vi "AlliGator Settings Storage.vi"(6 "Get(F)/Set":bool, 7 "AlliGator Settings List":T1=enum."Source Image:Use Image Histogram for Contrast", 8 "Error In":errorcluster, 11 "Variant Data in":variant) -> (0 "Error Out":errorcluster, 3 "Variant Data out":variant)   [LabVIEW 2021, in "AlliGator Settings.lvlib"]
doc: "Get/Set Settings parameter values using variant attributes."
uses:
  AlliGator Settings.lvlib
  Phasor/Phasor Explorer Gate Parameters.ctl
  Phasor/Phasor Gate Type.ctl
  Phasor/Phasor Type of User-defined Function.ctl
  Phasor/Phasor Explorer Decay Parameters.ctl
  Phasor/Phasor IRF Model.ctl
  Phasor/Phasor Explorer Phasor Parameters.ctl
  Phasor/Phasor Calculation Type.ctl
  Phasor/Phasor SEPL Type.ctl
  Phasor/Phasor Explorer Display Parameters.ctl
  Phasor/Phasor Type of Series.ctl
  Image/Image Save File Format.ctl
  Phasor Plot/AlliGator Phasor Plot Size.ctl
  AlliGator Background Subtraction Parameters.ctl
  Graphs/XY Graph/XY Graph Plot Shift Parameters.ctl
  Graphs/XY Graph/XY Graph Plot Shift Method.ctl
  Fits/IRF(X)PSED/IRF(X)PSED Extraction Options.ctl
  Fits/IRF(X)PSED/Fourier Series Smoothing Option.ctl
  Fits/IRF(X)PSED/Fourier Series Truncation.ctl
  Fits/IRF(X)PSED/IRF Extraction Method.ctl
  AlliGator Settings List.ctl
  AlliGator Low Count Pixels Rejection Options.ctl
  Phasor/Phasor Ratio Type.ctl
  Decay Analysis/Decay Preprocessing/AlliGator Baseline Subtraction Method.ctl
  Fits/Decay Convolution/Decay Model.ctl
  Fits/Residual Type.ctl
  Fits/Non-linear Fitting Method v2.ctl
  Fits/Fit Calculation Method.ctl
  Fits/Non-linear Fitting Algorithm.ctl
  Fits/IRF(X)PSED/Decay Fit Parameters & Derived Quantities List v2.ctl
  Decay Analysis/Decay Fit/AlliGator Decay Fit Parameter Constraints 2.ctl
  Fits/IRF(X)PSED/Decay Fit Parameters In List.ctl
  Decay Analysis/IRF/AlliGator IRF Optimization Controls.ctl
  Decay Analysis/IRF/AlliGator IRF Deconvolution Metrics.ctl
  Math/Advanced Signal Processing Toolkit/Wavelet Analysis Options.ctl
  AlliGator High Count Pixels Rejection Options.ctl
  AlliGator Image Smoothing Options.ctl
  Arrays/Kernel Type.ctl
  Arrays/Smoothing Algorithm.ctl
  Fits/Square Pulse/Square Pulse Options.ctl
  Fits/Square Pulse/Square Pulse Levels Type.ctl
  Source Image/AlliGator Image Binning Options.ctl
  Phasor Plot/AlliGator Phasor Plot Smoothing Options.ctl
  AlliGator Phasor Plot Graphics Options.ctl
  AlliGator Exported Image Settings.ctl
  AlliGator Define Gates to.ctl
  AlliGator Gates to Keep.ctl
  Phasor Ratio/AlliGator Phasor Ratio Color-Coded Quantity.ctl
  Phasor/Phasor Calibration Type.ctl
  Histograms/Linear Histogram Options.ctl
  Histograms/Histogram Bin Option.ctl
  Histograms/Histogram Bin Position.ctl
  AlliGator Gate Arithmetic.ctl
  Phasor Ratio/AlliGator Phasor Reference Associated with Shortest Lifetime.ctl
  AlliGator Python Settings.ctl
  SwissSPAD/SwissSPAD Live_Image Display Options.ctl
  AlliGator Average Lifetime Options.ctl
  Phasor Calibration/AlliGator Calibration Map Algorithm.ctl
  Decay Analysis/Decay Fit/AlliGator Guess Parameters Options.ctl
  Phasor/Phasor Standard Deviation Options.ctl
  Source Image/AlliGator Source Image Scale Bar Options.ctl
  Fits/IRF(X)PSED/MLE Baseline Offset Type.ctl
  Image/Flatfield Correction Options.ctl
  Fits/Optimal Offset Selection Criterion.ctl
  Fits/IRF(X)PSED/Decay Fit Options v2.ctl
  Fits/IRF(X)PSED/Decay Fit Options v1.ctl
  Fits/Non-linear Fitting Method v1.ctl
  Graphs/XY Graph/XY Graph Plot Data.ctl
  Phasor/Phasor User-defined Gate & IRF.vi
  Graphs/XY Graph/XY Graph Add-Ons.lvlib
  Phasor/Phasor.lvlib
  Utilities/Utilities.lvlib
  Fits/Fits.lvlib
  Fits/IRF(X)PSED/Fit Weights Type.ctl
  Fits/IRF(X)PSED/Decay Fit Options v3.ctl
  Phasor Plot/AlliGator Phasor Plot.lvlib
  Image/Image.lvlib
  Decay Analysis/Decay Preprocessing/AlliGator Decay Preprocessing.lvlib
  Decay Analysis/Decay Fit/AlliGator Decay Fit.lvlib
  Decay Analysis/IRF/AlliGator IRF.lvlib
  Math/Math.lvlib
  Arrays/Arrays.lvlib
  Source Image/AlliGator Source Image.lvlib
  Phasor/Phasor Explorer.lvlib
  Phasor Ratio/AlliGator Phasor Ratio.lvlib
  Histograms/Histogram Window.lvlib
  SwissSPAD/SwissSPAD Live.lvlib
  Phasor Calibration/AlliGator Phasor Calibration.lvlib
  Fits/IRF(X)PSED/Fit Weights Type v2.ctl
  Fits/IRF(X)PSED/Decay Fit Options v4.ctl
panel:
  in  "Show Dead Left Columns Correction":bool
  in  "Tab Control":T2(tab)
  in  "Source ImageTab":T3(tab)
  in  "Use Image Histogram for Contrast":bool=TRUE
  in  "Low Count Pixels Rejection Options":T4={"Background Low Threshold Factor"=0.0, "Fixed Low Background Threshold"=20000.0, "Reject Low Count Pixels"=FALSE, "Low Percentile"=0.0} {"Low Percentile" min=0.0 max=100.0}
  in  "High Count Pixels Rejection Options":T5={"Background High Threshold Factor"=0.0, "Fixed High Background Threshold"=20000.0, "Reject High Count Pixels"=FALSE, "High Percentile"=100.0} {"High Percentile" min=0.0 max=100.0}
  in  "Hot Pixel Removal":T6 {"Percentile" min=0 max=100}
  in  "Dead Left Columns Correction":bool
  in  "Use Fixed ROI Diameter":bool
  in  "ROI Diameter":i32=12
  in  "ROI Center Color":u32(colorbox)=16711680
  in  "Image Binning Options":T7={"Use Image Binning"=FALSE, "X Bin"=1, "Y Bin"=1} {"Y Bin" min=1; "X Bin" min=1}
  in  "Flatfield Correction":T8={"Flatfield Estimation Options"={"Sampling Grid Size X"=256, "Sampling Grid Size Y"=256, "Polynomial Degree"=5}, "Background Options"={"Estimate Background"=TRUE, "Background Estimation Size"=32, "Niblack Deviation Factor [0. 1]"=0.2}, "Correction Factor"=1.1} {"Background Options"."Niblack Deviation Factor [0. 1]" min=0.0 max=1.0}
  in  "Image Smoothing Options":T9={"Use Image Smoothing"=FALSE, "Kernel Type"=enum."Bilinear", "Bin"=500, "Algorithm"=enum."Rapid"} {"Bin" min=1}
  in  "Peak Threshold":dbl=500.0
  in  "Intensity Threshold":dbl=500.0
  in  "Invert Binary Mask":bool
  in  "Image Pre-Processing Operations Order":string[](array[string]) caption="Order"
  in  "Median Overlay Color":u32(colorbox)
  in  "Overlay ROI Median":bool=TRUE caption="Use Image Brightness"
  in  "Image Resolution (Pixel Size)":dbl[unit]
  in  "Scale Bar Options":T12 caption="Scale Bar Options (*)"
  in  "Overlay Analyzed ROI Center":bool
  in  "Use Image Brightness":bool=TRUE
  in  "Blend Overlay with Image Background":bool=TRUE
  in  "Dataset Scaling Factor":dbl=1.0 caption="Scaling Factor" min=0.0
  in  "Gate Image Integration":dbl[unit]=3e-10 min=0.0 format="%#.3g"
  in  "Gate Image Exposure":dbl[unit]=3e-10 min=0.0 format="%#.3g"
  in  "Background File Subtraction":bool
  in  "Background Scaling Factor":dbl=1.0 caption="Scaling Factor"
  in  "Background File":path
  in  "Background Pile-up Correction":bool caption="Pile-up Correction"
  in  "Background Pixel Well Capacity":u32=1 caption="Max Value" min=1 step=1
  in  "Channel Arithmetic":T13
  in  "Available Gate Names":string[](array[string])
  in  "Channel Name":u16(ring) items=["Gate"]
  in  "Gates to Keep":T14 caption="Gates to Keep (*)"
  in  "Define Gates to":T15
  in  "Laser Period":dbl[unit] format="%#_3g"
  in  "Gates to Skip":T16
  in  "Gate Separation":dbl[unit]=4e-11
  in  "Gate Width":dbl[unit]=3e-10
  in  "Gate Step":i32=1 min=1
  in  "Pile-up Correction":bool
  in  "Pixel Well Capacity":i32=1 min=1
  in  "# Gates":u32=1 min=1 step=1
  in  "SYNC Period":dbl[unit] caption="IRF Period" min=0.0 format="%#_3g"
  in  "Mscrotime Gate Separation":dbl[unit]=1.0 min=0.0
  in  "Decay Tabs":T17(tab)
  in  "# Folds":u32=1 min=1
  in  "Fold Decay":bool caption="Straighten Decay"
  in  "Use Decay Pre-Processing":bool=TRUE
  in  "Head Fraction":dbl min=0.0 max=1.0
  in  "Use Cursors":bool
  in  "Use Periodicity":bool
  in  "Pixel-Normalize Decay":bool
  in  "Verbose Decay Pre-Processing":bool=TRUE caption="Verbose Devay Pre-Processing"
  in  "Straighten Decay":bool
  in  "Reverse Gates":bool caption="Revert Gates"
  in  "Additional Points":u32 caption="Gate Duration"
  in  "Tail Fraction":dbl caption="Gate Duration" min=0.0 max=1.0
  in  "Extrapolate Decay":bool
  in  "Baseline Subtraction Method":T18=enum."Min" caption="Method"
  in  "Background Definition Range":T19={"Min Gate"=0.0, "Max Gate"=8e-10}
  in  "Decay Shift Parameters":T20
  in  "Shift Decay":bool
  in  "Smoothen Decay":bool caption="Smooth Decay"
  in  "Smoothing Parameter":dbl caption="Gate Duration" min=0.0 max=1.0
  in  "1-Normalize Decay":bool
  in  "Background Subtraction":bool=TRUE
  in  "Constant Background":dbl=1.0
  in  "Decay Pre-Processing Operations Order":string[](array[string]) caption="Order"
  in  "[0-1]-Normalize Decay":bool caption="1- Normalize Decay"
  in  "Average Lifetime Options":T22={"Use Local IRF "=TRUE, "Use IRF Offset"=TRUE, "Use Fixed Offset"=TRUE, "Fixed Offset"=0.0, "Baseline %"=0.0} caption="Use Local IRF" {"Baseline %" min=0.0 max=100.0}
  in  "IRF Time Constants":dbl[](array[numeric])
  in  "IRF order":i32
  in  "Square Pulse Options":T23={"Method"=enum."Mode", "# Bins"=0, "Threshold %"=10.0, "Center on Midpoint"=FALSE, "Smoothen Plot"=FALSE} {"Threshold %" min=0.0 max=100.0}
  in  "Wavelet Analysis Options":T25={"Wavelet"=enum."db02", "Option for Approximate Coefficients"=enum."None", "# Levels"=1, "Threshold Settings"={"Thresholding Rule"=enum."Universal", "Rescaling Method"=enum."Single level", "Soft Threshold?"=TRUE}, "Wavelet Transform Type"=enum."Discrete"}
  in  "Time Constant for IRF Extraction":T26={"Time Constant for IRF Extraction"=1e-18, "IRF Order"=1, "Fourier Series Smoothing"=enum."None", "Noise Threshold"=0.0, "Smoothing Width"=0.0, "Fourier Series Truncation"=enum."Automatic", "Truncation Order"=0, "Save Power Spectrum"=FALSE, "Smoothing"=FALSE, "Smoothing Parameter"=0.0, "Smoothing Order"=1, "Method"=enum."Direct"} caption="Gate Duration" {"Smoothing Order" min=1 max=10; "Time Constant for IRF Extraction" format="%#_5g"}
  in  "Extract IRF instead of Decay":bool
  in  "IRF Optimization Options":T30={"Search Range"=1e-18, "Search Step"=1e-09, "Tail Threshold (%)"=1e-09, "Regularized IRF"=FALSE, "Export Plot"=FALSE, "Export Data"=FALSE, "Smooth Metrics"=FALSE, "S-G Side Points"=1, "S-G Polynomial Order"=3, "Metrics"=enum."Average"} {"S-G Polynomial Order" min=3 max=10; "S-G Side Points" min=1; "Search Range" min=0.0 max=1e-09}
  in  "Use Data Information Laser Period":bool
  in  "Use Legagy Fitting Approach":bool
  in  "Fit Options":T32={"Show Fit Residuals"=TRUE, "Fit Model"=enum."1-Exponential", "Residual Type"=enum."Standard", "Max Decay Percentile"=0.0, "Min Decay Percentile"=0.0, "Show Full Decay"=TRUE, "Weights"=enum."Unweighted", "Fitting Method"=enum."Least Square", "Compute Parameter Uncertainties"=TRUE, "Periodic Boundaries"=TRUE, "Model Calculation"=enum."Simulation", "Period"=1.2500000000000001e-08, "Termination Criteria"={"Max Iterations"=1000, "Max Function Calls"=0, "Max Time"=1000.0, "Function Tolerance"=1e-06, "Parameter Tolerance"=1e-06, "Gradient Tolerance"=0.0, "Min Lambda"=1e-06, "Max Lambda"=1e-06, "Initial Tick Count"=0}, "Offset Resolution"=1.2500000000000001e-08, "Use Local IRF"=TRUE, "Fitting Algorithm"=enum."Levenberg-Marquardt", "Show Confidence Interval "=TRUE, "Confidence Level"=95.0} {"Confidence Level" min=0.0 max=100.0; "Offset Resolution" min=0.0; "Period" min=0.0; "Min Decay Percentile" min=0.0 max=1.0; "Max Decay Percentile" min=0.0 max=100.0}
  in  "Optimal Offset Selection Criterion":T39
  in  "MLE Baseline Offset Type":T40
  in  "MLE Baseline Offset":dbl
  in  "Guess Parameters Options":T41 caption="Options"
  in  "Guess Parameters Names":T42[](array[typedef])
  in  "Guess Parameter Values":dbl[](array[numeric]) caption="Guess Parameters"
  in  "Fit Parameter Constraints":T43[](array[typedef]) {"Max Value" format="%#.3g"; "Min Value" format="%#.3g"}
  in  "Displayed Fit Parameters":T44[](array[typedef])
  in  "Export Tabulated Results":bool=TRUE
  in  "Decay Graph Color Array":u32[](array[colorbox])
  in  "Show Last Decay only":bool
  in  "Max Peak Value":dbl
  in  "Reject High Decay Peak Pixels":bool
  in  "Min Peak Value":dbl
  in  "Reject Low Decay Peak Pixels":bool
  in  "Intensity Correction File":path
  in  "Use Intensity Correction File":bool
  in  "Use File Timestamp":bool
  in  "Time Step":dbl[unit]=1.0
  in  "Intensity-weighted Phasor Plot":bool caption="Cumulative Phasor Plot"
  in  "Low Color":u32(colorbox)
  in  "High Color":u32(colorbox)
  in  "User-defined Quantity":string
  in  "Blend Overlay with Phasor Background":bool=TRUE
  in  "Draw Reference Segment":bool
  in  "Store Phasor Harmonics":bool
  in  "All Phasor Plot ROIs":bool
  in  "Selected Phasor Plot ROI(s)":bool
  in  "Phasor Ratio Color-Coded Quantity":T45 caption="Displayed Quantity"
  in  "All Image ROIs":bool
  in  "Selected Image ROI(s)":bool
  in  "Reference Radius":i32=512
  in  "Phasor Ratio Display Range":cluster{dbl, dbl}(slide)={0.0, 454.0} scale=0.0..1.0
  in  "Phasor Plot Graphics Options":T46={"UC Color"=3381759, "Show UC Tau Ticks"=FALSE, "SEPL Color"=3381759, "Show SEPL Tau Ticks"=FALSE, "Axes Color"=16776960, "Show (g,s) Ticks"=FALSE, "Show UC"=FALSE, "Show SEPL"=FALSE, "Show Axes"=FALSE, "Show UC Tau Labels"=FALSE, "Show SEPL Tau Labels"=FALSE, "Show (g,s) Labels"=FALSE, "UC Label Size"=18, "UC Label Distance"=0.0, "SEPL Label Size"=18, "SEPL Label Distance"=0.0, "Axes Label Size"=18, "Axes Label Distance"=0.0}
  in  "Phasor Plot Smoothing Options":T47={"Use Phasor Plot Smoothing"=FALSE, "Kernel Type"=enum."Uniform", "Bin"=1, "Algorithm"=enum."Rapid"} {"Bin" min=1 step=2}
  in  "Phasor Ratio Color Map":string
  in  "Phasor Ratio Color Map Type":T48(radio)
  in  "Show Color Map Vertices":bool=TRUE
  in  "Exponential Fading":bool
  in  "Phasor Ratio Reference Colors":T49={"Reference 1"=3381759, "Reference 2"=3381759, "Boundary"=3381759}
  in  "Phasor Ratio Decay Range":dbl=1.0
  in  "Show References":bool
  in  "Save Phasor Plot":bool
  in  "Cumulative Phasor Plot":bool
  in  "Phasor Plot Size":T50={"H"=512, "V"=512, "Margin"=0.2} {"Margin" min=0.0}
  in  "Use Phasor Brightness":bool
  in  "Intensity-weighted Phasor Graph":bool
  in  "Phasor SDV Options":T51={"Compute Estimated SDV"=FALSE, "# Replicas"=100, "Use Estimated Average Phasor"=FALSE}
  in  "Define Shortest Lifetime as":T52
  in  "Save Phasor Graph Image":bool
  in  "Pixel-level Phasor Computation":bool
  in  "Phasor Ratio Type":T53
  in  "Phasor Frequency":dbl[unit]=160000000.0
  in  "Phasor Graph Active":bool caption="Save Phasor Graph Image"
  in  "SEPL Tabs":enum32{"Display", "Phasor", "IRF", "Gates"}(tab)
  in  "SEPL Display Parameters":T54={"# Points"=1000, "Ramp Type"=enum."Logarithmic", "Type of Series"=enum."1-Exp Decays", "Min tau"=1.0000000000000002e-12, "Max tau"=1.0000000000000001e-07, "Include 0"=FALSE, "Include Infinity"=FALSE} {"Min tau" min=0.0; "Max tau" min=0.0; "# Points" min=1 step=1}
  in  "SEPL Phasor Parameters":T56={"Harmonic Frequency"=0.0, "Use f* = 1/D Frequency"=FALSE, "Calibrated Phasor"=FALSE, "Calibration Lifetime"=1e-09, "Phasor Calculation"=enum."Direct Sum", "SEPL Type"=enum."UC", "# Gates"=1.0, "Square Gate Width"=1e-09, "Show Ticks"=FALSE} {"Square Gate Width" min=0.0; "# Gates" min=0.0; "Calibration Lifetime" min=0.0; "Harmonic Frequency" min=0.0}
  in  "SEPL IRF Parameters":T59={"Lifetime"=3.0000000000000004e-09, "IRF Offset"=0.0, "IRF Period"=1.2500000000000001e-08, "Normalized Decays"=FALSE, "IRF Model"=enum."Dirac", "IRF Parameter 1"=0.0} {"Lifetime" min=0.0; "IRF Period" min=0.0}
  in  "SEPL Gate Parameters":T61={"First Gate Start"=0.0, "Use Gate Center"=FALSE, "Gate Width"=0.0, "Gate Step"=0.0, "# Gates"=1.0, "Gate Type"=enum."Square", "Edge Width"=0.0, "Top Slope"=0.0, "Reversed Sawtooth?"=FALSE, "Analytical Computation"=FALSE, "Integration"=enum."Item 0", "Tolerance"=1.0, "# Steps"=1.0, "Type of User-defined Function"=enum."Gate", "Use Gate Step"=FALSE} {"# Steps" min=0.0; "Tolerance" min=0.0; "Top Slope" min=0.0; "Edge Width" min=0.0; "Gate Step" min=0.0; "# Gates" min=1.0 step=1.0; "Gate Width" min=0.0}
  in  "Calibration Map Algorithm":T64
  in  "Calibration Type":T65=enum."Single Phasor"
  in  "Use Backup Calibration if needed":bool=TRUE
  in  "Backup Calibration Type":T66(ring) caption="Backup Calibration"
  in  "Calibration Lifetime":dbl[unit]=1e-09
  in  "Decay Analysis Parameters":T20
  in  "Python Settings":T67
  in  "Transparent Mask Color":u32(colorbox)
  in  "ROI Description Max Characters":i32=256
  in  "Beep on Error":bool caption="Verbose Error Mode"
  in  "# Logical Processors Used":i32 caption="Used" min=1 max=16
  in  "Histogram Options":T68={"Bin Size"=0.0, "Bin Number"=0, "Bin Option"=enum."Bin Number", "Min Value"=-inf, "Max Value"=inf, "Filter NaN & Infinite Values"=TRUE, "Frequency Plot"=FALSE, "Align Bins"=FALSE, "Bin Location"=enum."Left", "Project Outside Values"=FALSE, "Max Histogram Size"=100000} {"Max Histogram Size" format="%.0e"}
  in  "Exported Gate Image Settings":T71
  in  "Verbose Error Mode":bool
  in  "Verbose Settings Mode":bool
  in  "Beep after Script":bool
  in  "Verbose Mode":bool
  in  "Saved Displayed Image File Format":T72
  in  "Visible Settings Tab":string caption="Settings Tab List"
  in  "Include Loading in Timing":bool
  in  "Last Run Version":string
  # "see the AlliGator License on the block diagram (Ctrl+E or Window:Show Block Diagram)"
  # "Gates Characteristics"
  # "Limit Phasor Plot Analysis  to:"
  # "Lifetime Analysis Options"
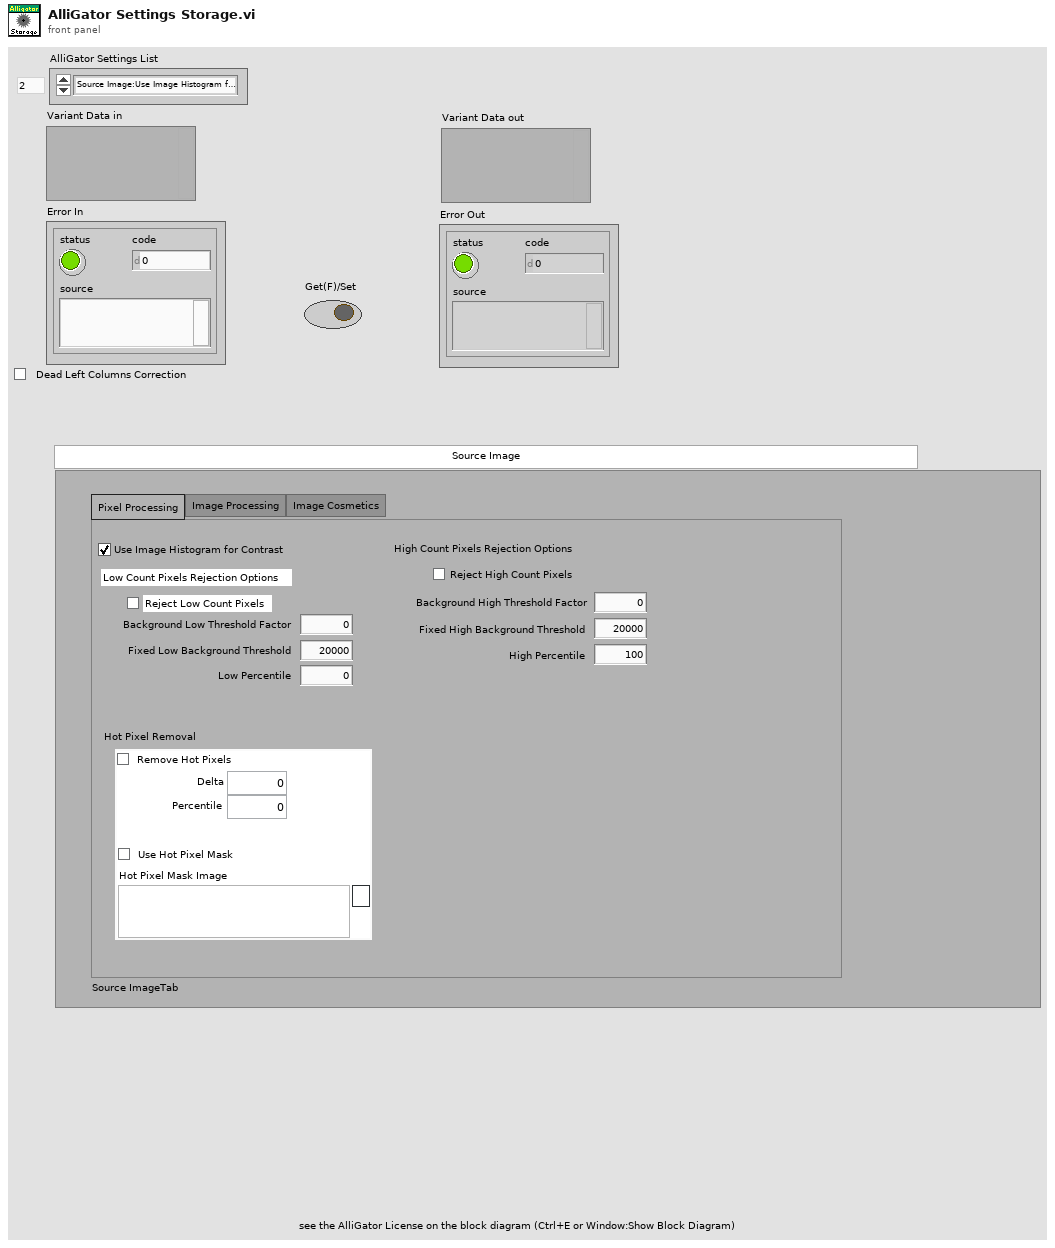
[diagram p1: front panel]
types:
  T1 = typedef "AlliGator Settings.lvlib/AlliGator Settings List.ctl" = enum16{"GUI:Visible Settings Tab", "GUI:Last Run Version", "Source Image:Use Image Histogram for Contrast", "Source Image:Low Count Pixels Rejection Options", "Source Image:High Count Pixels Rejection Options", "Source Image:Use Image Brightness", "Source Image:Blend Overlay with Image Background", "Source Image:Use Fixed ROI Diameter", "Source Image:ROI Diameter", "Source Image:ROI Center Color", "Source Image:Peak Threshold", "Source Image:Intensity Threshold", "Source Image:Image Binning Options", "Source Image:Image Smoothing Options", "Source Image:Image Histogram Active", "Source Image:Invert Binary Mask", "Source Image:Hot Pixel Removal", "Source Image:Overlay Analyzed ROI Center", "Source Image:Auto-Adjust Contrast", "Source Image:Histogram Lower Percentile", "Source Image:Histogram Upper Percentile", "Source Image:Save Source Image", "Source Image:Scale Bar Options", "Source Image:Image Resolution (Pixel Size)", "Source Image:Flatfield Correction", "Source Image:Show Dead Left Columns Correction", "Source Image:Dead Left Columns Correction", "Source Image:Image Pre-Processing Operations Order", "Source Image:Overlay ROI Median", "Source Image:Median Overlay Color", "Data Information:Gate Width", "Data Information:Nanotime Gate Separation", "Data Information:Macrotime Gate Separation", "Data Information:Gate Step", "Data Information:# Gates", "Data Information:Gate Image Exposure", "Data Information:Gate Image Integration", "Data Information:Gates to Skip", "Data Information:Gates to Keep", "Data Information:Define Gates to", "Data Information:Channel Name", "Data Information:Available Channel Names", "Data Information:Channel Arithmetic", "Data Information:Background File Subtraction", "Data Information:Background File", "Data Information:Background Scaling Factor", "Data Information:Background Pile-up Correction", "Data Information:Background Pixel Well Capacity", "Data Information:Laser Period", "Data Information:SYNC Period", "Data Information:Pile-up Correction", "Data Information:Pixel Well Capacity", "Data Information:Dataset Scaling Factor", "Fluorescence Decay_Decay Pre-Processing:Reverse Gates", "Fluorescence Decay_Decay Pre-Processing:Verbose Decay Pre-Processing", "Fluorescence Decay_Decay Pre-Processing:Use Decay Pre-Processing", "Fluorescence Decay_Decay Pre-Processing:Background Subtraction", "Fluorescence Decay_Decay Pre-Processing:Background Definition Range", "Fluorescence Decay_Decay Pre-Processing:Baseline Subtraction Method", "Fluorescence Decay_Decay Pre-Processing:Decay Pre-Processing Operations Order", "Fluorescence Decay_Decay Pre-Processing:Smoothing Parameter", "Fluorescence Decay_Decay Pre-Processing:Shift Decay", "Fluorescence Decay_Decay Pre-Processing:Decay Shift Parameters", "Fluorescence Decay_Decay Pre-Processing:Fold Decay", "Fluorescence Decay_Decay Pre-Processing:# Folds", "Fluorescence Decay_Decay Pre-Processing:1-Normalize Decay", "Fluorescence Decay_Decay Pre-Processing:[0-1]-Normalize Decay", "Fluorescence Decay_Decay Pre-Processing:Smoothen Decay", "Fluorescence Decay_Decay Pre-Processing:Extrapolate Decay", "Fluorescence Decay_Decay Pre-Processing:Use Periodicity", "Fluorescence Decay_Decay Pre-Processing:Use Cursors", "Fluorescence Decay_Decay Pre-Processing:Tail Fraction", "Fluorescence Decay_Decay Pre-Processing:Head Fraction", "Fluorescence Decay_Decay Pre-Processing:Additional Points", "Fluorescence Decay_Decay Pre-Processing:Straighten Decay", "Fluorescence Decay_Decay Pre-Processing:Constant Background", "Fluorescence Decay_Decay Pre-Processing:Pixel-Normalize Decay", "Fluorescence Decay_Advanced Analysis:Extract IRF instead of Decay", "Fluorescence Decay_Advanced Analysis:IRF Extraction Options", "Fluorescence Decay_Advanced Analysis:IRF Optimization Options", "Fluorescence Decay_Advanced Analysis:Square Pulse Options", "Fluorescence Decay_Advanced Analysis:IRF Order", "Fluorescence Decay_Advanced Analysis:IRF Time Constants", "Fluorescence Decay_Advanced Analysis:Wavelet Analysis Options", "Fluorescence Decay_Advanced Analysis:Average Lifetime Options", "Fluorescence Decay_Fit Options:Fit Options", "Fluorescence Decay_Fit Options:Use Legacy Fitting Approach", "Fluorescence Decay_Fit Options:Use Data Information Laser Period", "Fluorescence Decay_Fit Parameters:Displayed Fit Parameters", "Fluorescence Decay_Fit Parameters:Fit Parameter Constraints", "Fluorescence Decay_Fit Parameters:Export Tabulated Results", "Fluorescence Decay_Fit Parameters:MLE Baseline Offset Type", "Fluorescence Decay_Fit Parameters:MLE Baseline Offset", "Fluorescence Decay_Fit Parameters:Guess Parameter Names", "Fluorescence Decay_Fit Parameters:Guess Parameter Values", "Fluorescence Decay_Fit Parameters:Guess Parameters Options", "Fluorescence Decay_Fit Parameters:Optimal Offset Selection Criterion", "Fluorescence Decay_Styles:Show Last Decay Only", "Fluorescence Decay_Styles:Decay Graph Color Array", "Fluorescence Decay:Decay Graph Active", "Fluorescence Decay Statistics:Min Peak Value", "Fluorescence Decay Statistics:Reject Low Decay Peak Pixels", "Fluorescence Decay Statistics:Reject High Decay Peak Pixels", "Fluorescence Decay Statistics:Max Peak Value", "Time Traces:Use File Timestamp", "Time Traces:Time Step", "Time Traces:Use Intensity Correction File", "Time Traces:Intensity Correction File", "Phasor Plot:Phasor Plot Smoothing Options", "Phasor Plot:Phasor Plot Size", "Phasor Plot:Phasor Plot Graphics Options", "Phasor Plot:Cumulative Phasor Plot", "Phasor Plot:Use Phasor Brightness", "Phasor Plot:Blend Overlay with Phasor Background", "Phasor Plot:Save Phasor Plot", "Phasor Plot:Show References", "Phasor Plot:Phasor Ratio Decay Range", "Phasor Plot:Exponential Fading", "Phasor Plot:Phasor Ratio Reference Colors", "Phasor Plot:Reference Radius", "Phasor Plot:Show Color Map Vertices", "Phasor Plot:Phasor Plot Active", "Phasor Plot:Phasor Ratio Color Map Type", "Phasor Plot:Phasor Ratio Color Map", "Phasor Plot:Phasor Ratio Display Range", "Phasor Plot:Selected Image ROI(s)", "Phasor Plot:All Image ROIs", "Phasor Plot:Selected Phasor Plot ROI(s)", "Phasor Plot:All Phasor Plot ROIs", "Phasor Plot:Phasor Ratio Color-Coded Quantity", "Phasor Plot:Store Phasor Harmonics", "Phasor Plot:Draw Reference Segment", "Phasor Plot:User-Defined Quantity", "Phasor Plot:Color Scale High Color", "Phasor Plot:Color Scale Low Color", "Phasor Plot:Intensity-weighted Phasor Plot", "Phasor Graph:Phasor Frequency", "Phasor Graph:Phasor Ratio Type", "Phasor Graph:Pixel-level Phasor Computation", "Phasor Graph:Save Phasor Graph", "Phasor Graph:Phasor Graph Active", "Phasor Graph:Phasor SDV Options", "Phasor Graph:Intensity-weighted Phasor Graph", "Phasor Graph:Define Shortest Lifetime as", "Phasor Calibration:Use Backup Calibration if needed", "Phasor Calibration:Backup Calibration Type", "Phasor Calibration:Calibration Type", "Phasor Calibration:Calibration Lifetime", "Phasor Calibration:Calibration Map Algorithm", "Single-Exponential Phasor Locus (SEPL):Gate Parameters", "Single-Exponential Phasor Locus (SEPL):User-defined Gate", "Single-Exponential Phasor Locus (SEPL):User-defined IRF", "Single-Exponential Phasor Locus (SEPL):Phasor Parameters", "Single-Exponential Phasor Locus (SEPL):Decay & IRF Parameters", "Single-Exponential Phasor Locus (SEPL):Display Parameters", "Lifetime Analysis:Decay Analysis Parameters", "Lifetime Analysis:Lifetime Map Active", "Plugins:Python Settings", "Miscellaneous:Verbose Mode", "Miscellaneous:Beep after Script", "Miscellaneous:Saved Image File Format", "Miscellaneous:Exported Gate Image Settings", "Miscellaneous:Include Loading in Timing", "Miscellaneous:Verbose Settings Mode", "Miscellaneous:Histogram Options", "Miscellaneous:Beep on Error", "Miscellaneous:# Logical Processors Used", "Miscellaneous:ROI Description Max Characters", "Miscellaneous:Verbose Error Mode", "Miscellaneous:Transparent Mask Color"}
  T2 = enum32{"Source Image", "Data Information", "Fluorescence Decay", "Fluorescence Decay Statistics", "Time Traces", "Phasor Plot", "Phasor Graph", "Single-Exponential Phasor Locus (SEPL)", "Phasor Calibration", "Lifetime Analysis", "Plugins", "Miscellaneous"}
  T3 = enum32{"Pixel Processing", "Image Processing", "Image Cosmetics"}
  T4 = typedef "AlliGator Settings.lvlib/AlliGator Low Count Pixels Rejection Options.ctl" = cluster{"Background Low Threshold Factor":dbl, "Fixed Low Background Threshold":dbl, "Reject Low Count Pixels":bool, "Low Percentile":dbl}
  T5 = typedef "AlliGator Settings.lvlib/AlliGator High Count Pixels Rejection Options.ctl" = cluster{"Background High Threshold Factor":dbl, "Fixed High Background Threshold":dbl, "Reject High Count Pixels":bool, "High Percentile":dbl}
  T6 = typedef "SwissSPAD Live.lvlib/SwissSPAD Live_Image Display Options.ctl" = cluster{"Remove Screamers":bool, "Delta":sgl, "Equalize Histogram":bool, "Percentile":sgl, "Hot Pixel Mask Image":path, "Use Hot Pixel Mask":bool}
  T7 = typedef "AlliGator Source Image.lvlib/AlliGator Image Binning Options.ctl" = cluster{"Use Image Binning":bool, "X Bin":i32, "Y Bin":i32}
  T8 = typedef "Image.lvlib/Flatfield Correction Options.ctl" = cluster{"Flatfield Estimation Options":cluster{"Sampling Grid Size X":i32, "Sampling Grid Size Y":i32, "Polynomial Degree":i32}, "Background Options":cluster{"Estimate Background":bool, "Background Estimation Size":i32, "Niblack Deviation Factor [0. 1]":dbl}, "Correction Factor":sgl}
  T9 = typedef "AlliGator Settings.lvlib/AlliGator Image Smoothing Options.ctl" = cluster{"Use Image Smoothing":bool, "Kernel Type":T10, "Bin":i32, "Algorithm":T11}
  T10 = typedef "Arrays.lvlib/Kernel Type.ctl" = enum16{"Uniform", "Bilinear", "Gaussian"}
  T11 = typedef "Arrays.lvlib/Smoothing Algorithm.ctl" = enum16{"Rapid", "Thorough"}
  T12 = typedef "AlliGator Source Image.lvlib/AlliGator Source Image Scale Bar Options.ctl" = cluster{"Show Scale Bar Overlay":bool, "Scale Bar Length":dbl[unit], "Scale Bar Color":u32, "Scale Bar X":u32, "Scale Bar Y":u32, "Scale Bar Height":dbl[unit]}
  T13 = typedef "AlliGator Settings.lvlib/AlliGator Gate Arithmetic.ctl" = enum16{"None", "INT-G2", "G2/INT*<INT>", "(1 - G2/INT)*<INT>"}
  T14 = typedef "AlliGator Settings.lvlib/AlliGator Gates to Keep.ctl" = cluster{"First":u32, "Last":u32}
  T15 = typedef "AlliGator Settings.lvlib/AlliGator Define Gates to.ctl" = enum32{"Skip", "Keep"}
  T16 = typedef "AlliGator Settings.lvlib/AlliGator Background Subtraction Parameters.ctl" = cluster{"Start":u32, "End":u32}
  T17 = enum32{"Decay Pre-Processing", "Advanced Analysis", "Fit Options", "Fit Parameters", "Styles"}
  T18 = typedef "AlliGator Decay Preprocessing.lvlib/AlliGator Baseline Subtraction Method.ctl" = enum16{"Mean", "Min", "Square Gated Single-Exponential", "File", "Constant"}
  T19 = cluster{"Min Gate":dbl[unit], "Max Gate":dbl[unit]}
  T20 = typedef "XY Graph Add-Ons.lvlib/XY Graph Plot Shift Parameters.ctl" = cluster{"Type":T21, "Shift":dbl[unit], "Threshold":dbl, "Rotate":bool}
  T21 = typedef "XY Graph Add-Ons.lvlib/XY Graph Plot Shift Method.ctl" = enum16{"Default", "CFD", "Threshold", "Cross-Correlation"}
  T22 = typedef "AlliGator Settings.lvlib/AlliGator Average Lifetime Options.ctl" = cluster{"Use Local IRF ":bool, "Use IRF Offset":bool, "Use Fixed Offset":bool, "Fixed Offset":dbl[unit], "Baseline %":dbl}
  T23 = typedef "Fits.lvlib/Square Pulse Options.ctl" = cluster{"Method":T24, "# Bins":i32, "Threshold %":dbl, "Center on Midpoint":bool, "Smoothen Plot":bool}
  T24 = typedef "Fits.lvlib/Square Pulse Levels Type.ctl" = enum16{"Mode", "Mean"}
  T25 = typedef "Math.lvlib/Wavelet Analysis Options.ctl" = cluster{"Wavelet":enum16{"db02", "db03", "db04", "db05", "db06", "db07", "db08", "db09", "db10", "db11", "db12", "db13", "db14", "Haar", "bior1_3", "bior1_5", "bior2_2", "bior2_4", "bior2_6", "bior2_8", "bior3_1", "bior3_3", "bior3_5", "bior3_7", "bior3_9", "bior4_4 (FBI)", "bior5_5", "bior6_8", "coif1", "coif2", "coif3", "coif4", "coif5", "sym2", "sym3", "sym4", "sym5", "sym6", "sym7", "sym8"}, "Option for Approximate Coefficients":enum16{"None", "Threshold", "Detrend"}, "# Levels":i32, "Threshold Settings":cluster{"Thresholding Rule":enum16{"SURE", "Hybrid", "Universal", "Minimax"}, "Rescaling Method":enum16{"One", "Single level", "Multiple levels"}, "Soft Threshold?":bool}, "Wavelet Transform Type":enum16{"Discrete", "Undecimated"}}
  T26 = typedef "Fits.lvlib/IRF(X)PSED Extraction Options.ctl" = cluster{"Time Constant for IRF Extraction":dbl[unit], "IRF Order":i32, "Fourier Series Smoothing":T27, "Noise Threshold":dbl, "Smoothing Width":dbl, "Fourier Series Truncation":T28, "Truncation Order":i32, "Save Power Spectrum":bool, "Smoothing":bool, "Smoothing Parameter":dbl, "Smoothing Order":u32, "Method":T29}
  T27 = typedef "Fits.lvlib/Fourier Series Smoothing Option.ctl" = enum16{"None", "Lanczos Factors", "Fejer Summation"}
  T28 = typedef "Fits.lvlib/Fourier Series Truncation.ctl" = enum16{"Automatic", "Fixed"}
  T29 = typedef "Fits.lvlib/IRF Extraction Method.ctl" = enum16{"Direct", "Topless", "Toeplitz"}
  T30 = typedef "AlliGator IRF.lvlib/AlliGator IRF Optimization Controls.ctl" = cluster{"Search Range":dbl[unit], "Search Step":dbl[unit], "Tail Threshold (%)":dbl, "Regularized IRF":bool, "Export Plot":bool, "Export Data":bool, "Smooth Metrics":bool, "S-G Side Points":i32, "S-G Polynomial Order":i32, "Metrics":T31}
  T31 = typedef "AlliGator IRF.lvlib/AlliGator IRF Deconvolution Metrics.ctl" = enum16{"Average", "SDV", "Max", "Average * SDV", "Slope"}
  T32 = typedef "Fits.lvlib/Decay Fit Options v4.ctl" = cluster{"Show Fit Residuals":bool, "Fit Model":T33, "Residual Type":T34, "Max Decay Percentile":dbl, "Min Decay Percentile":dbl, "Show Full Decay":bool, "Weights":T35, "Fitting Method":T36, "Compute Parameter Uncertainties":bool, "Periodic Boundaries":bool, "Model Calculation":T37, "Period":dbl[unit], "Termination Criteria":cluster{"Max Iterations":i32, "Max Function Calls":i32, "Max Time":dbl[unit], "Function Tolerance":dbl, "Parameter Tolerance":dbl, "Gradient Tolerance":dbl, "Min Lambda":dbl, "Max Lambda":dbl, "Initial Tick Count":u32}, "Offset Resolution":dbl[unit], "Use Local IRF":bool, "Fitting Algorithm":T38, "Show Confidence Interval ":bool, "Confidence Level":dbl}
  T33 = typedef "Fits.lvlib/Decay Model.ctl" = enum16{"1-Exponential", "2-Exponentials"}
  T34 = typedef "Fits.lvlib/Residual Type.ctl" = enum16{"Standard", "Normalized", "Reduced"}
  T35 = typedef "Fits.lvlib/Fit Weights Type v2.ctl" = enum16{"Unweighted", "1/Variance (Neyman)", "1/Variance (Pearson)", "Best of All"}
  T36 = typedef "Fits.lvlib/Non-linear Fitting Method v2.ctl" = enum16{"Least Square", "Least Absolute Residual", "Bisquare", "MLE", "-", "Best of All"}
  T37 = typedef "Fits.lvlib/Fit Calculation Method.ctl" = enum16{"Simulation", "Convolution", "Integration"}
  T38 = typedef "Fits.lvlib/Non-linear Fitting Algorithm.ctl" = enum16{"Levenberg-Marquardt", "Trust-Region Dogleg"}
  T39 = typedef "Fits.lvlib/Optimal Offset Selection Criterion.ctl" = enum16{"Min Chi^2", "Max R^2"}
  T40 = typedef "Fits.lvlib/MLE Baseline Offset Type.ctl" = enum32{"Absolute", "Percentage"}
  T41 = typedef "AlliGator Decay Fit.lvlib/AlliGator Guess Parameters Options.ctl" = enum16{"Numerically estimated", "User-provided", "User-provided (normalized)", "Last valid fitted parameters"}
  T42 = typedef "Fits.lvlib/Decay Fit Parameters In List.ctl" = enum16{"Offset", "Baseline", "A_1", "tau_1", "A_2", "tau_2"}
  T43 = typedef "AlliGator Decay Fit.lvlib/AlliGator Decay Fit Parameter Constraints 2.ctl" = cluster{"Fit Parameter":T42, "Min Value":dbl, "Max Value":dbl, "Global":bool, "Used":bool}
  T44 = typedef "Fits.lvlib/Decay Fit Parameters & Derived Quantities List v2.ctl" = enum16{"Offset", "Baseline", "A_1", "tau_1", "A_2", "tau_2", "<tau>_a", "f1_a", "f2_a", "<tau>_i", "f1_i", "f2_i", "-", "R^2", "Chi^2"}
  T45 = typedef "AlliGator Phasor Ratio.lvlib/AlliGator Phasor Ratio Color-Coded Quantity.ctl" = enum16{"Phasor Ratio (f1 or a1)", "Average Lifetime (<tau>_i or <tau>_a))", "User-Defined Quantity"}
  T46 = typedef "AlliGator Settings.lvlib/AlliGator Phasor Plot Graphics Options.ctl" = cluster{"UC Color":u32, "Show UC Tau Ticks":bool, "SEPL Color":u32, "Show SEPL Tau Ticks":bool, "Axes Color":u32, "Show (g,s) Ticks":bool, "Show UC":bool, "Show SEPL":bool, "Show Axes":bool, "Show UC Tau Labels":bool, "Show SEPL Tau Labels":bool, "Show (g,s) Labels":bool, "UC Label Size":i16, "UC Label Distance":dbl, "SEPL Label Size":i16, "SEPL Label Distance":dbl, "Axes Label Size":i16, "Axes Label Distance":dbl}
  T47 = typedef "AlliGator Phasor Plot.lvlib/AlliGator Phasor Plot Smoothing Options.ctl" = cluster{"Use Phasor Plot Smoothing":bool, "Kernel Type":T10, "Bin":i32, "Algorithm":T11}
  T48 = enum32{"Interpolate Reference Colors", "Use Custom Map"}
  T49 = cluster{"Reference 1":u32, "Reference 2":u32, "Boundary":u32}
  T50 = typedef "AlliGator Phasor Plot.lvlib/AlliGator Phasor Plot Size.ctl" = cluster{"H":i32, "V":i32, "Margin":dbl}
  T51 = typedef "Phasor.lvlib/Phasor Standard Deviation Options.ctl" = cluster{"Compute Estimated SDV":bool, "# Replicas":u32, "Use Estimated Average Phasor":bool}
  T52 = typedef "AlliGator Phasor Ratio.lvlib/AlliGator Phasor Reference Associated with Shortest Lifetime.ctl" = enum32{"Reference 1", "Reference 2"}
  T53 = typedef "Phasor.lvlib/Phasor Ratio Type.ctl" = enum32{"Intensity-weighted", "Amplitude-weighted"}
  T54 = typedef "Phasor Explorer.lvlib/Phasor Explorer Display Parameters.ctl" = cluster{"# Points":i32, "Ramp Type":enum16{"Linear", "Logarithmic"}, "Type of Series":T55, "Min tau":dbl[unit], "Max tau":dbl[unit], "Include 0":bool, "Include Infinity":bool}
  T55 = typedef "Phasor.lvlib/Phasor Type of Series.ctl" = enum16{"1-Exp Decays", "Linear Combination of 1-Exp"}
  T56 = typedef "Phasor Explorer.lvlib/Phasor Explorer Phasor Parameters.ctl" = cluster{"Harmonic Frequency":dbl[unit], "Use f* = 1/D Frequency":bool, "Calibrated Phasor":bool, "Calibration Lifetime":dbl[unit], "Phasor Calculation":T57, "SEPL Type":T58, "# Gates":dbl, "Square Gate Width":dbl[unit], "Show Ticks":bool}
  T57 = typedef "Phasor.lvlib/Phasor Calculation Type.ctl" = enum16{"Direct Sum", "Analytical Formula"}
  T58 = typedef "Phasor.lvlib/Phasor SEPL Type.ctl" = enum16{"UC", "L_N", "L_N[W]", "L_X"}
  T59 = typedef "Phasor Explorer.lvlib/Phasor Explorer Decay Parameters.ctl" = cluster{"Lifetime":dbl[unit], "IRF Offset":dbl[unit], "IRF Period":dbl[unit], "Normalized Decays":bool, "IRF Model":T60, "IRF Parameter 1":dbl[unit]}
  T60 = typedef "Phasor.lvlib/Phasor IRF Model.ctl" = enum16{"Dirac", "Exponential"}
  T61 = typedef "Phasor Explorer.lvlib/Phasor Explorer Gate Parameters.ctl" = cluster{"First Gate Start":dbl[unit], "Use Gate Center":bool, "Gate Width":dbl[unit], "Gate Step":dbl[unit], "# Gates":dbl, "Gate Type":T62, "Edge Width":dbl[unit], "Top Slope":dbl[unit], "Reversed Sawtooth?":bool, "Analytical Computation":bool, "Integration":enum32{"Item 0", "Item 1"}, "Tolerance":dbl, "# Steps":dbl, "Type of User-defined Function":T63, "Use Gate Step":bool}
  T62 = typedef "Phasor.lvlib/Phasor Gate Type.ctl" = enum16{"Square", "Finite Edge Square", "Finite Edge, Tilted Top Square", "Triangle", "Sawtooth", "User-defined"}
  T63 = typedef "Phasor.lvlib/Phasor Type of User-defined Function.ctl" = enum16{"Gate", "IRF"}
  T64 = typedef "AlliGator Phasor Calibration.lvlib/AlliGator Calibration Map Algorithm.ctl" = enum16{"Simple Search", "Min Distance"}
  T65 = typedef "Phasor.lvlib/Phasor Calibration Type.ctl" = enum16{"None", "Single Phasor", "Phasor Series", "Phasor Map"}
  T66 = enum16{"Single Calibration", "Nearest Valid Calibration"}
  T67 = typedef "AlliGator Settings.lvlib/AlliGator Python Settings.ctl" = cluster{"Python Version":string, "Use PATH definition":bool, "Python.exe Path":path, "Include Example Plugins":bool}
  T68 = typedef "Histogram Window.lvlib/Linear Histogram Options.ctl" = cluster{"Bin Size":dbl, "Bin Number":i32, "Bin Option":T69, "Min Value":dbl, "Max Value":dbl, "Filter NaN & Infinite Values":bool, "Frequency Plot":bool, "Align Bins":bool, "Bin Location":T70, "Project Outside Values":bool, "Max Histogram Size":i32}
  T69 = typedef "Histogram Window.lvlib/Histogram Bin Option.ctl" = enum32{"Bin Number", "Bin Size"}
  T70 = typedef "Histogram Window.lvlib/Histogram Bin Position.ctl" = enum16{"Left", "Center", "Right"}
  T71 = typedef "AlliGator Settings.lvlib/AlliGator Exported Image Settings.ctl" = cluster{"bitness":bool, " Min Value":sgl, " Max Value":sgl}
  T72 = typedef "Image.lvlib/Image Save File Format.ctl" = enum16{"PNG", "JPEG", "BMP"}
  T73 = typedef "Fits.lvlib/Decay Fit Options v3.ctl" = cluster{"Show Fit Residuals":bool, "Fit Model":T33, "Residual Type":T34, "Max Decay Percentile":dbl, "Min Decay Percentile":dbl, "Show Full Decay":bool, "Weights":T74, "Fitting Method":T36, "Compute Parameter Uncertainties":bool, "Periodic Boundaries":bool, "Model Calculation":T37, "Period":dbl[unit], "Termination Criteria":cluster{"Max Iterations":i32, "Max Function Calls":i32, "Max Time":dbl[unit], "Function Tolerance":dbl, "Parameter Tolerance":dbl, "Gradient Tolerance":dbl, "Min Lambda":dbl, "Max Lambda":dbl, "Initial Tick Count":u32}, "Offset Resolution":dbl[unit], "Use Local IRF":bool, "Fitting Algorithm":T38, "Show Confidence Interval ":bool, "Confidence Level":dbl}
  T74 = typedef "Fits.lvlib/Fit Weights Type.ctl" = enum16{"Unweighted", "1/Variance", "Best of All"}
  T75 = typedef "Fits.lvlib/Decay Fit Options v2.ctl" = cluster{"Show Fit Residuals":bool, "Fit Model":T33, "Residual Type":T34, "Max Decay Percentile":dbl, "Min Decay Percentile":dbl, "Show Full Decay":bool, "Weights":T74, "Fitting Method":T36, "Compute Parameter Uncertainties":bool, "Periodic Boundaries":bool, "Model Calculation":T37, "Period":dbl[unit], "Termination Criteria":cluster{"Max Iterations":i32, "Max Function Calls":i32, "Max Time":dbl[unit], "Function Tolerance":dbl, "Parameter Tolerance":dbl, "Gradient Tolerance":dbl, "Min Lambda":dbl, "Max Lambda":dbl, "Initial Tick Count":u32}, "Offset Resolution":dbl[unit], "Use Local IRF":bool, "Fitting Algorithm":T38}
  T76 = typedef "Fits.lvlib/Decay Fit Options v1.ctl" = cluster{"Show Fit Residuals":bool, "Fit Model":T33, "Residual Type":T34, "Max Decay Percentile":dbl, "Min Decay Percentile":dbl, "Show Full Decay":bool, "Weights":T74, "Fitting Method":T77, "Compute Parameter Uncertainties":bool, "Periodic Boundaries":bool, "Model Calculation":T37, "Period":dbl[unit], "Termination Criteria":cluster{"Max Iterations":i32, "Max Function Calls":i32, "Max Time":dbl[unit], "Function Tolerance":dbl, "Parameter Tolerance":dbl, "Gradient Tolerance":dbl, "Min Lambda":dbl, "Max Lambda":dbl, "Initial Tick Count":u32}, "Offset Resolution":dbl[unit], "Use Local IRF":bool, "Fitting Algorithm":T38}
  T77 = typedef "Fits.lvlib/Non-linear Fitting Method v1.ctl" = enum16{"Least Square", "Least Absolute Residual", "Bisquare", "-", "Best of All"}
  T78 = typedef "XY Graph Add-Ons.lvlib/XY Graph Plot Data.ctl" = cluster{"X Array":dbl[], "Y Array":dbl[]}
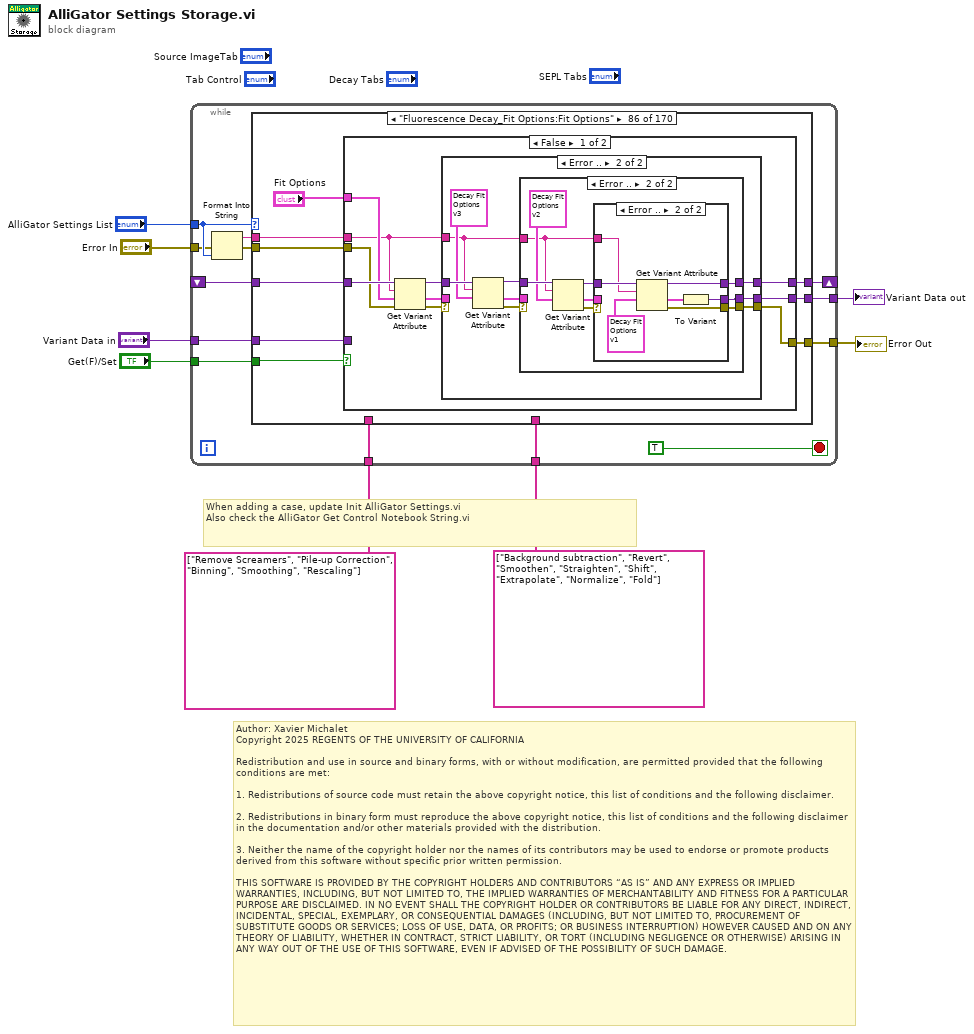
[diagram p0: block diagram]
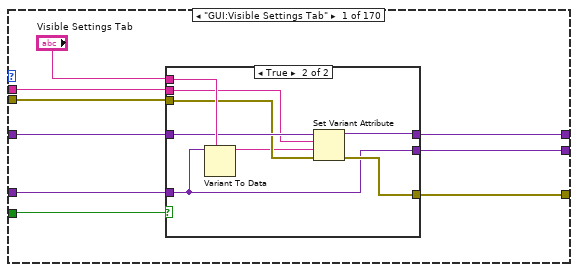
[diagram p2: hidden frame]
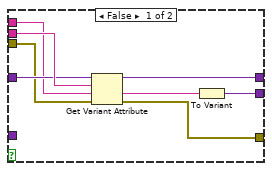
[diagram p3: hidden frame]
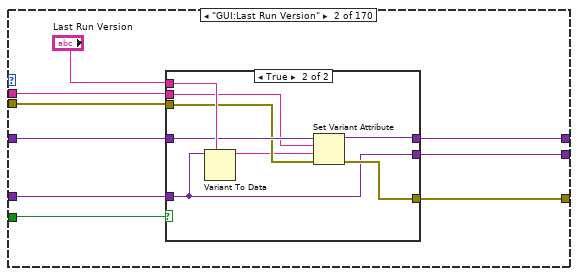
[diagram p4: hidden frame]
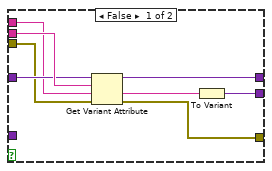
[diagram p5: hidden frame]
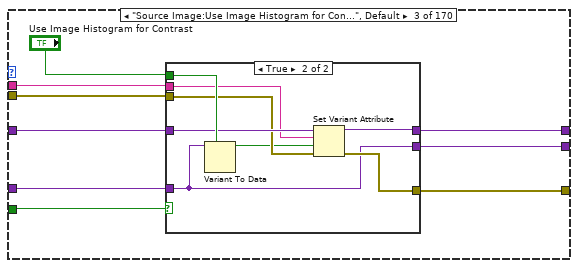
[diagram p6: hidden frame]
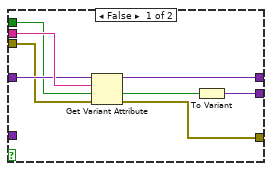
[diagram p7: hidden frame]
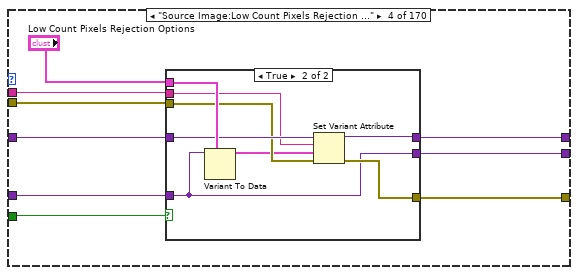
[diagram p8: hidden frame]
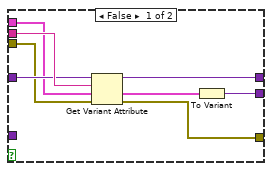
[diagram p9: hidden frame]
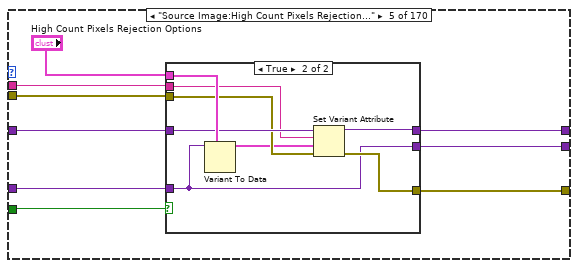
[diagram p10: hidden frame]
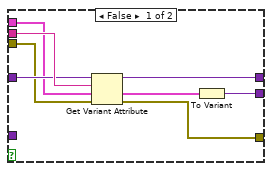
[diagram p11: hidden frame]
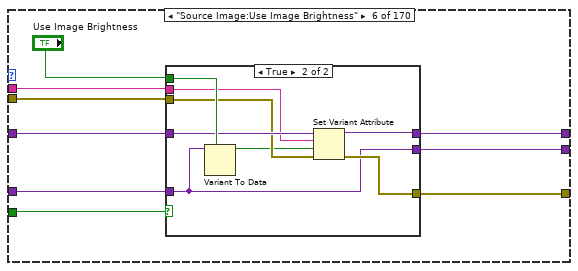
[diagram p12: hidden frame]
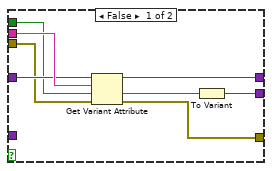
[diagram p13: hidden frame]
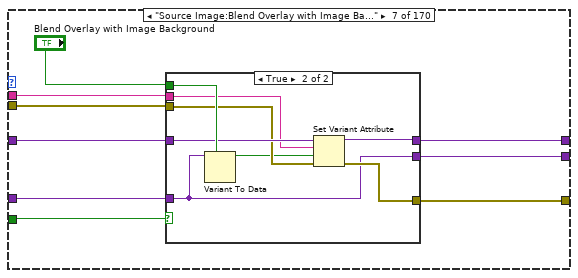
[diagram p14: hidden frame]
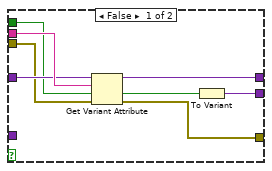
[diagram p15: hidden frame]
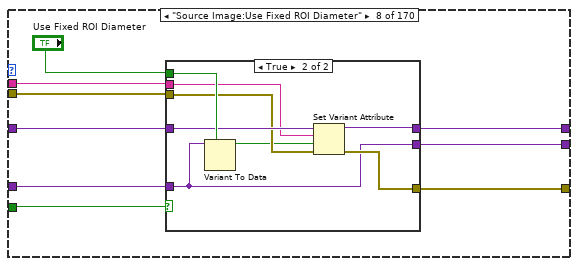
[diagram p16: hidden frame]
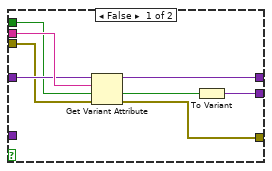
[diagram p17: hidden frame]
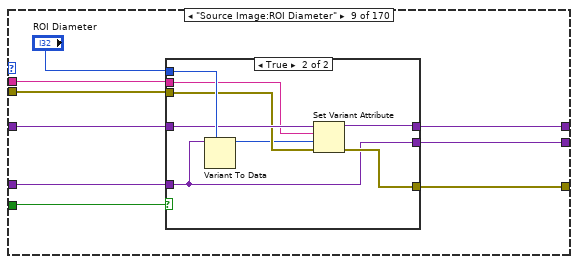
[diagram p18: hidden frame]
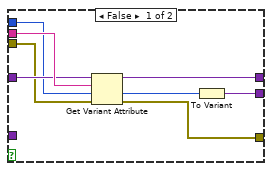
[diagram p19: hidden frame]
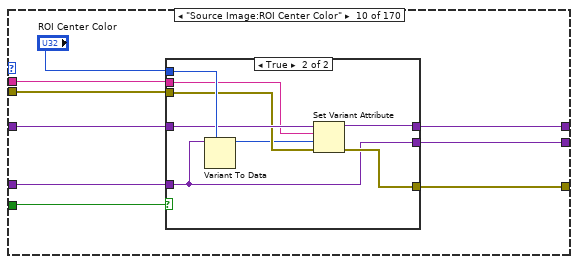
[diagram p20: hidden frame]
diagram:
  # "Author: Xavier Michalet\nCopyright 2025 REGENTS OF THE UNIVERSITY OF CALIFORNIA\n\nRedistribution and use in source and binary forms, with or without modification, are permitted provided that the following conditions are met:\n\n1. Redistributions of source code must retain the above copyright notice, this list of conditions and the following disclaimer.\n\n2. Redistributions in binary form must reproduce the above copyright notice, this list of conditions and the following disclaimer in the documentation and/or other materials provided with the distribution.\n\n3. Neither the name of the copyright holder nor the names of its contributors may be used to endorse or promote products derived from this software without specific prior written permission.\n\nTHIS SOFTWARE IS PROVIDED BY THE COPYRIGHT HOLDERS AND CONTRIBUTORS “AS IS” AND ANY EXPRESS OR IMPLIED WARRANTIES, INCLUDING, BUT NOT LIMITED TO, THE IMPLIED WARRANTIES OF MERCHANTABILITY AND FITNESS FOR A PARTICULAR PURPOSE ARE DISCLAIMED. IN NO EVENT SHALL THE COPYRIGHT HOLDER OR CONTRIBUTORS BE LIABLE FOR ANY DIRECT, INDIRECT, INCIDENTAL, SPECIAL, EXEMPLARY, OR CONSEQUENTIAL DAMAGES (INCLUDING, BUT NOT LIMITED TO, PROCUREMENT OF SUBSTITUTE GOODS OR SERVICES; LOSS OF USE, DATA, OR PROFITS; OR BUSINESS INTERRUPTION) HOWEVER CAUSED AND ON ANY THEORY OF LIABILITY, WHETHER IN CONTRACT, STRICT LIABILITY, OR TORT (INCLUDING NEGLIGENCE OR OTHERWISE) ARISING IN ANY WAY OUT OF THE USE OF THIS SOFTWARE, EVEN IF ADVISED OF THE POSSIBILITY OF SUCH DAMAGE."
  # "When adding a case, update Init AlliGator Settings.vi\nAlso check the AlliGator Get Control Notebook String.vi"
  n1 = while {
    tunnel: "AlliGator Settings List" -> [w21]
    tunnel: "Get(F)/Set" -> [w18]
    tunnel: "Variant Data in" -> [w17]
    tunnel: "Error In" -> [w16]
    shift-right: [w13] -> _
    shift-left: _ -> [w14]
    tunnel: [w12] -> w4
    tunnel: [w11] -> w3
    tunnel: string[] ["Background subtraction", "Revert", "Smoothen", "Straighten", "Shift", "Extrapolate", "Normalize", "Fold"] ("Operation Order") -> [w10]
    tunnel: string[] ["Remove Screamers", "Pile-up Correction", "Binning", "Smoothing", "Rescaling"] ("Operation Order") -> [w9]
    stop <- TRUE stop-if-true
    n2 = Format Into String(error in=w16, w21) -> (resulting string=w20:string, error out=w15:errorcluster)  [unwired: 2 in]
    n3 = case shown="\"Fluorescence Decay_Fit Options:Fit Options\"" w21 {
      tunnel: w20 -> [w29 w54 w79 w104 w129 w154 w179 w204 w229 w254 w279 w304 w329 w354 w379 w404 w429 w454 w479 w504 w529 w554 w579 w604 w629 w654 w679 w704 w729 w754 w779 w804 w829 w854 w879 w904 w929 w954 w979 w1004 w1029 w1054 w1079 w1104 w1129 w1154 w1179 w1204 w1229 w1254 w1279 w1304 w1329 w1354 w1379 w1404 w1429 w1454 w1480 w1511 w1541 w1566 w1591 w1616 w1641 w1666 w1691 w1716 w1741 w1766 w1791 w1816 w1841 w1866 w1891 w1916 w1941 w1966 w1991 w2016 w2041 w2066 w2091 w2118 w2143 w2168 w2232 w2257 w2282 w2307 w2332 w2357 w2382 w2407 w2432 w2457 w2482 w2507 w2532 w2557 w2582 w2607 w2632 w2657 w2682 w2707 w2732 w2757 w2782 w2807 w2832 w2857 w2882 w2907 w2932 w2957 w2982 w3007 w3032 w3057 w3082 w3107 w3132 w3157 w3185 w3210 w3235 w3260 w3285 w3310 w3335 w3360 w3385 w3410 w3435 w3460 w3485 w3510 w3535 w3560 w3585 w3610 w3635 w3660 w3685 w3710 w3735 w3760 w3785 w3810 w3835 w3860 w3885 w3910 w3935 w3960 w3985 w4010 w4035 w4060 w4085 w4110 w4135 w4160 w4185 w4210 w4235 w4261 w4286 w4311]
      tunnel: w18 -> [w30 w55 w80 w105 w130 w155 w180 w205 w230 w255 w280 w305 w330 w355 w380 w405 w430 w455 w480 w505 w530 w555 w580 w605 w630 w655 w680 w705 w730 w755 w780 w805 w830 w855 w880 w905 w930 w955 w980 w1005 w1030 w1055 w1080 w1105 w1130 w1155 w1180 w1205 w1230 w1255 w1280 w1305 w1330 w1355 w1380 w1405 w1430 w1455 w1481 w1512 w1542 w1567 w1592 w1617 w1642 w1667 w1692 w1717 w1742 w1767 w1792 w1817 w1842 w1867 w1892 w1917 w1942 w1967 w1992 w2017 w2042 w2067 w2092 w2119 w2144 w2169 w2233 w2258 w2283 w2308 w2333 w2358 w2383 w2408 w2433 w2458 w2483 w2508 w2533 w2558 w2583 w2608 w2633 w2658 w2683 w2708 w2733 w2758 w2783 w2808 w2833 w2858 w2883 w2908 w2933 w2958 w2983 w3008 w3033 w3058 w3083 w3108 w3133 w3158 w3186 w3211 w3236 w3261 w3286 w3311 w3336 w3361 w3386 w3411 w3436 w3461 w3486 w3511 w3536 w3561 w3586 w3611 w3636 w3661 w3686 w3711 w3736 w3761 w3786 w3811 w3836 w3861 w3886 w3911 w3936 w3961 w3986 w4011 w4036 w4061 w4086 w4111 w4136 w4161 w4186 w4211 w4236 w4262 w4287 w4312]
      tunnel: w17 -> [w23 w48 w72 w98 w123 w148 w173 w198 w223 w248 w273 w298 w323 w348 w373 w398 w423 w448 w473 w498 w523 w548 w573 w598 w623 w648 w673 w698 w723 w748 w773 w798 w823 w848 w873 w898 w923 w948 w973 w998 w1023 w1048 w1073 w1098 w1123 w1148 w1173 w1198 w1223 w1248 w1273 w1298 w1323 w1348 w1373 w1398 w1423 w1448 w1474 w1505 w1535 w1560 w1585 w1610 w1635 w1660 w1685 w1710 w1735 w1760 w1785 w1810 w1835 w1860 w1885 w1910 w1935 w1960 w1985 w2010 w2035 w2060 w2085 w2112 w2137 w2162 w2226 w2251 w2276 w2301 w2326 w2351 w2376 w2401 w2426 w2451 w2476 w2501 w2526 w2551 w2576 w2601 w2626 w2651 w2676 w2701 w2726 w2751 w2776 w2801 w2826 w2851 w2876 w2901 w2926 w2951 w2976 w3001 w3026 w3051 w3076 w3101 w3126 w3151 w3180 w3205 w3230 w3255 w3280 w3305 w3330 w3355 w3380 w3405 w3430 w3455 w3479 w3504 w3529 w3554 w3579 w3604 w3629 w3654 w3679 w3704 w3729 w3754 w3779 w3804 w3829 w3854 w3879 w3904 w3929 w3954 w3979 w4004 w4029 w4054 w4079 w4104 w4129 w4154 w4179 w4204 w4229 w4255 w4280 w4305]
      tunnel: w15 -> [w26 w51 w76 w101 w126 w151 w176 w201 w226 w251 w276 w301 w326 w351 w376 w401 w426 w451 w476 w501 w526 w551 w576 w601 w626 w651 w676 w701 w726 w751 w776 w801 w826 w851 w876 w901 w926 w951 w976 w1001 w1026 w1051 w1076 w1101 w1126 w1151 w1176 w1201 w1226 w1251 w1276 w1301 w1326 w1351 w1376 w1401 w1426 w1451 w1477 w1508 w1538 w1563 w1588 w1613 w1638 w1663 w1688 w1713 w1738 w1763 w1788 w1813 w1838 w1863 w1888 w1913 w1938 w1963 w1988 w2013 w2038 w2063 w2088 w2115 w2140 w2165 w2229 w2254 w2279 w2304 w2329 w2354 w2379 w2404 w2429 w2454 w2479 w2504 w2529 w2554 w2579 w2604 w2629 w2654 w2679 w2704 w2729 w2754 w2779 w2804 w2829 w2854 w2879 w2904 w2929 w2954 w2979 w3004 w3029 w3054 w3079 w3104 w3129 w3154 w3177 w3204 w3229 w3254 w3279 w3304 w3329 w3354 w3379 w3404 w3429 w3454 w3482 w3507 w3532 w3557 w3582 w3607 w3632 w3657 w3682 w3707 w3732 w3757 w3782 w3807 w3832 w3857 w3882 w3907 w3932 w3957 w3982 w4007 w4032 w4057 w4082 w4107 w4132 w4157 w4182 w4207 w4232 w4258 w4283 w4308]
      tunnel: w14 -> [w28 w53 w78 w103 w128 w153 w178 w203 w228 w253 w278 w303 w328 w353 w378 w403 w428 w453 w478 w503 w528 w553 w578 w603 w628 w653 w678 w703 w728 w753 w778 w803 w828 w853 w878 w903 w928 w953 w978 w1003 w1028 w1053 w1078 w1103 w1128 w1153 w1178 w1203 w1228 w1253 w1278 w1303 w1328 w1353 w1378 w1403 w1428 w1453 w1479 w1510 w1540 w1565 w1590 w1615 w1640 w1665 w1690 w1715 w1740 w1765 w1790 w1815 w1840 w1865 w1890 w1915 w1940 w1965 w1990 w2015 w2040 w2065 w2090 w2117 w2142 w2167 w2231 w2256 w2281 w2306 w2331 w2356 w2381 w2406 w2431 w2456 w2481 w2506 w2531 w2556 w2581 w2606 w2631 w2656 w2681 w2706 w2731 w2756 w2781 w2806 w2831 w2856 w2881 w2906 w2931 w2956 w2981 w3006 w3031 w3056 w3081 w3106 w3131 w3156 w3184 w3209 w3234 w3259 w3284 w3309 w3334 w3359 w3384 w3409 w3434 w3459 w3484 w3509 w3534 w3559 w3584 w3609 w3634 w3659 w3684 w3709 w3734 w3759 w3784 w3809 w3834 w3859 w3884 w3909 w3934 w3959 w3984 w4009 w4034 w4059 w4084 w4109 w4134 w4159 w4184 w4209 w4234 w4260 w4285 w4310]
      tunnel: [w27 w52 w77 w102 w127 w152 w177 w202 w227 w252 w277 w302 w327 w352 w377 w402 w427 w452 w477 w502 w527 w552 w577 w602 w627 w652 w677 w702 w727 w752 w777 w802 w827 w852 w877 w902 w927 w952 w977 w1002 w1027 w1052 w1077 w1102 w1127 w1152 w1177 w1202 w1227 w1252 w1277 w1302 w1327 w1352 w1377 w1402 w1427 w1452 w1478 w1509 w1539 w1564 w1589 w1614 w1639 w1664 w1689 w1714 w1739 w1764 w1789 w1814 w1839 w1864 w1889 w1914 w1939 w1964 w1989 w2014 w2039 w2064 w2089 w2116 w2141 w2166 w2230 w2255 w2280 w2305 w2330 w2355 w2380 w2405 w2430 w2455 w2480 w2505 w2530 w2555 w2580 w2605 w2630 w2655 w2680 w2705 w2730 w2755 w2780 w2805 w2830 w2855 w2880 w2905 w2930 w2955 w2980 w3005 w3030 w3055 w3080 w3105 w3130 w3155 w3183 w3208 w3233 w3258 w3283 w3308 w3333 w3358 w3383 w3408 w3433 w3458 w3483 w3508 w3533 w3558 w3583 w3608 w3633 w3658 w3683 w3708 w3733 w3758 w3783 w3808 w3833 w3858 w3883 w3908 w3933 w3958 w3983 w4008 w4033 w4058 w4083 w4108 w4133 w4158 w4183 w4208 w4233 w4259 w4284 w4309] -> w13
      tunnel: [w25 w50 w75 w100 w125 w150 w175 w200 w225 w250 w275 w300 w325 w350 w375 w400 w425 w450 w475 w500 w525 w550 w575 w600 w625 w650 w675 w700 w725 w750 w775 w800 w825 w850 w875 w900 w925 w950 w975 w1000 w1025 w1050 w1075 w1100 w1125 w1150 w1175 w1200 w1225 w1250 w1275 w1300 w1325 w1350 w1375 w1400 w1425 w1450 w1476 w1507 w1537 w1562 w1587 w1612 w1637 w1662 w1687 w1712 w1737 w1762 w1787 w1812 w1837 w1862 w1887 w1912 w1937 w1962 w1987 w2012 w2037 w2062 w2087 w2114 w2139 w2164 w2228 w2253 w2278 w2303 w2328 w2353 w2378 w2403 w2428 w2453 w2478 w2503 w2528 w2553 w2578 w2603 w2628 w2653 w2678 w2703 w2728 w2753 w2778 w2803 w2828 w2853 w2878 w2903 w2928 w2953 w2978 w3003 w3028 w3053 w3078 w3103 w3128 w3153 w3182 w3207 w3232 w3257 w3282 w3307 w3332 w3357 w3382 w3407 w3432 w3457 w3481 w3506 w3531 w3556 w3581 w3606 w3631 w3656 w3681 w3706 w3731 w3756 w3781 w3806 w3831 w3856 w3881 w3906 w3931 w3956 w3981 w4006 w4031 w4056 w4081 w4106 w4131 w4156 w4181 w4206 w4231 w4257 w4282 w4307] -> w12
      tunnel: [w24 w49 w73 w99 w124 w149 w174 w199 w224 w249 w274 w299 w324 w349 w374 w399 w424 w449 w474 w499 w524 w549 w574 w599 w624 w649 w674 w699 w724 w749 w774 w799 w824 w849 w874 w899 w924 w949 w974 w999 w1024 w1049 w1074 w1099 w1124 w1149 w1174 w1199 w1224 w1249 w1274 w1299 w1324 w1349 w1374 w1399 w1424 w1449 w1475 w1506 w1536 w1561 w1586 w1611 w1636 w1661 w1686 w1711 w1736 w1761 w1786 w1811 w1836 w1861 w1886 w1911 w1936 w1961 w1986 w2011 w2036 w2061 w2086 w2113 w2138 w2163 w2227 w2252 w2277 w2302 w2327 w2352 w2377 w2402 w2427 w2452 w2477 w2502 w2527 w2552 w2577 w2602 w2627 w2652 w2677 w2702 w2727 w2752 w2777 w2802 w2827 w2852 w2877 w2902 w2927 w2952 w2977 w3002 w3027 w3052 w3077 w3102 w3127 w3152 w3181 w3206 w3231 w3256 w3281 w3306 w3331 w3356 w3381 w3406 w3431 w3456 w3480 w3505 w3530 w3555 w3580 w3605 w3630 w3655 w3680 w3705 w3730 w3755 w3780 w3805 w3830 w3855 w3880 w3905 w3930 w3955 w3980 w4005 w4030 w4055 w4080 w4105 w4130 w4155 w4180 w4205 w4230 w4256 w4281 w4306] -> w11
      tunnel: w10 -> [_ _ _ _ _ _ _ _ _ _ _ _ _ _ _ _ _ _ _ _ _ _ _ _ _ _ _ _ _ _ _ _ _ _ _ _ _ _ _ _ _ _ _ _ _ _ _ _ _ _ _ _ _ _ _ _ _ _ w1472 _ _ _ _ _ _ _ _ _ _ _ _ _ _ _ _ _ _ _ _ _ _ _ _ _ _ _ _ _ _ _ _ _ _ _ _ _ _ _ _ _ _ _ _ _ _ _ _ _ _ _ _ _ _ _ _ _ _ _ _ _ _ _ _ _ _ _ _ _ _ _ _ _ _ _ _ _ _ _ _ _ _ _ _ _ _ _ _ _ _ _ _ _ _ _ _ _ _ _ _ _ _ _ _ _ _ _ _ _ _ _]
      tunnel: w9 -> [_ _ _ _ _ _ _ _ _ _ _ _ _ _ _ _ _ _ _ _ _ _ _ _ _ _ _ _ _ _ _ _ _ _ _ _ _ _ _ _ _ _ _ _ _ _ _ _ _ _ _ _ _ _ _ _ _ _ _ w1503 _ _ _ _ _ _ _ _ _ _ _ _ _ _ _ _ _ _ _ _ _ _ _ _ _ _ _ _ _ _ _ _ _ _ _ _ _ _ _ _ _ _ _ _ _ _ _ _ _ _ _ _ _ _ _ _ _ _ _ _ _ _ _ _ _ _ _ _ _ _ _ _ _ _ _ _ _ _ _ _ _ _ _ _ _ _ _ _ _ _ _ _ _ _ _ _ _ _ _ _ _ _ _ _ _ _ _ _ _ _]
      frame "GUI:Visible Settings Tab" {
        n4 = case shown="True" w30 {
          tunnel: w29 -> [w38 w42]
          tunnel: w28 -> [w37 w45]
          tunnel: [w36 w44] -> w27
          tunnel: w26 -> [w35 w43]
          tunnel: [w34 w40] -> w25
          tunnel: "Visible Settings Tab" -> [w33 w46]
          tunnel: [w31 w39] -> w24
          tunnel: w23 -> [_ w39]
          frame False {
            n5 = Get Variant Attribute(Variant=w37, name=w38, default value (empty Variant)=w33, error in=w35) -> (duplicate Variant=w36:variant, value=w32:string, error out=w34:errorcluster)  [unwired: 1 out]
            n6 = To Variant(anything=w32) -> (Variant=w31:variant)
          }
          frame True {
            n7 = Variant To Data(type=w46, Variant=w39) -> (data=w41:string)  [unwired: 1 in, 1 out]
            n8 = Set Variant Attribute(Variant=w45, name=w42, value=w41, error in=w43) -> (Variant out=w44:variant, error out=w40:errorcluster)  [unwired: 1 out]
          }
        }
      }
      frame "GUI:Last Run Version" {
        n9 = case shown="True" w55 {
          tunnel: w54 -> [w63 w67]
          tunnel: w53 -> [w62 w70]
          tunnel: [w61 w69] -> w52
          tunnel: w51 -> [w60 w68]
          tunnel: [w59 w65] -> w50
          tunnel: "Last Run Version" -> [w58 w71]
          tunnel: [w56 w64] -> w49
          tunnel: w48 -> [_ w64]
          frame False {
            n10 = Get Variant Attribute(Variant=w62, name=w63, default value (empty Variant)=w58, error in=w60) -> (duplicate Variant=w61:variant, value=w57:string, error out=w59:errorcluster)  [unwired: 1 out]
            n11 = To Variant(anything=w57) -> (Variant=w56:variant)
          }
          frame True {
            n12 = Variant To Data(type=w71, Variant=w64) -> (data=w66:string)  [unwired: 1 in, 1 out]
            n13 = Set Variant Attribute(Variant=w70, name=w67, value=w66, error in=w68) -> (Variant out=w69:variant, error out=w65:errorcluster)  [unwired: 1 out]
          }
        }
      }
      frame "Source Image:Use Image Histogram for Contrast", Default {
        n14 = case shown="True" w80 {
          tunnel: w79 -> [w88 w92]
          tunnel: w78 -> [w87 w95]
          tunnel: [w86 w94] -> w77
          tunnel: w76 -> [w85 w93]
          tunnel: [w84 w90] -> w75
          tunnel: "Use Image Histogram for Contrast" -> [w83 w96]
          tunnel: [w81 w89] -> w73
          tunnel: w72 -> [_ w89]
          frame False {
            n15 = Get Variant Attribute(Variant=w87, name=w88, default value (empty Variant)=w83, error in=w85) -> (duplicate Variant=w86:variant, value=w82:bool, error out=w84:errorcluster)  [unwired: 1 out]
            n16 = To Variant(anything=w82) -> (Variant=w81:variant)
          }
          frame True {
            n17 = Variant To Data(type=w96, Variant=w89) -> (data=w91:bool)  [unwired: 1 in, 1 out]
            n18 = Set Variant Attribute(Variant=w95, name=w92, value=w91, error in=w93) -> (Variant out=w94:variant, error out=w90:errorcluster)  [unwired: 1 out]
          }
        }
      }
      frame "Source Image:Low Count Pixels Rejection Options" {
        n19 = case shown="True" w105 {
          tunnel: w104 -> [w113 w117]
          tunnel: w103 -> [w112 w120]
          tunnel: [w111 w119] -> w102
          tunnel: w101 -> [w110 w118]
          tunnel: [w109 w115] -> w100
          tunnel: "Low Count Pixels Rejection Options" -> [w108 w121]
          tunnel: [w106 w114] -> w99
          tunnel: w98 -> [_ w114]
          frame False {
            n20 = Get Variant Attribute(Variant=w112, name=w113, default value (empty Variant)=w108, error in=w110) -> (duplicate Variant=w111:variant, value=w107:T4, error out=w109:errorcluster)  [unwired: 1 out]
            n21 = To Variant(anything=w107) -> (Variant=w106:variant)
          }
          frame True {
            n22 = Variant To Data(type=w121, Variant=w114) -> (data=w116:T4)  [unwired: 1 in, 1 out]
            n23 = Set Variant Attribute(Variant=w120, name=w117, value=w116, error in=w118) -> (Variant out=w119:variant, error out=w115:errorcluster)  [unwired: 1 out]
          }
        }
      }
      frame "Source Image:High Count Pixels Rejection Options" {
        n24 = case shown="True" w130 {
          tunnel: w129 -> [w138 w142]
          tunnel: w128 -> [w137 w145]
          tunnel: [w136 w144] -> w127
          tunnel: w126 -> [w135 w143]
          tunnel: [w134 w140] -> w125
          tunnel: "High Count Pixels Rejection Options" -> [w133 w146]
          tunnel: [w131 w139] -> w124
          tunnel: w123 -> [_ w139]
          frame False {
            n25 = Get Variant Attribute(Variant=w137, name=w138, default value (empty Variant)=w133, error in=w135) -> (duplicate Variant=w136:variant, value=w132:T5, error out=w134:errorcluster)  [unwired: 1 out]
            n26 = To Variant(anything=w132) -> (Variant=w131:variant)
          }
          frame True {
            n27 = Variant To Data(type=w146, Variant=w139) -> (data=w141:T5)  [unwired: 1 in, 1 out]
            n28 = Set Variant Attribute(Variant=w145, name=w142, value=w141, error in=w143) -> (Variant out=w144:variant, error out=w140:errorcluster)  [unwired: 1 out]
          }
        }
      }
      frame "Source Image:Use Image Brightness" {
        n29 = case shown="True" w155 {
          tunnel: w154 -> [w163 w167]
          tunnel: w153 -> [w162 w170]
          tunnel: [w161 w169] -> w152
          tunnel: w151 -> [w160 w168]
          tunnel: [w159 w165] -> w150
          tunnel: "Use Image Brightness" -> [w158 w171]
          tunnel: [w156 w164] -> w149
          tunnel: w148 -> [_ w164]
          frame False {
            n30 = Get Variant Attribute(Variant=w162, name=w163, default value (empty Variant)=w158, error in=w160) -> (duplicate Variant=w161:variant, value=w157:bool, error out=w159:errorcluster)  [unwired: 1 out]
            n31 = To Variant(anything=w157) -> (Variant=w156:variant)
          }
          frame True {
            n32 = Variant To Data(type=w171, Variant=w164) -> (data=w166:bool)  [unwired: 1 in, 1 out]
            n33 = Set Variant Attribute(Variant=w170, name=w167, value=w166, error in=w168) -> (Variant out=w169:variant, error out=w165:errorcluster)  [unwired: 1 out]
          }
        }
      }
      frame "Source Image:Blend Overlay with Image Background" {
        n34 = case shown="True" w180 {
          tunnel: w179 -> [w188 w192]
          tunnel: w178 -> [w187 w195]
          tunnel: [w186 w194] -> w177
          tunnel: w176 -> [w185 w193]
          tunnel: [w184 w190] -> w175
          tunnel: "Blend Overlay with Image Background" -> [w183 w196]
          tunnel: [w181 w189] -> w174
          tunnel: w173 -> [_ w189]
          frame False {
            n35 = Get Variant Attribute(Variant=w187, name=w188, default value (empty Variant)=w183, error in=w185) -> (duplicate Variant=w186:variant, value=w182:bool, error out=w184:errorcluster)  [unwired: 1 out]
            n36 = To Variant(anything=w182) -> (Variant=w181:variant)
          }
          frame True {
            n37 = Variant To Data(type=w196, Variant=w189) -> (data=w191:bool)  [unwired: 1 in, 1 out]
            n38 = Set Variant Attribute(Variant=w195, name=w192, value=w191, error in=w193) -> (Variant out=w194:variant, error out=w190:errorcluster)  [unwired: 1 out]
          }
        }
      }
      frame "Source Image:Use Fixed ROI Diameter" {
        n39 = case shown="True" w205 {
          tunnel: w204 -> [w213 w217]
          tunnel: w203 -> [w212 w220]
          tunnel: [w211 w219] -> w202
          tunnel: w201 -> [w210 w218]
          tunnel: [w209 w215] -> w200
          tunnel: "Use Fixed ROI Diameter" -> [w208 w221]
          tunnel: [w206 w214] -> w199
          tunnel: w198 -> [_ w214]
          frame False {
            n40 = Get Variant Attribute(Variant=w212, name=w213, default value (empty Variant)=w208, error in=w210) -> (duplicate Variant=w211:variant, value=w207:bool, error out=w209:errorcluster)  [unwired: 1 out]
            n41 = To Variant(anything=w207) -> (Variant=w206:variant)
          }
          frame True {
            n42 = Variant To Data(type=w221, Variant=w214) -> (data=w216:bool)  [unwired: 1 in, 1 out]
            n43 = Set Variant Attribute(Variant=w220, name=w217, value=w216, error in=w218) -> (Variant out=w219:variant, error out=w215:errorcluster)  [unwired: 1 out]
          }
        }
      }
      frame "Source Image:ROI Diameter" {
        n44 = case shown="True" w230 {
          tunnel: w229 -> [w238 w242]
          tunnel: w228 -> [w237 w245]
          tunnel: [w236 w244] -> w227
          tunnel: w226 -> [w235 w243]
          tunnel: [w234 w240] -> w225
          tunnel: "ROI Diameter" -> [w233 w246]
          tunnel: [w231 w239] -> w224
          tunnel: w223 -> [_ w239]
          frame False {
            n45 = Get Variant Attribute(Variant=w237, name=w238, default value (empty Variant)=w233, error in=w235) -> (duplicate Variant=w236:variant, value=w232:i32, error out=w234:errorcluster)  [unwired: 1 out]
            n46 = To Variant(anything=w232) -> (Variant=w231:variant)
          }
          frame True {
            n47 = Variant To Data(type=w246, Variant=w239) -> (data=w241:i32)  [unwired: 1 in, 1 out]
            n48 = Set Variant Attribute(Variant=w245, name=w242, value=w241, error in=w243) -> (Variant out=w244:variant, error out=w240:errorcluster)  [unwired: 1 out]
          }
        }
      }
      frame "Source Image:ROI Center Color" {
        n49 = case shown="True" w255 {
          tunnel: w254 -> [w263 w267]
          tunnel: w253 -> [w262 w270]
          tunnel: [w261 w269] -> w252
          tunnel: w251 -> [w260 w268]
          tunnel: [w259 w265] -> w250
          tunnel: "ROI Center Color" -> [w258 w271]
          tunnel: [w256 w264] -> w249
          tunnel: w248 -> [_ w264]
          frame False {
            n50 = Get Variant Attribute(Variant=w262, name=w263, default value (empty Variant)=w258, error in=w260) -> (duplicate Variant=w261:variant, value=w257:u32, error out=w259:errorcluster)  [unwired: 1 out]
            n51 = To Variant(anything=w257) -> (Variant=w256:variant)
          }
          frame True {
            n52 = Variant To Data(type=w271, Variant=w264) -> (data=w266:u32)  [unwired: 1 in, 1 out]
            n53 = Set Variant Attribute(Variant=w270, name=w267, value=w266, error in=w268) -> (Variant out=w269:variant, error out=w265:errorcluster)  [unwired: 1 out]
          }
        }
      }
      frame "Source Image:Peak Threshold" {
        n54 = case shown="True" w280 {
          tunnel: w279 -> [w288 w292]
          tunnel: w278 -> [w287 w295]
          tunnel: [w286 w294] -> w277
          tunnel: w276 -> [w285 w293]
          tunnel: [w284 w290] -> w275
          tunnel: "Peak Threshold" -> [w283 w296]
          tunnel: [w281 w289] -> w274
          tunnel: w273 -> [_ w289]
          frame False {
            n55 = Get Variant Attribute(Variant=w287, name=w288, default value (empty Variant)=w283, error in=w285) -> (duplicate Variant=w286:variant, value=w282:dbl, error out=w284:errorcluster)  [unwired: 1 out]
            n56 = To Variant(anything=w282) -> (Variant=w281:variant)
          }
          frame True {
            n57 = Variant To Data(type=w296, Variant=w289) -> (data=w291:dbl)  [unwired: 1 in, 1 out]
            n58 = Set Variant Attribute(Variant=w295, name=w292, value=w291, error in=w293) -> (Variant out=w294:variant, error out=w290:errorcluster)  [unwired: 1 out]
          }
        }
      }
      frame "Source Image:Intensity Threshold" {
        n59 = case shown="True" w305 {
          tunnel: w304 -> [w313 w317]
          tunnel: w303 -> [w312 w320]
          tunnel: [w311 w319] -> w302
          tunnel: w301 -> [w310 w318]
          tunnel: [w309 w315] -> w300
          tunnel: "Intensity Threshold" -> [w308 w321]
          tunnel: [w306 w314] -> w299
          tunnel: w298 -> [_ w314]
          frame False {
            n60 = Get Variant Attribute(Variant=w312, name=w313, default value (empty Variant)=w308, error in=w310) -> (duplicate Variant=w311:variant, value=w307:dbl, error out=w309:errorcluster)  [unwired: 1 out]
            n61 = To Variant(anything=w307) -> (Variant=w306:variant)
          }
          frame True {
            n62 = Variant To Data(type=w321, Variant=w314) -> (data=w316:dbl)  [unwired: 1 in, 1 out]
            n63 = Set Variant Attribute(Variant=w320, name=w317, value=w316, error in=w318) -> (Variant out=w319:variant, error out=w315:errorcluster)  [unwired: 1 out]
          }
        }
      }
      frame "Source Image:Image Binning Options" {
        n64 = case shown="True" w330 {
          tunnel: w329 -> [w338 w342]
          tunnel: w328 -> [w337 w345]
          tunnel: [w336 w344] -> w327
          tunnel: w326 -> [w335 w343]
          tunnel: [w334 w340] -> w325
          tunnel: "Image Binning Options" -> [w333 w346]
          tunnel: [w331 w339] -> w324
          tunnel: w323 -> [_ w339]
          frame False {
            n65 = Get Variant Attribute(Variant=w337, name=w338, default value (empty Variant)=w333, error in=w335) -> (duplicate Variant=w336:variant, value=w332:T7, error out=w334:errorcluster)  [unwired: 1 out]
            n66 = To Variant(anything=w332) -> (Variant=w331:variant)
          }
          frame True {
            n67 = Variant To Data(type=w346, Variant=w339) -> (data=w341:T7)  [unwired: 1 in, 1 out]
            n68 = Set Variant Attribute(Variant=w345, name=w342, value=w341, error in=w343) -> (Variant out=w344:variant, error out=w340:errorcluster)  [unwired: 1 out]
          }
        }
      }
      frame "Source Image:Image Smoothing Options" {
        n69 = case shown="True" w355 {
          tunnel: w354 -> [w363 w367]
          tunnel: w353 -> [w362 w370]
          tunnel: [w361 w369] -> w352
          tunnel: w351 -> [w360 w368]
          tunnel: [w359 w365] -> w350
          tunnel: "Image Smoothing Options" -> [w358 w371]
          tunnel: [w356 w364] -> w349
          tunnel: w348 -> [_ w364]
          frame False {
            n70 = Get Variant Attribute(Variant=w362, name=w363, default value (empty Variant)=w358, error in=w360) -> (duplicate Variant=w361:variant, value=w357:T9, error out=w359:errorcluster)  [unwired: 1 out]
            n71 = To Variant(anything=w357) -> (Variant=w356:variant)
          }
          frame True {
            n72 = Variant To Data(type=w371, Variant=w364) -> (data=w366:T9)  [unwired: 1 in, 1 out]
            n73 = Set Variant Attribute(Variant=w370, name=w367, value=w366, error in=w368) -> (Variant out=w369:variant, error out=w365:errorcluster)  [unwired: 1 out]
          }
        }
      }
      frame "Source Image:Image Histogram Active" {
        w372 = FALSE  # Not a Settings Window Control
        n74 = case shown="True" w380 {
          tunnel: w379 -> [w388 w392]
          tunnel: w378 -> [w387 w395]
          tunnel: [w386 w394] -> w377
          tunnel: w376 -> [w385 w393]
          tunnel: [w384 w390] -> w375
          tunnel: w372 -> [w383 w396]
          tunnel: [w381 w389] -> w374
          tunnel: w373 -> [_ w389]
          frame False {
            n75 = Get Variant Attribute(Variant=w387, name=w388, default value (empty Variant)=w383, error in=w385) -> (duplicate Variant=w386:variant, value=w382:bool, error out=w384:errorcluster)  [unwired: 1 out]
            n76 = To Variant(anything=w382) -> (Variant=w381:variant)
          }
          frame True {
            n77 = Variant To Data(type=w396, Variant=w389) -> (data=w391:bool)  [unwired: 1 in, 1 out]
            n78 = Set Variant Attribute(Variant=w395, name=w392, value=w391, error in=w393) -> (Variant out=w394:variant, error out=w390:errorcluster)  [unwired: 1 out]
          }
        }
      }
      frame "Source Image:Invert Binary Mask" {
        n79 = case shown="True" w405 {
          tunnel: w404 -> [w413 w417]
          tunnel: w403 -> [w412 w420]
          tunnel: [w411 w419] -> w402
          tunnel: w401 -> [w410 w418]
          tunnel: [w409 w415] -> w400
          tunnel: "Invert Binary Mask" -> [w408 w421]
          tunnel: [w406 w414] -> w399
          tunnel: w398 -> [_ w414]
          frame False {
            n80 = Get Variant Attribute(Variant=w412, name=w413, default value (empty Variant)=w408, error in=w410) -> (duplicate Variant=w411:variant, value=w407:bool, error out=w409:errorcluster)  [unwired: 1 out]
            n81 = To Variant(anything=w407) -> (Variant=w406:variant)
          }
          frame True {
            n82 = Variant To Data(type=w421, Variant=w414) -> (data=w416:bool)  [unwired: 1 in, 1 out]
            n83 = Set Variant Attribute(Variant=w420, name=w417, value=w416, error in=w418) -> (Variant out=w419:variant, error out=w415:errorcluster)  [unwired: 1 out]
          }
        }
      }
      frame "Source Image:Hot Pixel Removal" {
        n84 = case shown="True" w430 {
          tunnel: w429 -> [w438 w442]
          tunnel: w428 -> [w437 w445]
          tunnel: [w436 w444] -> w427
          tunnel: w426 -> [w435 w443]
          tunnel: [w434 w440] -> w425
          tunnel: "Hot Pixel Removal" -> [w433 w446]
          tunnel: [w431 w439] -> w424
          tunnel: w423 -> [_ w439]
          frame False {
            n85 = Get Variant Attribute(Variant=w437, name=w438, default value (empty Variant)=w433, error in=w435) -> (duplicate Variant=w436:variant, value=w432:T6, error out=w434:errorcluster)  [unwired: 1 out]
            n86 = To Variant(anything=w432) -> (Variant=w431:variant)
          }
          frame True {
            n87 = Variant To Data(type=w446, Variant=w439) -> (data=w441:T6)  [unwired: 1 in, 1 out]
            n88 = Set Variant Attribute(Variant=w445, name=w442, value=w441, error in=w443) -> (Variant out=w444:variant, error out=w440:errorcluster)  [unwired: 1 out]
          }
        }
      }
      frame "Source Image:Overlay Analyzed ROI Center" {
        n89 = case shown="True" w455 {
          tunnel: w454 -> [w463 w467]
          tunnel: w453 -> [w462 w470]
          tunnel: [w461 w469] -> w452
          tunnel: w451 -> [w460 w468]
          tunnel: [w459 w465] -> w450
          tunnel: "Overlay Analyzed ROI Center" -> [w458 w471]
          tunnel: [w456 w464] -> w449
          tunnel: w448 -> [_ w464]
          frame False {
            n90 = Get Variant Attribute(Variant=w462, name=w463, default value (empty Variant)=w458, error in=w460) -> (duplicate Variant=w461:variant, value=w457:bool, error out=w459:errorcluster)  [unwired: 1 out]
            n91 = To Variant(anything=w457) -> (Variant=w456:variant)
          }
          frame True {
            n92 = Variant To Data(type=w471, Variant=w464) -> (data=w466:bool)  [unwired: 1 in, 1 out]
            n93 = Set Variant Attribute(Variant=w470, name=w467, value=w466, error in=w468) -> (Variant out=w469:variant, error out=w465:errorcluster)  [unwired: 1 out]
          }
        }
      }
      frame "Source Image:Auto-Adjust Contrast" {
        w472 = FALSE  # Not a Settings Window Control
        n94 = case shown="True" w480 {
          tunnel: w479 -> [w488 w492]
          tunnel: w478 -> [w487 w495]
          tunnel: [w486 w494] -> w477
          tunnel: w476 -> [w485 w493]
          tunnel: [w484 w490] -> w475
          tunnel: w472 -> [w483 w496]
          tunnel: [w481 w489] -> w474
          tunnel: w473 -> [_ w489]
          frame False {
            n95 = Get Variant Attribute(Variant=w487, name=w488, default value (empty Variant)=w483, error in=w485) -> (duplicate Variant=w486:variant, value=w482:bool, error out=w484:errorcluster)  [unwired: 1 out]
            n96 = To Variant(anything=w482) -> (Variant=w481:variant)
          }
          frame True {
            n97 = Variant To Data(type=w496, Variant=w489) -> (data=w491:bool)  [unwired: 1 in, 1 out]
            n98 = Set Variant Attribute(Variant=w495, name=w492, value=w491, error in=w493) -> (Variant out=w494:variant, error out=w490:errorcluster)  [unwired: 1 out]
          }
        }
      }
      frame "Source Image:Histogram Lower Percentile" {
        w497 = 1.0  # Not a Settings Window Control
        n99 = case shown="True" w505 {
          tunnel: w504 -> [w513 w517]
          tunnel: w503 -> [w512 w520]
          tunnel: [w511 w519] -> w502
          tunnel: w501 -> [w510 w518]
          tunnel: [w509 w515] -> w500
          tunnel: w497 -> [w508 w521]
          tunnel: [w506 w514] -> w499
          tunnel: w498 -> [_ w514]
          frame False {
            n100 = Get Variant Attribute(Variant=w512, name=w513, default value (empty Variant)=w508, error in=w510) -> (duplicate Variant=w511:variant, value=w507:dbl, error out=w509:errorcluster)  [unwired: 1 out]
            n101 = To Variant(anything=w507) -> (Variant=w506:variant)
          }
          frame True {
            n102 = Variant To Data(type=w521, Variant=w514) -> (data=w516:dbl)  [unwired: 1 in, 1 out]
            n103 = Set Variant Attribute(Variant=w520, name=w517, value=w516, error in=w518) -> (Variant out=w519:variant, error out=w515:errorcluster)  [unwired: 1 out]
          }
        }
      }
      frame "Source Image:Histogram Upper Percentile" {
        w522 = 1.0  # Not a Settings Window Control
        n104 = case shown="True" w530 {
          tunnel: w529 -> [w538 w542]
          tunnel: w528 -> [w537 w545]
          tunnel: [w536 w544] -> w527
          tunnel: w526 -> [w535 w543]
          tunnel: [w534 w540] -> w525
          tunnel: w522 -> [w533 w546]
          tunnel: [w531 w539] -> w524
          tunnel: w523 -> [_ w539]
          frame False {
            n105 = Get Variant Attribute(Variant=w537, name=w538, default value (empty Variant)=w533, error in=w535) -> (duplicate Variant=w536:variant, value=w532:dbl, error out=w534:errorcluster)  [unwired: 1 out]
            n106 = To Variant(anything=w532) -> (Variant=w531:variant)
          }
          frame True {
            n107 = Variant To Data(type=w546, Variant=w539) -> (data=w541:dbl)  [unwired: 1 in, 1 out]
            n108 = Set Variant Attribute(Variant=w545, name=w542, value=w541, error in=w543) -> (Variant out=w544:variant, error out=w540:errorcluster)  [unwired: 1 out]
          }
        }
      }
      frame "Source Image:Save Source Image" {
        w547 = FALSE  # Save Source Image
        n109 = case shown="True" w555 {
          tunnel: w554 -> [w563 w567]
          tunnel: w553 -> [w562 w570]
          tunnel: [w561 w569] -> w552
          tunnel: w551 -> [w560 w568]
          tunnel: [w559 w565] -> w550
          tunnel: w547 -> [w558 w571]
          tunnel: [w556 w564] -> w549
          tunnel: w548 -> [_ w564]
          frame False {
            n110 = Get Variant Attribute(Variant=w562, name=w563, default value (empty Variant)=w558, error in=w560) -> (duplicate Variant=w561:variant, value=w557:bool, error out=w559:errorcluster)  [unwired: 1 out]
            n111 = To Variant(anything=w557) -> (Variant=w556:variant)
          }
          frame True {
            n112 = Variant To Data(type=w571, Variant=w564) -> (data=w566:bool)  [unwired: 1 in, 1 out]
            n113 = Set Variant Attribute(Variant=w570, name=w567, value=w566, error in=w568) -> (Variant out=w569:variant, error out=w565:errorcluster)  [unwired: 1 out]
          }
        }
      }
      frame "Source Image:Scale Bar Options" {
        n114 = case shown="True" w580 {
          tunnel: w579 -> [w588 w592]
          tunnel: w578 -> [w587 w595]
          tunnel: [w586 w594] -> w577
          tunnel: w576 -> [w585 w593]
          tunnel: [w584 w590] -> w575
          tunnel: "Scale Bar Options" -> [w583 w596]
          tunnel: [w581 w589] -> w574
          tunnel: w573 -> [_ w589]
          frame False {
            n115 = Get Variant Attribute(Variant=w587, name=w588, default value (empty Variant)=w583, error in=w585) -> (duplicate Variant=w586:variant, value=w582:T12, error out=w584:errorcluster)  [unwired: 1 out]
            n116 = To Variant(anything=w582) -> (Variant=w581:variant)
          }
          frame True {
            n117 = Variant To Data(type=w596, Variant=w589) -> (data=w591:T12)  [unwired: 1 in, 1 out]
            n118 = Set Variant Attribute(Variant=w595, name=w592, value=w591, error in=w593) -> (Variant out=w594:variant, error out=w590:errorcluster)  [unwired: 1 out]
          }
        }
      }
      frame "Source Image:Image Resolution (Pixel Size)" {
        n119 = case shown="True" w605 {
          tunnel: w604 -> [w613 w617]
          tunnel: w603 -> [w612 w620]
          tunnel: [w611 w619] -> w602
          tunnel: w601 -> [w610 w618]
          tunnel: [w609 w615] -> w600
          tunnel: "Image Resolution (Pixel Size)" -> [w608 w621]
          tunnel: [w606 w614] -> w599
          tunnel: w598 -> [_ w614]
          frame False {
            n120 = Get Variant Attribute(Variant=w612, name=w613, default value (empty Variant)=w608, error in=w610) -> (duplicate Variant=w611:variant, value=w607:dbl[unit], error out=w609:errorcluster)  [unwired: 1 out]
            n121 = To Variant(anything=w607) -> (Variant=w606:variant)
          }
          frame True {
            n122 = Variant To Data(type=w621, Variant=w614) -> (data=w616:dbl[unit])  [unwired: 1 in, 1 out]
            n123 = Set Variant Attribute(Variant=w620, name=w617, value=w616, error in=w618) -> (Variant out=w619:variant, error out=w615:errorcluster)  [unwired: 1 out]
          }
        }
      }
      frame "Source Image:Flatfield Correction" {
        n124 = case shown="True" w630 {
          tunnel: w629 -> [w638 w642]
          tunnel: w628 -> [w637 w645]
          tunnel: [w636 w644] -> w627
          tunnel: w626 -> [w635 w643]
          tunnel: [w634 w640] -> w625
          tunnel: "Flatfield Correction" -> [w633 w646]
          tunnel: [w631 w639] -> w624
          tunnel: w623 -> [_ w639]
          frame False {
            n125 = Get Variant Attribute(Variant=w637, name=w638, default value (empty Variant)=w633, error in=w635) -> (duplicate Variant=w636:variant, value=w632:T8, error out=w634:errorcluster)  [unwired: 1 out]
            n126 = To Variant(anything=w632) -> (Variant=w631:variant)
          }
          frame True {
            n127 = Variant To Data(type=w646, Variant=w639) -> (data=w641:T8)  [unwired: 1 in, 1 out]
            n128 = Set Variant Attribute(Variant=w645, name=w642, value=w641, error in=w643) -> (Variant out=w644:variant, error out=w640:errorcluster)  [unwired: 1 out]
          }
        }
      }
      frame "Source Image:Show Dead Left Columns Correction" {
        n129 = case shown="True" w655 {
          tunnel: w654 -> [w663 w667]
          tunnel: w653 -> [w662 w670]
          tunnel: [w661 w669] -> w652
          tunnel: w651 -> [w660 w668]
          tunnel: [w659 w665] -> w650
          tunnel: "Show Dead Left Columns Correction" -> [w658 w671]
          tunnel: [w656 w664] -> w649
          tunnel: w648 -> [_ w664]
          frame False {
            n130 = Get Variant Attribute(Variant=w662, name=w663, default value (empty Variant)=w658, error in=w660) -> (duplicate Variant=w661:variant, value=w657:bool, error out=w659:errorcluster)  [unwired: 1 out]
            n131 = To Variant(anything=w657) -> (Variant=w656:variant)
          }
          frame True {
            n132 = Variant To Data(type=w671, Variant=w664) -> (data=w666:bool)  [unwired: 1 in, 1 out]
            n133 = Set Variant Attribute(Variant=w670, name=w667, value=w666, error in=w668) -> (Variant out=w669:variant, error out=w665:errorcluster)  [unwired: 1 out]
          }
        }
      }
      frame "Source Image:Dead Left Columns Correction" {
        n134 = case shown="True" w680 {
          tunnel: w679 -> [w688 w692]
          tunnel: w678 -> [w687 w695]
          tunnel: [w686 w694] -> w677
          tunnel: w676 -> [w685 w693]
          tunnel: [w684 w690] -> w675
          tunnel: "Dead Left Columns Correction" -> [w683 w696]
          tunnel: [w681 w689] -> w674
          tunnel: w673 -> [_ w689]
          frame False {
            n135 = Get Variant Attribute(Variant=w687, name=w688, default value (empty Variant)=w683, error in=w685) -> (duplicate Variant=w686:variant, value=w682:bool, error out=w684:errorcluster)  [unwired: 1 out]
            n136 = To Variant(anything=w682) -> (Variant=w681:variant)
          }
          frame True {
            n137 = Variant To Data(type=w696, Variant=w689) -> (data=w691:bool)  [unwired: 1 in, 1 out]
            n138 = Set Variant Attribute(Variant=w695, name=w692, value=w691, error in=w693) -> (Variant out=w694:variant, error out=w690:errorcluster)  [unwired: 1 out]
          }
        }
      }
      frame "Source Image:Overlay ROI Median" {
        n139 = case shown="True" w705 {
          tunnel: w704 -> [w713 w717]
          tunnel: w703 -> [w712 w720]
          tunnel: [w711 w719] -> w702
          tunnel: w701 -> [w710 w718]
          tunnel: [w709 w715] -> w700
          tunnel: "Overlay ROI Median" -> [w708 w721]
          tunnel: [w706 w714] -> w699
          tunnel: w698 -> [_ w714]
          frame False {
            n140 = Get Variant Attribute(Variant=w712, name=w713, default value (empty Variant)=w708, error in=w710) -> (duplicate Variant=w711:variant, value=w707:bool, error out=w709:errorcluster)  [unwired: 1 out]
            n141 = To Variant(anything=w707) -> (Variant=w706:variant)
          }
          frame True {
            n142 = Variant To Data(type=w721, Variant=w714) -> (data=w716:bool)  [unwired: 1 in, 1 out]
            n143 = Set Variant Attribute(Variant=w720, name=w717, value=w716, error in=w718) -> (Variant out=w719:variant, error out=w715:errorcluster)  [unwired: 1 out]
          }
        }
      }
      frame "Source Image:Median Overlay Color" {
        n144 = case shown="True" w730 {
          tunnel: w729 -> [w738 w742]
          tunnel: w728 -> [w737 w745]
          tunnel: [w736 w744] -> w727
          tunnel: w726 -> [w735 w743]
          tunnel: [w734 w740] -> w725
          tunnel: "Median Overlay Color" -> [w733 w746]
          tunnel: [w731 w739] -> w724
          tunnel: w723 -> [_ w739]
          frame False {
            n145 = Get Variant Attribute(Variant=w737, name=w738, default value (empty Variant)=w733, error in=w735) -> (duplicate Variant=w736:variant, value=w732:u32, error out=w734:errorcluster)  [unwired: 1 out]
            n146 = To Variant(anything=w732) -> (Variant=w731:variant)
          }
          frame True {
            n147 = Variant To Data(type=w746, Variant=w739) -> (data=w741:u32)  [unwired: 1 in, 1 out]
            n148 = Set Variant Attribute(Variant=w745, name=w742, value=w741, error in=w743) -> (Variant out=w744:variant, error out=w740:errorcluster)  [unwired: 1 out]
          }
        }
      }
      frame "Data Information:Gate Width" {
        n149 = case shown="True" w755 {
          tunnel: w754 -> [w763 w767]
          tunnel: w753 -> [w762 w770]
          tunnel: [w761 w769] -> w752
          tunnel: w751 -> [w760 w768]
          tunnel: [w759 w765] -> w750
          tunnel: "Gate Width" -> [w758 w771]
          tunnel: [w756 w764] -> w749
          tunnel: w748 -> [_ w764]
          frame False {
            n150 = Get Variant Attribute(Variant=w762, name=w763, default value (empty Variant)=w758, error in=w760) -> (duplicate Variant=w761:variant, value=w757:dbl[unit], error out=w759:errorcluster)  [unwired: 1 out]
            n151 = To Variant(anything=w757) -> (Variant=w756:variant)
          }
          frame True {
            n152 = Variant To Data(type=w771, Variant=w764) -> (data=w766:dbl[unit])  [unwired: 1 in, 1 out]
            n153 = Set Variant Attribute(Variant=w770, name=w767, value=w766, error in=w768) -> (Variant out=w769:variant, error out=w765:errorcluster)  [unwired: 1 out]
          }
        }
      }
      frame "Data Information:Nanotime Gate Separation" {
        n154 = case shown="True" w780 {
          tunnel: w779 -> [w788 w792]
          tunnel: w778 -> [w787 w795]
          tunnel: [w786 w794] -> w777
          tunnel: w776 -> [w785 w793]
          tunnel: [w784 w790] -> w775
          tunnel: "Gate Separation" -> [w783 w796]
          tunnel: [w781 w789] -> w774
          tunnel: w773 -> [_ w789]
          frame False {
            n155 = Get Variant Attribute(Variant=w787, name=w788, default value (empty Variant)=w783, error in=w785) -> (duplicate Variant=w786:variant, value=w782:dbl[unit], error out=w784:errorcluster)  [unwired: 1 out]
            n156 = To Variant(anything=w782) -> (Variant=w781:variant)
          }
          frame True {
            n157 = Variant To Data(type=w796, Variant=w789) -> (data=w791:dbl[unit])  [unwired: 1 in, 1 out]
            n158 = Set Variant Attribute(Variant=w795, name=w792, value=w791, error in=w793) -> (Variant out=w794:variant, error out=w790:errorcluster)  [unwired: 1 out]
          }
        }
      }
      frame "Data Information:Gate Step" {
        n159 = case shown="True" w805 {
          tunnel: w804 -> [w813 w817]
          tunnel: w803 -> [w812 w820]
          tunnel: [w811 w819] -> w802
          tunnel: w801 -> [w810 w818]
          tunnel: [w809 w815] -> w800
          tunnel: "Gate Step" -> [w808 w821]
          tunnel: [w806 w814] -> w799
          tunnel: w798 -> [_ w814]
          frame False {
            n160 = Get Variant Attribute(Variant=w812, name=w813, default value (empty Variant)=w808, error in=w810) -> (duplicate Variant=w811:variant, value=w807:i32, error out=w809:errorcluster)  [unwired: 1 out]
            n161 = To Variant(anything=w807) -> (Variant=w806:variant)
          }
          frame True {
            n162 = Variant To Data(type=w821, Variant=w814) -> (data=w816:i32)  [unwired: 1 in, 1 out]
            n163 = Set Variant Attribute(Variant=w820, name=w817, value=w816, error in=w818) -> (Variant out=w819:variant, error out=w815:errorcluster)  [unwired: 1 out]
          }
        }
      }
      frame "Data Information:# Gates" {
        n164 = case shown="True" w830 {
          tunnel: w829 -> [w838 w842]
          tunnel: w828 -> [w837 w845]
          tunnel: [w836 w844] -> w827
          tunnel: w826 -> [w835 w843]
          tunnel: [w834 w840] -> w825
          tunnel: "# Gates" -> [w833 w846]
          tunnel: [w831 w839] -> w824
          tunnel: w823 -> [_ w839]
          frame False {
            n165 = Get Variant Attribute(Variant=w837, name=w838, default value (empty Variant)=w833, error in=w835) -> (duplicate Variant=w836:variant, value=w832:u32, error out=w834:errorcluster)  [unwired: 1 out]
            n166 = To Variant(anything=w832) -> (Variant=w831:variant)
          }
          frame True {
            n167 = Variant To Data(type=w846, Variant=w839) -> (data=w841:u32)  [unwired: 1 in, 1 out]
            n168 = Set Variant Attribute(Variant=w845, name=w842, value=w841, error in=w843) -> (Variant out=w844:variant, error out=w840:errorcluster)  [unwired: 1 out]
          }
        }
      }
      frame "Data Information:Gate Image Exposure" {
        n169 = case shown="True" w855 {
          tunnel: w854 -> [w863 w867]
          tunnel: w853 -> [w862 w870]
          tunnel: [w861 w869] -> w852
          tunnel: w851 -> [w860 w868]
          tunnel: [w859 w865] -> w850
          tunnel: "Gate Image Exposure" -> [w858 w871]
          tunnel: [w856 w864] -> w849
          tunnel: w848 -> [_ w864]
          frame False {
            n170 = Get Variant Attribute(Variant=w862, name=w863, default value (empty Variant)=w858, error in=w860) -> (duplicate Variant=w861:variant, value=w857:dbl[unit], error out=w859:errorcluster)  [unwired: 1 out]
            n171 = To Variant(anything=w857) -> (Variant=w856:variant)
          }
          frame True {
            n172 = Variant To Data(type=w871, Variant=w864) -> (data=w866:dbl[unit])  [unwired: 1 in, 1 out]
            n173 = Set Variant Attribute(Variant=w870, name=w867, value=w866, error in=w868) -> (Variant out=w869:variant, error out=w865:errorcluster)  [unwired: 1 out]
          }
        }
      }
      frame "Data Information:Gate Image Integration" {
        n174 = case shown="True" w880 {
          tunnel: w879 -> [w888 w892]
          tunnel: w878 -> [w887 w895]
          tunnel: [w886 w894] -> w877
          tunnel: w876 -> [w885 w893]
          tunnel: [w884 w890] -> w875
          tunnel: "Gate Image Integration" -> [w883 w896]
          tunnel: [w881 w889] -> w874
          tunnel: w873 -> [_ w889]
          frame False {
            n175 = Get Variant Attribute(Variant=w887, name=w888, default value (empty Variant)=w883, error in=w885) -> (duplicate Variant=w886:variant, value=w882:dbl[unit], error out=w884:errorcluster)  [unwired: 1 out]
            n176 = To Variant(anything=w882) -> (Variant=w881:variant)
          }
          frame True {
            n177 = Variant To Data(type=w896, Variant=w889) -> (data=w891:dbl[unit])  [unwired: 1 in, 1 out]
            n178 = Set Variant Attribute(Variant=w895, name=w892, value=w891, error in=w893) -> (Variant out=w894:variant, error out=w890:errorcluster)  [unwired: 1 out]
          }
        }
      }
      frame "Data Information:Gates to Skip" {
        n179 = case shown="True" w905 {
          tunnel: w904 -> [w913 w917]
          tunnel: w903 -> [w912 w920]
          tunnel: [w911 w919] -> w902
          tunnel: w901 -> [w910 w918]
          tunnel: [w909 w915] -> w900
          tunnel: "Gates to Skip" -> [w908 w921]
          tunnel: [w906 w914] -> w899
          tunnel: w898 -> [_ w914]
          frame False {
            n180 = Get Variant Attribute(Variant=w912, name=w913, default value (empty Variant)=w908, error in=w910) -> (duplicate Variant=w911:variant, value=w907:T16, error out=w909:errorcluster)  [unwired: 1 out]
            n181 = To Variant(anything=w907) -> (Variant=w906:variant)
          }
          frame True {
            n182 = Variant To Data(type=w921, Variant=w914) -> (data=w916:T16)  [unwired: 1 in, 1 out]
            n183 = Set Variant Attribute(Variant=w920, name=w917, value=w916, error in=w918) -> (Variant out=w919:variant, error out=w915:errorcluster)  [unwired: 1 out]
          }
        }
      }
      frame "Data Information:Gates to Keep" {
        n184 = case shown="True" w930 {
          tunnel: w929 -> [w938 w942]
          tunnel: w928 -> [w937 w945]
          tunnel: [w936 w944] -> w927
          tunnel: w926 -> [w935 w943]
          tunnel: [w934 w940] -> w925
          tunnel: "Gates to Keep" -> [w933 w946]
          tunnel: [w931 w939] -> w924
          tunnel: w923 -> [_ w939]
          frame False {
            n185 = Get Variant Attribute(Variant=w937, name=w938, default value (empty Variant)=w933, error in=w935) -> (duplicate Variant=w936:variant, value=w932:T14, error out=w934:errorcluster)  [unwired: 1 out]
            n186 = To Variant(anything=w932) -> (Variant=w931:variant)
          }
          frame True {
            n187 = Variant To Data(type=w946, Variant=w939) -> (data=w941:T14)  [unwired: 1 in, 1 out]
            n188 = Set Variant Attribute(Variant=w945, name=w942, value=w941, error in=w943) -> (Variant out=w944:variant, error out=w940:errorcluster)  [unwired: 1 out]
          }
        }
      }
      frame "Data Information:Define Gates to" {
        n189 = case shown="True" w955 {
          tunnel: w954 -> [w963 w967]
          tunnel: w953 -> [w962 w970]
          tunnel: [w961 w969] -> w952
          tunnel: w951 -> [w960 w968]
          tunnel: [w959 w965] -> w950
          tunnel: "Define Gates to" -> [w958 w971]
          tunnel: [w956 w964] -> w949
          tunnel: w948 -> [_ w964]
          frame False {
            n190 = Get Variant Attribute(Variant=w962, name=w963, default value (empty Variant)=w958, error in=w960) -> (duplicate Variant=w961:variant, value=w957:T15, error out=w959:errorcluster)  [unwired: 1 out]
            n191 = To Variant(anything=w957) -> (Variant=w956:variant)
          }
          frame True {
            n192 = Variant To Data(type=w971, Variant=w964) -> (data=w966:T15)  [unwired: 1 in, 1 out]
            n193 = Set Variant Attribute(Variant=w970, name=w967, value=w966, error in=w968) -> (Variant out=w969:variant, error out=w965:errorcluster)  [unwired: 1 out]
          }
        }
      }
      frame "Data Information:Channel Name" {
        n194 = case shown="True" w980 {
          tunnel: w979 -> [w988 w992]
          tunnel: w978 -> [w987 w995]
          tunnel: [w986 w994] -> w977
          tunnel: w976 -> [w985 w993]
          tunnel: [w984 w990] -> w975
          tunnel: "Channel Name" -> [w983 w996]
          tunnel: [w981 w989] -> w974
          tunnel: w973 -> [_ w989]
          frame False {
            n195 = Get Variant Attribute(Variant=w987, name=w988, default value (empty Variant)=w983, error in=w985) -> (duplicate Variant=w986:variant, value=w982:u16, error out=w984:errorcluster)  [unwired: 1 out]
            n196 = To Variant(anything=w982) -> (Variant=w981:variant)
          }
          frame True {
            n197 = Variant To Data(type=w996, Variant=w989) -> (data=w991:u16)  [unwired: 1 in, 1 out]
            n198 = Set Variant Attribute(Variant=w995, name=w992, value=w991, error in=w993) -> (Variant out=w994:variant, error out=w990:errorcluster)  [unwired: 1 out]
          }
        }
      }
      frame "Data Information:Available Channel Names" {
        n199 = case shown="True" w1005 {
          tunnel: w1004 -> [w1013 w1017]
          tunnel: w1003 -> [w1012 w1020]
          tunnel: [w1011 w1019] -> w1002
          tunnel: w1001 -> [w1010 w1018]
          tunnel: [w1009 w1015] -> w1000
          tunnel: "Available Gate Names" -> [w1008 w1021]
          tunnel: [w1006 w1014] -> w999
          tunnel: w998 -> [_ w1014]
          frame False {
            n200 = Get Variant Attribute(Variant=w1012, name=w1013, default value (empty Variant)=w1008, error in=w1010) -> (duplicate Variant=w1011:variant, value=w1007:string[], error out=w1009:errorcluster)  [unwired: 1 out]
            n201 = To Variant(anything=w1007) -> (Variant=w1006:variant)
          }
          frame True {
            n202 = Variant To Data(type=w1021, Variant=w1014) -> (data=w1016:string[])  [unwired: 1 in, 1 out]
            n203 = Set Variant Attribute(Variant=w1020, name=w1017, value=w1016, error in=w1018) -> (Variant out=w1019:variant, error out=w1015:errorcluster)  [unwired: 1 out]
          }
        }
      }
      frame "Data Information:Channel Arithmetic" {
        n204 = case shown="True" w1030 {
          tunnel: w1029 -> [w1038 w1042]
          tunnel: w1028 -> [w1037 w1045]
          tunnel: [w1036 w1044] -> w1027
          tunnel: w1026 -> [w1035 w1043]
          tunnel: [w1034 w1040] -> w1025
          tunnel: "Channel Arithmetic" -> [w1033 w1046]
          tunnel: [w1031 w1039] -> w1024
          tunnel: w1023 -> [_ w1039]
          frame False {
            n205 = Get Variant Attribute(Variant=w1037, name=w1038, default value (empty Variant)=w1033, error in=w1035) -> (duplicate Variant=w1036:variant, value=w1032:T13, error out=w1034:errorcluster)  [unwired: 1 out]
            n206 = To Variant(anything=w1032) -> (Variant=w1031:variant)
          }
          frame True {
            n207 = Variant To Data(type=w1046, Variant=w1039) -> (data=w1041:T13)  [unwired: 1 in, 1 out]
            n208 = Set Variant Attribute(Variant=w1045, name=w1042, value=w1041, error in=w1043) -> (Variant out=w1044:variant, error out=w1040:errorcluster)  [unwired: 1 out]
          }
        }
      }
      frame "Data Information:Background File Subtraction" {
        n209 = case shown="True" w1055 {
          tunnel: w1054 -> [w1063 w1067]
          tunnel: w1053 -> [w1062 w1070]
          tunnel: [w1061 w1069] -> w1052
          tunnel: w1051 -> [w1060 w1068]
          tunnel: [w1059 w1065] -> w1050
          tunnel: "Background File Subtraction" -> [w1058 w1071]
          tunnel: [w1056 w1064] -> w1049
          tunnel: w1048 -> [_ w1064]
          frame False {
            n210 = Get Variant Attribute(Variant=w1062, name=w1063, default value (empty Variant)=w1058, error in=w1060) -> (duplicate Variant=w1061:variant, value=w1057:bool, error out=w1059:errorcluster)  [unwired: 1 out]
            n211 = To Variant(anything=w1057) -> (Variant=w1056:variant)
          }
          frame True {
            n212 = Variant To Data(type=w1071, Variant=w1064) -> (data=w1066:bool)  [unwired: 1 in, 1 out]
            n213 = Set Variant Attribute(Variant=w1070, name=w1067, value=w1066, error in=w1068) -> (Variant out=w1069:variant, error out=w1065:errorcluster)  [unwired: 1 out]
          }
        }
      }
      frame "Data Information:Background File" {
        n214 = case shown="True" w1080 {
          tunnel: w1079 -> [w1088 w1092]
          tunnel: w1078 -> [w1087 w1095]
          tunnel: [w1086 w1094] -> w1077
          tunnel: w1076 -> [w1085 w1093]
          tunnel: [w1084 w1090] -> w1075
          tunnel: "Background File" -> [w1083 w1096]
          tunnel: [w1081 w1089] -> w1074
          tunnel: w1073 -> [_ w1089]
          frame False {
            n215 = Get Variant Attribute(Variant=w1087, name=w1088, default value (empty Variant)=w1083, error in=w1085) -> (duplicate Variant=w1086:variant, value=w1082:path, error out=w1084:errorcluster)  [unwired: 1 out]
            n216 = To Variant(anything=w1082) -> (Variant=w1081:variant)
          }
          frame True {
            n217 = Variant To Data(type=w1096, Variant=w1089) -> (data=w1091:path)  [unwired: 1 in, 1 out]
            n218 = Set Variant Attribute(Variant=w1095, name=w1092, value=w1091, error in=w1093) -> (Variant out=w1094:variant, error out=w1090:errorcluster)  [unwired: 1 out]
          }
        }
      }
      frame "Data Information:Background Scaling Factor" {
        n219 = case shown="True" w1105 {
          tunnel: w1104 -> [w1113 w1117]
          tunnel: w1103 -> [w1112 w1120]
          tunnel: [w1111 w1119] -> w1102
          tunnel: w1101 -> [w1110 w1118]
          tunnel: [w1109 w1115] -> w1100
          tunnel: "Background Scaling Factor" -> [w1108 w1121]
          tunnel: [w1106 w1114] -> w1099
          tunnel: w1098 -> [_ w1114]
          frame False {
            n220 = Get Variant Attribute(Variant=w1112, name=w1113, default value (empty Variant)=w1108, error in=w1110) -> (duplicate Variant=w1111:variant, value=w1107:dbl, error out=w1109:errorcluster)  [unwired: 1 out]
            n221 = To Variant(anything=w1107) -> (Variant=w1106:variant)
          }
          frame True {
            n222 = Variant To Data(type=w1121, Variant=w1114) -> (data=w1116:dbl)  [unwired: 1 in, 1 out]
            n223 = Set Variant Attribute(Variant=w1120, name=w1117, value=w1116, error in=w1118) -> (Variant out=w1119:variant, error out=w1115:errorcluster)  [unwired: 1 out]
          }
        }
      }
      frame "Data Information:Background Pile-up Correction" {
        n224 = case shown="True" w1130 {
          tunnel: w1129 -> [w1138 w1142]
          tunnel: w1128 -> [w1137 w1145]
          tunnel: [w1136 w1144] -> w1127
          tunnel: w1126 -> [w1135 w1143]
          tunnel: [w1134 w1140] -> w1125
          tunnel: "Background Pile-up Correction" -> [w1133 w1146]
          tunnel: [w1131 w1139] -> w1124
          tunnel: w1123 -> [_ w1139]
          frame False {
            n225 = Get Variant Attribute(Variant=w1137, name=w1138, default value (empty Variant)=w1133, error in=w1135) -> (duplicate Variant=w1136:variant, value=w1132:bool, error out=w1134:errorcluster)  [unwired: 1 out]
            n226 = To Variant(anything=w1132) -> (Variant=w1131:variant)
          }
          frame True {
            n227 = Variant To Data(type=w1146, Variant=w1139) -> (data=w1141:bool)  [unwired: 1 in, 1 out]
            n228 = Set Variant Attribute(Variant=w1145, name=w1142, value=w1141, error in=w1143) -> (Variant out=w1144:variant, error out=w1140:errorcluster)  [unwired: 1 out]
          }
        }
      }
      frame "Data Information:Background Pixel Well Capacity" {
        n229 = case shown="True" w1155 {
          tunnel: w1154 -> [w1163 w1167]
          tunnel: w1153 -> [w1162 w1170]
          tunnel: [w1161 w1169] -> w1152
          tunnel: w1151 -> [w1160 w1168]
          tunnel: [w1159 w1165] -> w1150
          tunnel: "Background Pixel Well Capacity" -> [w1158 w1171]
          tunnel: [w1156 w1164] -> w1149
          tunnel: w1148 -> [_ w1164]
          frame False {
            n230 = Get Variant Attribute(Variant=w1162, name=w1163, default value (empty Variant)=w1158, error in=w1160) -> (duplicate Variant=w1161:variant, value=w1157:u32, error out=w1159:errorcluster)  [unwired: 1 out]
            n231 = To Variant(anything=w1157) -> (Variant=w1156:variant)
          }
          frame True {
            n232 = Variant To Data(type=w1171, Variant=w1164) -> (data=w1166:u32)  [unwired: 1 in, 1 out]
            n233 = Set Variant Attribute(Variant=w1170, name=w1167, value=w1166, error in=w1168) -> (Variant out=w1169:variant, error out=w1165:errorcluster)  [unwired: 1 out]
          }
        }
      }
      frame "Data Information:Laser Period" {
        n234 = case shown="False" w1180 {
          tunnel: w1179 -> [w1188 w1192]
          tunnel: w1178 -> [w1187 w1195]
          tunnel: [w1186 w1194] -> w1177
          tunnel: w1176 -> [w1185 w1193]
          tunnel: [w1184 w1190] -> w1175
          tunnel: "Laser Period" -> [w1183 w1196]
          tunnel: [w1181 w1189] -> w1174
          tunnel: w1173 -> [_ w1189]
          frame False {
            n235 = Get Variant Attribute(Variant=w1187, name=w1188, default value (empty Variant)=w1183, error in=w1185) -> (duplicate Variant=w1186:variant, value=w1182:dbl[unit], error out=w1184:errorcluster)  [unwired: 1 out]
            n236 = To Variant(anything=w1182) -> (Variant=w1181:variant)
          }
          frame True {
            n237 = Variant To Data(type=w1196, Variant=w1189) -> (data=w1191:dbl[unit])  [unwired: 1 in, 1 out]
            n238 = Set Variant Attribute(Variant=w1195, name=w1192, value=w1191, error in=w1193) -> (Variant out=w1194:variant, error out=w1190:errorcluster)  [unwired: 1 out]
          }
        }
      }
      frame "Data Information:SYNC Period" {
        n239 = case shown="False" w1205 {
          tunnel: w1204 -> [w1213 w1217]
          tunnel: w1203 -> [w1212 w1220]
          tunnel: [w1211 w1219] -> w1202
          tunnel: w1201 -> [w1210 w1218]
          tunnel: [w1209 w1215] -> w1200
          tunnel: "SYNC Period" -> [w1208 w1221]
          tunnel: [w1206 w1214] -> w1199
          tunnel: w1198 -> [_ w1214]
          frame False {
            n240 = Get Variant Attribute(Variant=w1212, name=w1213, default value (empty Variant)=w1208, error in=w1210) -> (duplicate Variant=w1211:variant, value=w1207:dbl[unit], error out=w1209:errorcluster)  [unwired: 1 out]
            n241 = To Variant(anything=w1207) -> (Variant=w1206:variant)
          }
          frame True {
            n242 = Variant To Data(type=w1221, Variant=w1214) -> (data=w1216:dbl[unit])  [unwired: 1 in, 1 out]
            n243 = Set Variant Attribute(Variant=w1220, name=w1217, value=w1216, error in=w1218) -> (Variant out=w1219:variant, error out=w1215:errorcluster)  [unwired: 1 out]
          }
        }
      }
      frame "Data Information:Pile-up Correction" {
        n244 = case shown="True" w1230 {
          tunnel: w1229 -> [w1238 w1242]
          tunnel: w1228 -> [w1237 w1245]
          tunnel: [w1236 w1244] -> w1227
          tunnel: w1226 -> [w1235 w1243]
          tunnel: [w1234 w1240] -> w1225
          tunnel: "Pile-up Correction" -> [w1233 w1246]
          tunnel: [w1231 w1239] -> w1224
          tunnel: w1223 -> [_ w1239]
          frame False {
            n245 = Get Variant Attribute(Variant=w1237, name=w1238, default value (empty Variant)=w1233, error in=w1235) -> (duplicate Variant=w1236:variant, value=w1232:bool, error out=w1234:errorcluster)  [unwired: 1 out]
            n246 = To Variant(anything=w1232) -> (Variant=w1231:variant)
          }
          frame True {
            n247 = Variant To Data(type=w1246, Variant=w1239) -> (data=w1241:bool)  [unwired: 1 in, 1 out]
            n248 = Set Variant Attribute(Variant=w1245, name=w1242, value=w1241, error in=w1243) -> (Variant out=w1244:variant, error out=w1240:errorcluster)  [unwired: 1 out]
          }
        }
      }
      frame "Data Information:Pixel Well Capacity" {
        n249 = case shown="True" w1255 {
          tunnel: w1254 -> [w1263 w1267]
          tunnel: w1253 -> [w1262 w1270]
          tunnel: [w1261 w1269] -> w1252
          tunnel: w1251 -> [w1260 w1268]
          tunnel: [w1259 w1265] -> w1250
          tunnel: "Pixel Well Capacity" -> [w1258 w1271]
          tunnel: [w1256 w1264] -> w1249
          tunnel: w1248 -> [_ w1264]
          frame False {
            n250 = Get Variant Attribute(Variant=w1262, name=w1263, default value (empty Variant)=w1258, error in=w1260) -> (duplicate Variant=w1261:variant, value=w1257:i32, error out=w1259:errorcluster)  [unwired: 1 out]
            n251 = To Variant(anything=w1257) -> (Variant=w1256:variant)
          }
          frame True {
            n252 = Variant To Data(type=w1271, Variant=w1264) -> (data=w1266:i32)  [unwired: 1 in, 1 out]
            n253 = Set Variant Attribute(Variant=w1270, name=w1267, value=w1266, error in=w1268) -> (Variant out=w1269:variant, error out=w1265:errorcluster)  [unwired: 1 out]
          }
        }
      }
      frame "Data Information:Dataset Scaling Factor" {
        n254 = case shown="True" w1280 {
          tunnel: w1279 -> [w1288 w1292]
          tunnel: w1278 -> [w1287 w1295]
          tunnel: [w1286 w1294] -> w1277
          tunnel: w1276 -> [w1285 w1293]
          tunnel: [w1284 w1290] -> w1275
          tunnel: "Dataset Scaling Factor" -> [w1283 w1296]
          tunnel: [w1281 w1289] -> w1274
          tunnel: w1273 -> [_ w1289]
          frame False {
            n255 = Get Variant Attribute(Variant=w1287, name=w1288, default value (empty Variant)=w1283, error in=w1285) -> (duplicate Variant=w1286:variant, value=w1282:dbl, error out=w1284:errorcluster)  [unwired: 1 out]
            n256 = To Variant(anything=w1282) -> (Variant=w1281:variant)
          }
          frame True {
            n257 = Variant To Data(type=w1296, Variant=w1289) -> (data=w1291:dbl)  [unwired: 1 in, 1 out]
            n258 = Set Variant Attribute(Variant=w1295, name=w1292, value=w1291, error in=w1293) -> (Variant out=w1294:variant, error out=w1290:errorcluster)  [unwired: 1 out]
          }
        }
      }
      frame "Data Information:Macrotime Gate Separation" {
        n259 = case shown="True" w1305 {
          tunnel: w1304 -> [w1313 w1317]
          tunnel: w1303 -> [w1312 w1320]
          tunnel: [w1311 w1319] -> w1302
          tunnel: w1301 -> [w1310 w1318]
          tunnel: [w1309 w1315] -> w1300
          tunnel: "Mscrotime Gate Separation" -> [w1308 w1321]
          tunnel: [w1306 w1314] -> w1299
          tunnel: w1298 -> [_ w1314]
          frame False {
            n260 = Get Variant Attribute(Variant=w1312, name=w1313, default value (empty Variant)=w1308, error in=w1310) -> (duplicate Variant=w1311:variant, value=w1307:dbl[unit], error out=w1309:errorcluster)  [unwired: 1 out]
            n261 = To Variant(anything=w1307) -> (Variant=w1306:variant)
          }
          frame True {
            n262 = Variant To Data(type=w1321, Variant=w1314) -> (data=w1316:dbl[unit])  [unwired: 1 in, 1 out]
            n263 = Set Variant Attribute(Variant=w1320, name=w1317, value=w1316, error in=w1318) -> (Variant out=w1319:variant, error out=w1315:errorcluster)  [unwired: 1 out]
          }
        }
      }
      frame "Fluorescence Decay_Decay Pre-Processing:Reverse Gates" {
        n264 = case shown="True" w1330 {
          tunnel: w1329 -> [w1338 w1342]
          tunnel: w1328 -> [w1337 w1345]
          tunnel: [w1336 w1344] -> w1327
          tunnel: w1326 -> [w1335 w1343]
          tunnel: [w1334 w1340] -> w1325
          tunnel: "Reverse Gates" -> [w1333 w1346]
          tunnel: [w1331 w1339] -> w1324
          tunnel: w1323 -> [_ w1339]
          frame False {
            n265 = Get Variant Attribute(Variant=w1337, name=w1338, default value (empty Variant)=w1333, error in=w1335) -> (duplicate Variant=w1336:variant, value=w1332:bool, error out=w1334:errorcluster)  [unwired: 1 out]
            n266 = To Variant(anything=w1332) -> (Variant=w1331:variant)
          }
          frame True {
            n267 = Variant To Data(type=w1346, Variant=w1339) -> (data=w1341:bool)  [unwired: 1 in, 1 out]
            n268 = Set Variant Attribute(Variant=w1345, name=w1342, value=w1341, error in=w1343) -> (Variant out=w1344:variant, error out=w1340:errorcluster)  [unwired: 1 out]
          }
        }
      }
      frame "Fluorescence Decay_Decay Pre-Processing:Verbose Decay Pre-Processing" {
        n269 = case shown="True" w1355 {
          tunnel: w1354 -> [w1363 w1367]
          tunnel: w1353 -> [w1362 w1370]
          tunnel: [w1361 w1369] -> w1352
          tunnel: w1351 -> [w1360 w1368]
          tunnel: [w1359 w1365] -> w1350
          tunnel: "Verbose Decay Pre-Processing" -> [w1358 w1371]
          tunnel: [w1356 w1364] -> w1349
          tunnel: w1348 -> [_ w1364]
          frame False {
            n270 = Get Variant Attribute(Variant=w1362, name=w1363, default value (empty Variant)=w1358, error in=w1360) -> (duplicate Variant=w1361:variant, value=w1357:bool, error out=w1359:errorcluster)  [unwired: 1 out]
            n271 = To Variant(anything=w1357) -> (Variant=w1356:variant)
          }
          frame True {
            n272 = Variant To Data(type=w1371, Variant=w1364) -> (data=w1366:bool)  [unwired: 1 in, 1 out]
            n273 = Set Variant Attribute(Variant=w1370, name=w1367, value=w1366, error in=w1368) -> (Variant out=w1369:variant, error out=w1365:errorcluster)  [unwired: 1 out]
          }
        }
      }
      frame "Fluorescence Decay_Decay Pre-Processing:Use Decay Pre-Processing" {
        n274 = case shown="True" w1380 {
          tunnel: w1379 -> [w1388 w1392]
          tunnel: w1378 -> [w1387 w1395]
          tunnel: [w1386 w1394] -> w1377
          tunnel: w1376 -> [w1385 w1393]
          tunnel: [w1384 w1390] -> w1375
          tunnel: "Use Decay Pre-Processing" -> [w1383 w1396]
          tunnel: [w1381 w1389] -> w1374
          tunnel: w1373 -> [_ w1389]
          frame False {
            n275 = Get Variant Attribute(Variant=w1387, name=w1388, default value (empty Variant)=w1383, error in=w1385) -> (duplicate Variant=w1386:variant, value=w1382:bool, error out=w1384:errorcluster)  [unwired: 1 out]
            n276 = To Variant(anything=w1382) -> (Variant=w1381:variant)
          }
          frame True {
            n277 = Variant To Data(type=w1396, Variant=w1389) -> (data=w1391:bool)  [unwired: 1 in, 1 out]
            n278 = Set Variant Attribute(Variant=w1395, name=w1392, value=w1391, error in=w1393) -> (Variant out=w1394:variant, error out=w1390:errorcluster)  [unwired: 1 out]
          }
        }
      }
      frame "Fluorescence Decay_Decay Pre-Processing:Background Subtraction" {
        n279 = case shown="True" w1405 {
          tunnel: w1404 -> [w1413 w1417]
          tunnel: w1403 -> [w1412 w1420]
          tunnel: [w1411 w1419] -> w1402
          tunnel: w1401 -> [w1410 w1418]
          tunnel: [w1409 w1415] -> w1400
          tunnel: "Background Subtraction" -> [w1408 w1421]
          tunnel: [w1406 w1414] -> w1399
          tunnel: w1398 -> [_ w1414]
          frame False {
            n280 = Get Variant Attribute(Variant=w1412, name=w1413, default value (empty Variant)=w1408, error in=w1410) -> (duplicate Variant=w1411:variant, value=w1407:bool, error out=w1409:errorcluster)  [unwired: 1 out]
            n281 = To Variant(anything=w1407) -> (Variant=w1406:variant)
          }
          frame True {
            n282 = Variant To Data(type=w1421, Variant=w1414) -> (data=w1416:bool)  [unwired: 1 in, 1 out]
            n283 = Set Variant Attribute(Variant=w1420, name=w1417, value=w1416, error in=w1418) -> (Variant out=w1419:variant, error out=w1415:errorcluster)  [unwired: 1 out]
          }
        }
      }
      frame "Fluorescence Decay_Decay Pre-Processing:Background Definition Range" {
        n284 = case shown="True" w1430 {
          tunnel: w1429 -> [w1438 w1442]
          tunnel: w1428 -> [w1437 w1445]
          tunnel: [w1436 w1444] -> w1427
          tunnel: w1426 -> [w1435 w1443]
          tunnel: [w1434 w1440] -> w1425
          tunnel: "Background Definition Range" -> [w1433 w1446]
          tunnel: [w1431 w1439] -> w1424
          tunnel: w1423 -> [_ w1439]
          frame False {
            n285 = Get Variant Attribute(Variant=w1437, name=w1438, default value (empty Variant)=w1433, error in=w1435) -> (duplicate Variant=w1436:variant, value=w1432:T19, error out=w1434:errorcluster)  [unwired: 1 out]
            n286 = To Variant(anything=w1432) -> (Variant=w1431:variant)
          }
          frame True {
            n287 = Variant To Data(type=w1446, Variant=w1439) -> (data=w1441:T19)  [unwired: 1 in, 1 out]
            n288 = Set Variant Attribute(Variant=w1445, name=w1442, value=w1441, error in=w1443) -> (Variant out=w1444:variant, error out=w1440:errorcluster)  [unwired: 1 out]
          }
        }
      }
      frame "Fluorescence Decay_Decay Pre-Processing:Baseline Subtraction Method" {
        n289 = case shown="True" w1455 {
          tunnel: w1454 -> [w1463 w1467]
          tunnel: w1453 -> [w1462 w1470]
          tunnel: [w1461 w1469] -> w1452
          tunnel: w1451 -> [w1460 w1468]
          tunnel: [w1459 w1465] -> w1450
          tunnel: "Baseline Subtraction Method" -> [w1458 w1471]
          tunnel: [w1456 w1464] -> w1449
          tunnel: w1448 -> [_ w1464]
          frame False {
            n290 = Get Variant Attribute(Variant=w1462, name=w1463, default value (empty Variant)=w1458, error in=w1460) -> (duplicate Variant=w1461:variant, value=w1457:T18, error out=w1459:errorcluster)  [unwired: 1 out]
            n291 = To Variant(anything=w1457) -> (Variant=w1456:variant)
          }
          frame True {
            n292 = Variant To Data(type=w1471, Variant=w1464) -> (data=w1466:T18)  [unwired: 1 in, 1 out]
            n293 = Set Variant Attribute(Variant=w1470, name=w1467, value=w1466, error in=w1468) -> (Variant out=w1469:variant, error out=w1465:errorcluster)  [unwired: 1 out]
          }
        }
      }
      frame "Fluorescence Decay_Decay Pre-Processing:Decay Pre-Processing Operations Order" {
        n294 = case shown="True" w1481 {
          tunnel: w1480 -> [w1489 w1496]
          tunnel: w1479 -> [w1488 w1499]
          tunnel: [w1487 w1498] -> w1478
          tunnel: w1477 -> [w1486 w1497]
          tunnel: [w1485 w1495] -> w1476
          tunnel: "Decay Pre-Processing Operations Order" -> [w1484 w1500]
          tunnel: [w1482 w1494] -> w1475
          tunnel: w1474 -> [_ w1494]
          tunnel: w1472 -> [_ w1490]
          frame False {
            n295 = Get Variant Attribute(Variant=w1488, name=w1489, default value (empty Variant)=w1484, error in=w1486) -> (duplicate Variant=w1487:variant, value=w1483:string[], error out=w1485:errorcluster)  [unwired: 1 out]
            n296 = To Variant(anything=w1483) -> (Variant=w1482:variant)
          }
          frame True {
            n297 = Variant To Data(type=w1500, Variant=w1494) -> (data=w1492:string[])  [unwired: 1 in, 1 out]
            n298 = Array Size(array=w1492) -> (size(s)=w1491:i32)
            n299 = case shown="8" w1491 {
              tunnel: w1492 -> [w1501 _]
              tunnel: [w1501 w1502] -> w1493
              tunnel: w1490 -> [_ w1502]
              frame 8 {
              }
              frame 0, Default {
              }
            }
            n300 = Set Variant Attribute(Variant=w1499, name=w1496, value=w1493, error in=w1497) -> (Variant out=w1498:variant, error out=w1495:errorcluster)  [unwired: 1 out]
          }
        }
      }
      frame "Source Image:Image Pre-Processing Operations Order" {
        n301 = case shown="True" w1512 {
          tunnel: w1511 -> [w1520 w1527]
          tunnel: w1510 -> [w1519 w1530]
          tunnel: [w1518 w1529] -> w1509
          tunnel: w1508 -> [w1517 w1528]
          tunnel: [w1516 w1526] -> w1507
          tunnel: "Image Pre-Processing Operations Order" -> [w1515 w1531]
          tunnel: [w1513 w1525] -> w1506
          tunnel: w1505 -> [_ w1525]
          tunnel: w1503 -> [_ w1521]
          frame False {
            n302 = Get Variant Attribute(Variant=w1519, name=w1520, default value (empty Variant)=w1515, error in=w1517) -> (duplicate Variant=w1518:variant, value=w1514:string[], error out=w1516:errorcluster)  [unwired: 1 out]
            n303 = To Variant(anything=w1514) -> (Variant=w1513:variant)
          }
          frame True {
            n304 = Variant To Data(type=w1531, Variant=w1525) -> (data=w1523:string[])  [unwired: 1 in, 1 out]
            n305 = Array Size(array=w1523) -> (size(s)=w1522:i32)
            n306 = case shown="5, 6" w1522 {
              tunnel: w1523 -> [w1532 _]
              tunnel: [w1532 w1533] -> w1524
              tunnel: w1521 -> [_ w1533]
              frame 5, 6 {
              }
              frame 0, Default {
              }
            }
            n307 = Set Variant Attribute(Variant=w1530, name=w1527, value=w1524, error in=w1528) -> (Variant out=w1529:variant, error out=w1526:errorcluster)  [unwired: 1 out]
          }
        }
      }
      frame "Fluorescence Decay_Decay Pre-Processing:Smoothing Parameter" {
        n308 = case shown="True" w1542 {
          tunnel: w1541 -> [w1550 w1554]
          tunnel: w1540 -> [w1549 w1557]
          tunnel: [w1548 w1556] -> w1539
          tunnel: w1538 -> [w1547 w1555]
          tunnel: [w1546 w1552] -> w1537
          tunnel: "Smoothing Parameter" -> [w1545 w1558]
          tunnel: [w1543 w1551] -> w1536
          tunnel: w1535 -> [_ w1551]
          frame False {
            n309 = Get Variant Attribute(Variant=w1549, name=w1550, default value (empty Variant)=w1545, error in=w1547) -> (duplicate Variant=w1548:variant, value=w1544:dbl, error out=w1546:errorcluster)  [unwired: 1 out]
            n310 = To Variant(anything=w1544) -> (Variant=w1543:variant)
          }
          frame True {
            n311 = Variant To Data(type=w1558, Variant=w1551) -> (data=w1553:dbl)  [unwired: 1 in, 1 out]
            n312 = Set Variant Attribute(Variant=w1557, name=w1554, value=w1553, error in=w1555) -> (Variant out=w1556:variant, error out=w1552:errorcluster)  [unwired: 1 out]
          }
        }
      }
      frame "Fluorescence Decay_Decay Pre-Processing:Shift Decay" {
        n313 = case shown="True" w1567 {
          tunnel: w1566 -> [w1575 w1579]
          tunnel: w1565 -> [w1574 w1582]
          tunnel: [w1573 w1581] -> w1564
          tunnel: w1563 -> [w1572 w1580]
          tunnel: [w1571 w1577] -> w1562
          tunnel: "Shift Decay" -> [w1570 w1583]
          tunnel: [w1568 w1576] -> w1561
          tunnel: w1560 -> [_ w1576]
          frame False {
            n314 = Get Variant Attribute(Variant=w1574, name=w1575, default value (empty Variant)=w1570, error in=w1572) -> (duplicate Variant=w1573:variant, value=w1569:bool, error out=w1571:errorcluster)  [unwired: 1 out]
            n315 = To Variant(anything=w1569) -> (Variant=w1568:variant)
          }
          frame True {
            n316 = Variant To Data(type=w1583, Variant=w1576) -> (data=w1578:bool)  [unwired: 1 in, 1 out]
            n317 = Set Variant Attribute(Variant=w1582, name=w1579, value=w1578, error in=w1580) -> (Variant out=w1581:variant, error out=w1577:errorcluster)  [unwired: 1 out]
          }
        }
      }
      frame "Fluorescence Decay_Decay Pre-Processing:Decay Shift Parameters" {
        n318 = case shown="True" w1592 {
          tunnel: w1591 -> [w1600 w1604]
          tunnel: w1590 -> [w1599 w1607]
          tunnel: [w1598 w1606] -> w1589
          tunnel: w1588 -> [w1597 w1605]
          tunnel: [w1596 w1602] -> w1587
          tunnel: "Decay Shift Parameters" -> [w1595 w1608]
          tunnel: [w1593 w1601] -> w1586
          tunnel: w1585 -> [_ w1601]
          frame False {
            n319 = Get Variant Attribute(Variant=w1599, name=w1600, default value (empty Variant)=w1595, error in=w1597) -> (duplicate Variant=w1598:variant, value=w1594:T20, error out=w1596:errorcluster)  [unwired: 1 out]
            n320 = To Variant(anything=w1594) -> (Variant=w1593:variant)
          }
          frame True {
            n321 = Variant To Data(type=w1608, Variant=w1601) -> (data=w1603:T20)  [unwired: 1 in, 1 out]
            n322 = Set Variant Attribute(Variant=w1607, name=w1604, value=w1603, error in=w1605) -> (Variant out=w1606:variant, error out=w1602:errorcluster)  [unwired: 1 out]
          }
        }
      }
      frame "Fluorescence Decay_Decay Pre-Processing:Fold Decay" {
        n323 = case shown="True" w1617 {
          tunnel: w1616 -> [w1625 w1629]
          tunnel: w1615 -> [w1624 w1632]
          tunnel: [w1623 w1631] -> w1614
          tunnel: w1613 -> [w1622 w1630]
          tunnel: [w1621 w1627] -> w1612
          tunnel: "Fold Decay" -> [w1620 w1633]
          tunnel: [w1618 w1626] -> w1611
          tunnel: w1610 -> [_ w1626]
          frame False {
            n324 = Get Variant Attribute(Variant=w1624, name=w1625, default value (empty Variant)=w1620, error in=w1622) -> (duplicate Variant=w1623:variant, value=w1619:bool, error out=w1621:errorcluster)  [unwired: 1 out]
            n325 = To Variant(anything=w1619) -> (Variant=w1618:variant)
          }
          frame True {
            n326 = Variant To Data(type=w1633, Variant=w1626) -> (data=w1628:bool)  [unwired: 1 in, 1 out]
            n327 = Set Variant Attribute(Variant=w1632, name=w1629, value=w1628, error in=w1630) -> (Variant out=w1631:variant, error out=w1627:errorcluster)  [unwired: 1 out]
          }
        }
      }
      frame "Fluorescence Decay_Decay Pre-Processing:# Folds" {
        n328 = case shown="True" w1642 {
          tunnel: w1641 -> [w1650 w1654]
          tunnel: w1640 -> [w1649 w1657]
          tunnel: [w1648 w1656] -> w1639
          tunnel: w1638 -> [w1647 w1655]
          tunnel: [w1646 w1652] -> w1637
          tunnel: "# Folds" -> [w1645 w1658]
          tunnel: [w1643 w1651] -> w1636
          tunnel: w1635 -> [_ w1651]
          frame False {
            n329 = Get Variant Attribute(Variant=w1649, name=w1650, default value (empty Variant)=w1645, error in=w1647) -> (duplicate Variant=w1648:variant, value=w1644:u32, error out=w1646:errorcluster)  [unwired: 1 out]
            n330 = To Variant(anything=w1644) -> (Variant=w1643:variant)
          }
          frame True {
            n331 = Variant To Data(type=w1658, Variant=w1651) -> (data=w1653:u32)  [unwired: 1 in, 1 out]
            n332 = Set Variant Attribute(Variant=w1657, name=w1654, value=w1653, error in=w1655) -> (Variant out=w1656:variant, error out=w1652:errorcluster)  [unwired: 1 out]
          }
        }
      }
      frame "Fluorescence Decay_Decay Pre-Processing:1-Normalize Decay" {
        n333 = case shown="True" w1667 {
          tunnel: w1666 -> [w1675 w1679]
          tunnel: w1665 -> [w1674 w1682]
          tunnel: [w1673 w1681] -> w1664
          tunnel: w1663 -> [w1672 w1680]
          tunnel: [w1671 w1677] -> w1662
          tunnel: "1-Normalize Decay" -> [w1670 w1683]
          tunnel: [w1668 w1676] -> w1661
          tunnel: w1660 -> [_ w1676]
          frame False {
            n334 = Get Variant Attribute(Variant=w1674, name=w1675, default value (empty Variant)=w1670, error in=w1672) -> (duplicate Variant=w1673:variant, value=w1669:bool, error out=w1671:errorcluster)  [unwired: 1 out]
            n335 = To Variant(anything=w1669) -> (Variant=w1668:variant)
          }
          frame True {
            n336 = Variant To Data(type=w1683, Variant=w1676) -> (data=w1678:bool)  [unwired: 1 in, 1 out]
            n337 = Set Variant Attribute(Variant=w1682, name=w1679, value=w1678, error in=w1680) -> (Variant out=w1681:variant, error out=w1677:errorcluster)  [unwired: 1 out]
          }
        }
      }
      frame "Fluorescence Decay_Decay Pre-Processing:[0-1]-Normalize Decay" {
        n338 = case shown="True" w1692 {
          tunnel: w1691 -> [w1700 w1704]
          tunnel: w1690 -> [w1699 w1707]
          tunnel: [w1698 w1706] -> w1689
          tunnel: w1688 -> [w1697 w1705]
          tunnel: [w1696 w1702] -> w1687
          tunnel: "[0-1]-Normalize Decay" -> [w1695 w1708]
          tunnel: [w1693 w1701] -> w1686
          tunnel: w1685 -> [_ w1701]
          frame False {
            n339 = Get Variant Attribute(Variant=w1699, name=w1700, default value (empty Variant)=w1695, error in=w1697) -> (duplicate Variant=w1698:variant, value=w1694:bool, error out=w1696:errorcluster)  [unwired: 1 out]
            n340 = To Variant(anything=w1694) -> (Variant=w1693:variant)
          }
          frame True {
            n341 = Variant To Data(type=w1708, Variant=w1701) -> (data=w1703:bool)  [unwired: 1 in, 1 out]
            n342 = Set Variant Attribute(Variant=w1707, name=w1704, value=w1703, error in=w1705) -> (Variant out=w1706:variant, error out=w1702:errorcluster)  [unwired: 1 out]
          }
        }
      }
      frame "Fluorescence Decay_Decay Pre-Processing:Smoothen Decay" {
        n343 = case shown="True" w1717 {
          tunnel: w1716 -> [w1725 w1729]
          tunnel: w1715 -> [w1724 w1732]
          tunnel: [w1723 w1731] -> w1714
          tunnel: w1713 -> [w1722 w1730]
          tunnel: [w1721 w1727] -> w1712
          tunnel: "Smoothen Decay" -> [w1720 w1733]
          tunnel: [w1718 w1726] -> w1711
          tunnel: w1710 -> [_ w1726]
          frame False {
            n344 = Get Variant Attribute(Variant=w1724, name=w1725, default value (empty Variant)=w1720, error in=w1722) -> (duplicate Variant=w1723:variant, value=w1719:bool, error out=w1721:errorcluster)  [unwired: 1 out]
            n345 = To Variant(anything=w1719) -> (Variant=w1718:variant)
          }
          frame True {
            n346 = Variant To Data(type=w1733, Variant=w1726) -> (data=w1728:bool)  [unwired: 1 in, 1 out]
            n347 = Set Variant Attribute(Variant=w1732, name=w1729, value=w1728, error in=w1730) -> (Variant out=w1731:variant, error out=w1727:errorcluster)  [unwired: 1 out]
          }
        }
      }
      frame "Fluorescence Decay_Decay Pre-Processing:Extrapolate Decay" {
        n348 = case shown="True" w1742 {
          tunnel: w1741 -> [w1750 w1754]
          tunnel: w1740 -> [w1749 w1757]
          tunnel: [w1748 w1756] -> w1739
          tunnel: w1738 -> [w1747 w1755]
          tunnel: [w1746 w1752] -> w1737
          tunnel: "Extrapolate Decay" -> [w1745 w1758]
          tunnel: [w1743 w1751] -> w1736
          tunnel: w1735 -> [_ w1751]
          frame False {
            n349 = Get Variant Attribute(Variant=w1749, name=w1750, default value (empty Variant)=w1745, error in=w1747) -> (duplicate Variant=w1748:variant, value=w1744:bool, error out=w1746:errorcluster)  [unwired: 1 out]
            n350 = To Variant(anything=w1744) -> (Variant=w1743:variant)
          }
          frame True {
            n351 = Variant To Data(type=w1758, Variant=w1751) -> (data=w1753:bool)  [unwired: 1 in, 1 out]
            n352 = Set Variant Attribute(Variant=w1757, name=w1754, value=w1753, error in=w1755) -> (Variant out=w1756:variant, error out=w1752:errorcluster)  [unwired: 1 out]
          }
        }
      }
      frame "Fluorescence Decay_Decay Pre-Processing:Use Periodicity" {
        n353 = case shown="True" w1767 {
          tunnel: w1766 -> [w1775 w1779]
          tunnel: w1765 -> [w1774 w1782]
          tunnel: [w1773 w1781] -> w1764
          tunnel: w1763 -> [w1772 w1780]
          tunnel: [w1771 w1777] -> w1762
          tunnel: "Use Periodicity" -> [w1770 w1783]
          tunnel: [w1768 w1776] -> w1761
          tunnel: w1760 -> [_ w1776]
          frame False {
            n354 = Get Variant Attribute(Variant=w1774, name=w1775, default value (empty Variant)=w1770, error in=w1772) -> (duplicate Variant=w1773:variant, value=w1769:bool, error out=w1771:errorcluster)  [unwired: 1 out]
            n355 = To Variant(anything=w1769) -> (Variant=w1768:variant)
          }
          frame True {
            n356 = Variant To Data(type=w1783, Variant=w1776) -> (data=w1778:bool)  [unwired: 1 in, 1 out]
            n357 = Set Variant Attribute(Variant=w1782, name=w1779, value=w1778, error in=w1780) -> (Variant out=w1781:variant, error out=w1777:errorcluster)  [unwired: 1 out]
          }
        }
      }
      frame "Fluorescence Decay_Decay Pre-Processing:Use Cursors" {
        n358 = case shown="True" w1792 {
          tunnel: w1791 -> [w1800 w1804]
          tunnel: w1790 -> [w1799 w1807]
          tunnel: [w1798 w1806] -> w1789
          tunnel: w1788 -> [w1797 w1805]
          tunnel: [w1796 w1802] -> w1787
          tunnel: "Use Cursors" -> [w1795 w1808]
          tunnel: [w1793 w1801] -> w1786
          tunnel: w1785 -> [_ w1801]
          frame False {
            n359 = Get Variant Attribute(Variant=w1799, name=w1800, default value (empty Variant)=w1795, error in=w1797) -> (duplicate Variant=w1798:variant, value=w1794:bool, error out=w1796:errorcluster)  [unwired: 1 out]
            n360 = To Variant(anything=w1794) -> (Variant=w1793:variant)
          }
          frame True {
            n361 = Variant To Data(type=w1808, Variant=w1801) -> (data=w1803:bool)  [unwired: 1 in, 1 out]
            n362 = Set Variant Attribute(Variant=w1807, name=w1804, value=w1803, error in=w1805) -> (Variant out=w1806:variant, error out=w1802:errorcluster)  [unwired: 1 out]
          }
        }
      }
      frame "Fluorescence Decay_Decay Pre-Processing:Tail Fraction" {
        n363 = case shown="True" w1817 {
          tunnel: w1816 -> [w1825 w1829]
          tunnel: w1815 -> [w1824 w1832]
          tunnel: [w1823 w1831] -> w1814
          tunnel: w1813 -> [w1822 w1830]
          tunnel: [w1821 w1827] -> w1812
          tunnel: "Tail Fraction" -> [w1820 w1833]
          tunnel: [w1818 w1826] -> w1811
          tunnel: w1810 -> [_ w1826]
          frame False {
            n364 = Get Variant Attribute(Variant=w1824, name=w1825, default value (empty Variant)=w1820, error in=w1822) -> (duplicate Variant=w1823:variant, value=w1819:dbl, error out=w1821:errorcluster)  [unwired: 1 out]
            n365 = To Variant(anything=w1819) -> (Variant=w1818:variant)
          }
          frame True {
            n366 = Variant To Data(type=w1833, Variant=w1826) -> (data=w1828:dbl)  [unwired: 1 in, 1 out]
            n367 = Set Variant Attribute(Variant=w1832, name=w1829, value=w1828, error in=w1830) -> (Variant out=w1831:variant, error out=w1827:errorcluster)  [unwired: 1 out]
          }
        }
      }
      frame "Fluorescence Decay_Decay Pre-Processing:Head Fraction" {
        n368 = case shown="True" w1842 {
          tunnel: w1841 -> [w1850 w1854]
          tunnel: w1840 -> [w1849 w1857]
          tunnel: [w1848 w1856] -> w1839
          tunnel: w1838 -> [w1847 w1855]
          tunnel: [w1846 w1852] -> w1837
          tunnel: "Head Fraction" -> [w1845 w1858]
          tunnel: [w1843 w1851] -> w1836
          tunnel: w1835 -> [_ w1851]
          frame False {
            n369 = Get Variant Attribute(Variant=w1849, name=w1850, default value (empty Variant)=w1845, error in=w1847) -> (duplicate Variant=w1848:variant, value=w1844:dbl, error out=w1846:errorcluster)  [unwired: 1 out]
            n370 = To Variant(anything=w1844) -> (Variant=w1843:variant)
          }
          frame True {
            n371 = Variant To Data(type=w1858, Variant=w1851) -> (data=w1853:dbl)  [unwired: 1 in, 1 out]
            n372 = Set Variant Attribute(Variant=w1857, name=w1854, value=w1853, error in=w1855) -> (Variant out=w1856:variant, error out=w1852:errorcluster)  [unwired: 1 out]
          }
        }
      }
      frame "Fluorescence Decay_Decay Pre-Processing:Additional Points" {
        n373 = case shown="True" w1867 {
          tunnel: w1866 -> [w1875 w1879]
          tunnel: w1865 -> [w1874 w1882]
          tunnel: [w1873 w1881] -> w1864
          tunnel: w1863 -> [w1872 w1880]
          tunnel: [w1871 w1877] -> w1862
          tunnel: "Additional Points" -> [w1870 w1883]
          tunnel: [w1868 w1876] -> w1861
          tunnel: w1860 -> [_ w1876]
          frame False {
            n374 = Get Variant Attribute(Variant=w1874, name=w1875, default value (empty Variant)=w1870, error in=w1872) -> (duplicate Variant=w1873:variant, value=w1869:u32, error out=w1871:errorcluster)  [unwired: 1 out]
            n375 = To Variant(anything=w1869) -> (Variant=w1868:variant)
          }
          frame True {
            n376 = Variant To Data(type=w1883, Variant=w1876) -> (data=w1878:u32)  [unwired: 1 in, 1 out]
            n377 = Set Variant Attribute(Variant=w1882, name=w1879, value=w1878, error in=w1880) -> (Variant out=w1881:variant, error out=w1877:errorcluster)  [unwired: 1 out]
          }
        }
      }
      frame "Fluorescence Decay_Decay Pre-Processing:Straighten Decay" {
        n378 = case shown="True" w1892 {
          tunnel: w1891 -> [w1900 w1904]
          tunnel: w1890 -> [w1899 w1907]
          tunnel: [w1898 w1906] -> w1889
          tunnel: w1888 -> [w1897 w1905]
          tunnel: [w1896 w1902] -> w1887
          tunnel: "Straighten Decay" -> [w1895 w1908]
          tunnel: [w1893 w1901] -> w1886
          tunnel: w1885 -> [_ w1901]
          frame False {
            n379 = Get Variant Attribute(Variant=w1899, name=w1900, default value (empty Variant)=w1895, error in=w1897) -> (duplicate Variant=w1898:variant, value=w1894:bool, error out=w1896:errorcluster)  [unwired: 1 out]
            n380 = To Variant(anything=w1894) -> (Variant=w1893:variant)
          }
          frame True {
            n381 = Variant To Data(type=w1908, Variant=w1901) -> (data=w1903:bool)  [unwired: 1 in, 1 out]
            n382 = Set Variant Attribute(Variant=w1907, name=w1904, value=w1903, error in=w1905) -> (Variant out=w1906:variant, error out=w1902:errorcluster)  [unwired: 1 out]
          }
        }
      }
      frame "Fluorescence Decay_Decay Pre-Processing:Constant Background" {
        n383 = case shown="True" w1917 {
          tunnel: w1916 -> [w1925 w1929]
          tunnel: w1915 -> [w1924 w1932]
          tunnel: [w1923 w1931] -> w1914
          tunnel: w1913 -> [w1922 w1930]
          tunnel: [w1921 w1927] -> w1912
          tunnel: "Constant Background" -> [w1920 w1933]
          tunnel: [w1918 w1926] -> w1911
          tunnel: w1910 -> [_ w1926]
          frame False {
            n384 = Get Variant Attribute(Variant=w1924, name=w1925, default value (empty Variant)=w1920, error in=w1922) -> (duplicate Variant=w1923:variant, value=w1919:dbl, error out=w1921:errorcluster)  [unwired: 1 out]
            n385 = To Variant(anything=w1919) -> (Variant=w1918:variant)
          }
          frame True {
            n386 = Variant To Data(type=w1933, Variant=w1926) -> (data=w1928:dbl)  [unwired: 1 in, 1 out]
            n387 = Set Variant Attribute(Variant=w1932, name=w1929, value=w1928, error in=w1930) -> (Variant out=w1931:variant, error out=w1927:errorcluster)  [unwired: 1 out]
          }
        }
      }
      frame "Fluorescence Decay_Decay Pre-Processing:Pixel-Normalize Decay" {
        n388 = case shown="True" w1942 {
          tunnel: w1941 -> [w1950 w1954]
          tunnel: w1940 -> [w1949 w1957]
          tunnel: [w1948 w1956] -> w1939
          tunnel: w1938 -> [w1947 w1955]
          tunnel: [w1946 w1952] -> w1937
          tunnel: "Pixel-Normalize Decay" -> [w1945 w1958]
          tunnel: [w1943 w1951] -> w1936
          tunnel: w1935 -> [_ w1951]
          frame False {
            n389 = Get Variant Attribute(Variant=w1949, name=w1950, default value (empty Variant)=w1945, error in=w1947) -> (duplicate Variant=w1948:variant, value=w1944:bool, error out=w1946:errorcluster)  [unwired: 1 out]
            n390 = To Variant(anything=w1944) -> (Variant=w1943:variant)
          }
          frame True {
            n391 = Variant To Data(type=w1958, Variant=w1951) -> (data=w1953:bool)  [unwired: 1 in, 1 out]
            n392 = Set Variant Attribute(Variant=w1957, name=w1954, value=w1953, error in=w1955) -> (Variant out=w1956:variant, error out=w1952:errorcluster)  [unwired: 1 out]
          }
        }
      }
      frame "Fluorescence Decay_Advanced Analysis:Extract IRF instead of Decay" {
        n393 = case shown="True" w1967 {
          tunnel: w1966 -> [w1975 w1979]
          tunnel: w1965 -> [w1974 w1982]
          tunnel: [w1973 w1981] -> w1964
          tunnel: w1963 -> [w1972 w1980]
          tunnel: [w1971 w1977] -> w1962
          tunnel: "Extract IRF instead of Decay" -> [w1970 w1983]
          tunnel: [w1968 w1976] -> w1961
          tunnel: w1960 -> [_ w1976]
          frame False {
            n394 = Get Variant Attribute(Variant=w1974, name=w1975, default value (empty Variant)=w1970, error in=w1972) -> (duplicate Variant=w1973:variant, value=w1969:bool, error out=w1971:errorcluster)  [unwired: 1 out]
            n395 = To Variant(anything=w1969) -> (Variant=w1968:variant)
          }
          frame True {
            n396 = Variant To Data(type=w1983, Variant=w1976) -> (data=w1978:bool)  [unwired: 1 in, 1 out]
            n397 = Set Variant Attribute(Variant=w1982, name=w1979, value=w1978, error in=w1980) -> (Variant out=w1981:variant, error out=w1977:errorcluster)  [unwired: 1 out]
          }
        }
      }
      frame "Fluorescence Decay_Advanced Analysis:IRF Extraction Options" {
        n398 = case shown="True" w1992 {
          tunnel: w1991 -> [w2000 w2004]
          tunnel: w1990 -> [w1999 w2007]
          tunnel: [w1998 w2006] -> w1989
          tunnel: w1988 -> [w1997 w2005]
          tunnel: [w1996 w2002] -> w1987
          tunnel: "Time Constant for IRF Extraction" -> [w1995 w2008]
          tunnel: [w1993 w2001] -> w1986
          tunnel: w1985 -> [_ w2001]
          frame False {
            n399 = Get Variant Attribute(Variant=w1999, name=w2000, default value (empty Variant)=w1995, error in=w1997) -> (duplicate Variant=w1998:variant, value=w1994:T26, error out=w1996:errorcluster)  [unwired: 1 out]
            n400 = To Variant(anything=w1994) -> (Variant=w1993:variant)
          }
          frame True {
            n401 = Variant To Data(type=w2008, Variant=w2001) -> (data=w2003:T26)  [unwired: 1 in, 1 out]
            n402 = Set Variant Attribute(Variant=w2007, name=w2004, value=w2003, error in=w2005) -> (Variant out=w2006:variant, error out=w2002:errorcluster)  [unwired: 1 out]
          }
        }
      }
      frame "Fluorescence Decay_Advanced Analysis:IRF Optimization Options" {
        n403 = case shown="True" w2017 {
          tunnel: w2016 -> [w2025 w2029]
          tunnel: w2015 -> [w2024 w2032]
          tunnel: [w2023 w2031] -> w2014
          tunnel: w2013 -> [w2022 w2030]
          tunnel: [w2021 w2027] -> w2012
          tunnel: "IRF Optimization Options" -> [w2020 w2033]
          tunnel: [w2018 w2026] -> w2011
          tunnel: w2010 -> [_ w2026]
          frame False {
            n404 = Get Variant Attribute(Variant=w2024, name=w2025, default value (empty Variant)=w2020, error in=w2022) -> (duplicate Variant=w2023:variant, value=w2019:T30, error out=w2021:errorcluster)  [unwired: 1 out]
            n405 = To Variant(anything=w2019) -> (Variant=w2018:variant)
          }
          frame True {
            n406 = Variant To Data(type=w2033, Variant=w2026) -> (data=w2028:T30)  [unwired: 1 in, 1 out]
            n407 = Set Variant Attribute(Variant=w2032, name=w2029, value=w2028, error in=w2030) -> (Variant out=w2031:variant, error out=w2027:errorcluster)  [unwired: 1 out]
          }
        }
      }
      frame "Fluorescence Decay_Advanced Analysis:Square Pulse Options" {
        n408 = case shown="True" w2042 {
          tunnel: w2041 -> [w2050 w2054]
          tunnel: w2040 -> [w2049 w2057]
          tunnel: [w2048 w2056] -> w2039
          tunnel: w2038 -> [w2047 w2055]
          tunnel: [w2046 w2052] -> w2037
          tunnel: "Square Pulse Options" -> [w2045 w2058]
          tunnel: [w2043 w2051] -> w2036
          tunnel: w2035 -> [_ w2051]
          frame False {
            n409 = Get Variant Attribute(Variant=w2049, name=w2050, default value (empty Variant)=w2045, error in=w2047) -> (duplicate Variant=w2048:variant, value=w2044:T23, error out=w2046:errorcluster)  [unwired: 1 out]
            n410 = To Variant(anything=w2044) -> (Variant=w2043:variant)
          }
          frame True {
            n411 = Variant To Data(type=w2058, Variant=w2051) -> (data=w2053:T23)  [unwired: 1 in, 1 out]
            n412 = Set Variant Attribute(Variant=w2057, name=w2054, value=w2053, error in=w2055) -> (Variant out=w2056:variant, error out=w2052:errorcluster)  [unwired: 1 out]
          }
        }
      }
      frame "Fluorescence Decay_Advanced Analysis:IRF Order" {
        n413 = case shown="True" w2067 {
          tunnel: w2066 -> [w2075 w2079]
          tunnel: w2065 -> [w2074 w2082]
          tunnel: [w2073 w2081] -> w2064
          tunnel: w2063 -> [w2072 w2080]
          tunnel: [w2071 w2077] -> w2062
          tunnel: "IRF order" -> [w2070 w2083]
          tunnel: [w2068 w2076] -> w2061
          tunnel: w2060 -> [_ w2076]
          frame False {
            n414 = Get Variant Attribute(Variant=w2074, name=w2075, default value (empty Variant)=w2070, error in=w2072) -> (duplicate Variant=w2073:variant, value=w2069:i32, error out=w2071:errorcluster)  [unwired: 1 out]
            n415 = To Variant(anything=w2069) -> (Variant=w2068:variant)
          }
          frame True {
            n416 = Variant To Data(type=w2083, Variant=w2076) -> (data=w2078:i32)  [unwired: 1 in, 1 out]
            n417 = Set Variant Attribute(Variant=w2082, name=w2079, value=w2078, error in=w2080) -> (Variant out=w2081:variant, error out=w2077:errorcluster)  [unwired: 1 out]
          }
        }
      }
      frame "Fluorescence Decay_Advanced Analysis:IRF Time Constants" {
        n418 = case shown="True" w2092 {
          tunnel: w2091 -> [w2101 w2106]
          tunnel: w2090 -> [w2100 w2109]
          tunnel: [w2099 w2108] -> w2089
          tunnel: w2088 -> [w2098 w2107]
          tunnel: [w2097 w2104] -> w2087
          tunnel: "IRF Time Constants" -> [w2096 w2110]
          tunnel: [w2094 w2103] -> w2086
          tunnel: w2085 -> [_ w2103]
          tunnel: [w2093 w2102] -> _
          frame False {
            n419 = Get Variant Attribute(Variant=w2100, name=w2101, default value (empty Variant)=w2096, error in=w2098) -> (duplicate Variant=w2099:variant, found=w2093:bool, value=w2095:dbl[], error out=w2097:errorcluster)
            n420 = To Variant(anything=w2095) -> (Variant=w2094:variant)
          }
          frame True {
            n421 = Variant To Data(type=w2110, Variant=w2103) -> (data=w2105:dbl[])  [unwired: 1 in, 1 out]
            n422 = Set Variant Attribute(Variant=w2109, name=w2106, value=w2105, error in=w2107) -> (Variant out=w2108:variant, replaced=w2102:bool, error out=w2104:errorcluster)
          }
        }
      }
      frame "Fluorescence Decay_Advanced Analysis:Wavelet Analysis Options" {
        n423 = case shown="True" w2119 {
          tunnel: w2118 -> [w2127 w2131]
          tunnel: w2117 -> [w2126 w2134]
          tunnel: [w2125 w2133] -> w2116
          tunnel: w2115 -> [w2124 w2132]
          tunnel: [w2123 w2129] -> w2114
          tunnel: "Wavelet Analysis Options" -> [w2122 w2135]
          tunnel: [w2120 w2128] -> w2113
          tunnel: w2112 -> [_ w2128]
          frame False {
            n424 = Get Variant Attribute(Variant=w2126, name=w2127, default value (empty Variant)=w2122, error in=w2124) -> (duplicate Variant=w2125:variant, value=w2121:T25, error out=w2123:errorcluster)  [unwired: 1 out]
            n425 = To Variant(anything=w2121) -> (Variant=w2120:variant)
          }
          frame True {
            n426 = Variant To Data(type=w2135, Variant=w2128) -> (data=w2130:T25)  [unwired: 1 in, 1 out]
            n427 = Set Variant Attribute(Variant=w2134, name=w2131, value=w2130, error in=w2132) -> (Variant out=w2133:variant, error out=w2129:errorcluster)  [unwired: 1 out]
          }
        }
      }
      frame "Fluorescence Decay_Advanced Analysis:Average Lifetime Options" {
        n428 = case shown="True" w2144 {
          tunnel: w2143 -> [w2152 w2156]
          tunnel: w2142 -> [w2151 w2159]
          tunnel: [w2150 w2158] -> w2141
          tunnel: w2140 -> [w2149 w2157]
          tunnel: [w2148 w2154] -> w2139
          tunnel: "Average Lifetime Options" -> [w2147 w2160]
          tunnel: [w2145 w2153] -> w2138
          tunnel: w2137 -> [_ w2153]
          frame False {
            n429 = Get Variant Attribute(Variant=w2151, name=w2152, default value (empty Variant)=w2147, error in=w2149) -> (duplicate Variant=w2150:variant, value=w2146:T22, error out=w2148:errorcluster)  [unwired: 1 out]
            n430 = To Variant(anything=w2146) -> (Variant=w2145:variant)
          }
          frame True {
            n431 = Variant To Data(type=w2160, Variant=w2153) -> (data=w2155:T22)  [unwired: 1 in, 1 out]
            n432 = Set Variant Attribute(Variant=w2159, name=w2156, value=w2155, error in=w2157) -> (Variant out=w2158:variant, error out=w2154:errorcluster)  [unwired: 1 out]
          }
        }
      }
      frame "Fluorescence Decay_Fit Options:Fit Options" {
        n433 = case shown="False" w2169 {
          tunnel: w2168 -> [w2172 w2220]
          tunnel: w2167 -> [w2179 w2223]
          tunnel: [w2170 w2222] -> w2166
          tunnel: w2165 -> [w2178 w2221]
          tunnel: [w2171 w2218] -> w2164
          tunnel: "Fit Options" -> [w2177 w2224]
          tunnel: [w2175 w2217] -> w2163
          tunnel: w2162 -> [_ w2217]
          frame False {
            n434 = Get Variant Attribute(Variant=w2179, name=w2172, default value (empty Variant)=w2177, error in=w2178) -> (duplicate Variant=w2173:variant, value=w2176:T32, error out=w2174:errorcluster)  [unwired: 1 out]
            n435 = case shown="Error .." w2174 {
              selector: w2174 -> [w2180 _]
              tunnel: w2176 -> [w2182 _]
              tunnel: [w2181 w2192] -> w2175
              tunnel: w2173 -> [w2183 w2189]
              tunnel: w2172 -> [_ w2185]
              tunnel: [w2180 w2191] -> w2171
              tunnel: [w2183 w2190] -> w2170
              frame No Error {
                n436 = To Variant(anything=w2182) -> (Variant=w2181:variant)
              }
              frame Error {
                n437 = Get Variant Attribute(Variant=w2189, name=w2185, default value (empty Variant)=T73 {"Show Fit Residuals"=TRUE, "Fit Model"=enum."1-Exponential", "Residual Type"=enum."Standard", "Max Decay Percentile"=0.0, "Min Decay Percentile"=0.0, "Show Full Decay"=TRUE, "Weights"=enum."Unweighted", "Fitting Method"=enum."Least Square", "Compute Parameter Uncertainties"=TRUE, "Periodic Boundaries"=TRUE, "Model Calculation"=enum."Simulation", "Period"=1.2500000000000001e-08, "Termination Criteria"={"Max Iterations"=0, "Max Function Calls"=0, "Max Time"=1000.0, "Function Tolerance"=1e-06, "Parameter Tolerance"=1e-06, "Gradient Tolerance"=0.0, "Min Lambda"=1e-06, "Max Lambda"=1e-06, "Initial Tick Count"=0}, "Offset Resolution"=1.2500000000000001e-08, "Use Local IRF"=TRUE, "Fitting Algorithm"=enum."Levenberg-Marquardt", "Show Confidence Interval "=TRUE, "Confidence Level"=95.0} ("Decay Fit Options")) -> (duplicate Variant=w2188:variant, value=w2187:T73, error out=w2184:errorcluster)  [unwired: 1 in, 1 out]
                n438 = case shown="Error .." w2184 {
                  selector: w2184 -> [w2194 _]
                  tunnel: w2187 -> [w2196 _]
                  tunnel: [w2195 w2202] -> w2192
                  tunnel: w2188 -> [w2193 w2205]
                  tunnel: w2185 -> [_ w2197]
                  tunnel: [w2194 w2198] -> w2191
                  tunnel: [w2193 w2199] -> w2190
                  frame No Error {
                    n439 = To Variant(anything=w2196) -> (Variant=w2195:variant)
                  }
                  frame Error {
                    n440 = Get Variant Attribute(Variant=w2205, name=w2197, default value (empty Variant)=T75 {"Show Fit Residuals"=TRUE, "Fit Model"=enum."1-Exponential", "Residual Type"=enum."Standard", "Max Decay Percentile"=0.0, "Min Decay Percentile"=0.0, "Show Full Decay"=TRUE, "Weights"=enum."Unweighted", "Fitting Method"=enum."Least Square", "Compute Parameter Uncertainties"=TRUE, "Periodic Boundaries"=TRUE, "Model Calculation"=enum."Simulation", "Period"=1.2500000000000001e-08, "Termination Criteria"={"Max Iterations"=0, "Max Function Calls"=0, "Max Time"=1000.0, "Function Tolerance"=1e-06, "Parameter Tolerance"=1e-06, "Gradient Tolerance"=0.0, "Min Lambda"=1e-06, "Max Lambda"=1e-06, "Initial Tick Count"=0}, "Offset Resolution"=1.2500000000000001e-08, "Use Local IRF"=TRUE, "Fitting Algorithm"=enum."Levenberg-Marquardt"} ("Decay Fit Options")) -> (duplicate Variant=w2200:variant, value=w2203:T75, error out=w2201:errorcluster)  [unwired: 1 in, 1 out]
                    n441 = case shown="Error .." w2201 {
                      selector: w2201 -> [w2206 _]
                      tunnel: w2203 -> [w2209 _]
                      tunnel: [w2208 w2210] -> w2202
                      tunnel: w2200 -> [w2207 w2216]
                      tunnel: [w2207 w2212] -> w2199
                      tunnel: [w2206 w2213] -> w2198
                      tunnel: w2197 -> [_ w2215]
                      frame No Error {
                        n442 = To Variant(anything=w2209) -> (Variant=w2208:variant)
                      }
                      frame Error {
                        n443 = Get Variant Attribute(Variant=w2216, name=w2215, default value (empty Variant)=T76 {"Show Fit Residuals"=TRUE, "Fit Model"=enum."1-Exponential", "Residual Type"=enum."Standard", "Max Decay Percentile"=0.0, "Min Decay Percentile"=0.0, "Show Full Decay"=TRUE, "Weights"=enum."Unweighted", "Fitting Method"=enum."Least Square", "Compute Parameter Uncertainties"=TRUE, "Periodic Boundaries"=TRUE, "Model Calculation"=enum."Simulation", "Period"=1.2500000000000001e-08, "Termination Criteria"={"Max Iterations"=0, "Max Function Calls"=0, "Max Time"=1000.0, "Function Tolerance"=1e-06, "Parameter Tolerance"=1e-06, "Gradient Tolerance"=0.0, "Min Lambda"=1e-06, "Max Lambda"=1e-06, "Initial Tick Count"=0}, "Offset Resolution"=1.2500000000000001e-08, "Use Local IRF"=TRUE, "Fitting Algorithm"=enum."Levenberg-Marquardt"} ("Decay Fit Options")) -> (duplicate Variant=w2212:variant, value=w2211:T76, error out=w2213:errorcluster)  [unwired: 1 in, 1 out]
                        n444 = To Variant(anything=w2211) -> (Variant=w2210:variant)
                      }
                    }
                  }
                }
              }
            }
          }
          frame True {
            n445 = Variant To Data(type=w2224, Variant=w2217) -> (data=w2219:T32)  [unwired: 1 in, 1 out]
            n446 = Set Variant Attribute(Variant=w2223, name=w2220, value=w2219, error in=w2221) -> (Variant out=w2222:variant, error out=w2218:errorcluster)  [unwired: 1 out]
          }
        }
      }
      frame "Fluorescence Decay_Fit Options:Use Legacy Fitting Approach" {
        n447 = case shown="True" w2233 {
          tunnel: w2232 -> [w2241 w2245]
          tunnel: w2231 -> [w2240 w2248]
          tunnel: [w2239 w2247] -> w2230
          tunnel: w2229 -> [w2238 w2246]
          tunnel: [w2237 w2243] -> w2228
          tunnel: "Use Legagy Fitting Approach" -> [w2236 w2249]
          tunnel: [w2234 w2242] -> w2227
          tunnel: w2226 -> [_ w2242]
          frame False {
            n448 = Get Variant Attribute(Variant=w2240, name=w2241, default value (empty Variant)=w2236, error in=w2238) -> (duplicate Variant=w2239:variant, value=w2235:bool, error out=w2237:errorcluster)  [unwired: 1 out]
            n449 = To Variant(anything=w2235) -> (Variant=w2234:variant)
          }
          frame True {
            n450 = Variant To Data(type=w2249, Variant=w2242) -> (data=w2244:bool)  [unwired: 1 in, 1 out]
            n451 = Set Variant Attribute(Variant=w2248, name=w2245, value=w2244, error in=w2246) -> (Variant out=w2247:variant, error out=w2243:errorcluster)  [unwired: 1 out]
          }
        }
      }
      frame "Fluorescence Decay_Fit Options:Use Data Information Laser Period" {
        n452 = case shown="True" w2258 {
          tunnel: w2257 -> [w2266 w2270]
          tunnel: w2256 -> [w2265 w2273]
          tunnel: [w2264 w2272] -> w2255
          tunnel: w2254 -> [w2263 w2271]
          tunnel: [w2262 w2268] -> w2253
          tunnel: "Use Data Information Laser Period" -> [w2261 w2274]
          tunnel: [w2259 w2267] -> w2252
          tunnel: w2251 -> [_ w2267]
          frame False {
            n453 = Get Variant Attribute(Variant=w2265, name=w2266, default value (empty Variant)=w2261, error in=w2263) -> (duplicate Variant=w2264:variant, value=w2260:bool, error out=w2262:errorcluster)  [unwired: 1 out]
            n454 = To Variant(anything=w2260) -> (Variant=w2259:variant)
          }
          frame True {
            n455 = Variant To Data(type=w2274, Variant=w2267) -> (data=w2269:bool)  [unwired: 1 in, 1 out]
            n456 = Set Variant Attribute(Variant=w2273, name=w2270, value=w2269, error in=w2271) -> (Variant out=w2272:variant, error out=w2268:errorcluster)  [unwired: 1 out]
          }
        }
      }
      frame "Fluorescence Decay_Fit Parameters:Displayed Fit Parameters" {
        n457 = case shown="True" w2283 {
          tunnel: w2282 -> [w2291 w2295]
          tunnel: w2281 -> [w2290 w2298]
          tunnel: [w2289 w2297] -> w2280
          tunnel: w2279 -> [w2288 w2296]
          tunnel: [w2287 w2293] -> w2278
          tunnel: "Displayed Fit Parameters" -> [w2286 w2299]
          tunnel: [w2284 w2292] -> w2277
          tunnel: w2276 -> [_ w2292]
          frame False {
            n458 = Get Variant Attribute(Variant=w2290, name=w2291, default value (empty Variant)=w2286, error in=w2288) -> (duplicate Variant=w2289:variant, value=w2285:T44[], error out=w2287:errorcluster)  [unwired: 1 out]
            n459 = To Variant(anything=w2285) -> (Variant=w2284:variant)
          }
          frame True {
            n460 = Variant To Data(type=w2299, Variant=w2292) -> (data=w2294:T44[])  [unwired: 1 in, 1 out]
            n461 = Set Variant Attribute(Variant=w2298, name=w2295, value=w2294, error in=w2296) -> (Variant out=w2297:variant, error out=w2293:errorcluster)  [unwired: 1 out]
          }
        }
      }
      frame "Fluorescence Decay_Fit Parameters:Fit Parameter Constraints" {
        n462 = case shown="True" w2308 {
          tunnel: w2307 -> [w2316 w2320]
          tunnel: w2306 -> [w2315 w2323]
          tunnel: [w2314 w2322] -> w2305
          tunnel: w2304 -> [w2313 w2321]
          tunnel: [w2312 w2318] -> w2303
          tunnel: "Fit Parameter Constraints" -> [w2311 w2324]
          tunnel: [w2309 w2317] -> w2302
          tunnel: w2301 -> [_ w2317]
          frame False {
            n463 = Get Variant Attribute(Variant=w2315, name=w2316, default value (empty Variant)=w2311, error in=w2313) -> (duplicate Variant=w2314:variant, value=w2310:T43[], error out=w2312:errorcluster)  [unwired: 1 out]
            n464 = To Variant(anything=w2310) -> (Variant=w2309:variant)
          }
          frame True {
            n465 = Variant To Data(type=w2324, Variant=w2317) -> (data=w2319:T43[])  [unwired: 1 in, 1 out]
            n466 = Set Variant Attribute(Variant=w2323, name=w2320, value=w2319, error in=w2321) -> (Variant out=w2322:variant, error out=w2318:errorcluster)  [unwired: 1 out]
          }
        }
      }
      frame "Fluorescence Decay_Fit Parameters:Export Tabulated Results" {
        n467 = case shown="True" w2333 {
          tunnel: w2332 -> [w2341 w2345]
          tunnel: w2331 -> [w2340 w2348]
          tunnel: [w2339 w2347] -> w2330
          tunnel: w2329 -> [w2338 w2346]
          tunnel: [w2337 w2343] -> w2328
          tunnel: "Export Tabulated Results" -> [w2336 w2349]
          tunnel: [w2334 w2342] -> w2327
          tunnel: w2326 -> [_ w2342]
          frame False {
            n468 = Get Variant Attribute(Variant=w2340, name=w2341, default value (empty Variant)=w2336, error in=w2338) -> (duplicate Variant=w2339:variant, value=w2335:bool, error out=w2337:errorcluster)  [unwired: 1 out]
            n469 = To Variant(anything=w2335) -> (Variant=w2334:variant)
          }
          frame True {
            n470 = Variant To Data(type=w2349, Variant=w2342) -> (data=w2344:bool)  [unwired: 1 in, 1 out]
            n471 = Set Variant Attribute(Variant=w2348, name=w2345, value=w2344, error in=w2346) -> (Variant out=w2347:variant, error out=w2343:errorcluster)  [unwired: 1 out]
          }
        }
      }
      frame "Fluorescence Decay_Fit Parameters:MLE Baseline Offset Type" {
        n472 = case shown="True" w2358 {
          tunnel: w2357 -> [w2366 w2370]
          tunnel: w2356 -> [w2365 w2373]
          tunnel: [w2364 w2372] -> w2355
          tunnel: w2354 -> [w2363 w2371]
          tunnel: [w2362 w2368] -> w2353
          tunnel: "MLE Baseline Offset Type" -> [w2361 w2374]
          tunnel: [w2359 w2367] -> w2352
          tunnel: w2351 -> [_ w2367]
          frame False {
            n473 = Get Variant Attribute(Variant=w2365, name=w2366, default value (empty Variant)=w2361, error in=w2363) -> (duplicate Variant=w2364:variant, value=w2360:T40, error out=w2362:errorcluster)  [unwired: 1 out]
            n474 = To Variant(anything=w2360) -> (Variant=w2359:variant)
          }
          frame True {
            n475 = Variant To Data(type=w2374, Variant=w2367) -> (data=w2369:T40)  [unwired: 1 in, 1 out]
            n476 = Set Variant Attribute(Variant=w2373, name=w2370, value=w2369, error in=w2371) -> (Variant out=w2372:variant, error out=w2368:errorcluster)  [unwired: 1 out]
          }
        }
      }
      frame "Fluorescence Decay_Fit Parameters:MLE Baseline Offset" {
        n477 = case shown="True" w2383 {
          tunnel: w2382 -> [w2391 w2395]
          tunnel: w2381 -> [w2390 w2398]
          tunnel: [w2389 w2397] -> w2380
          tunnel: w2379 -> [w2388 w2396]
          tunnel: [w2387 w2393] -> w2378
          tunnel: "MLE Baseline Offset" -> [w2386 w2399]
          tunnel: [w2384 w2392] -> w2377
          tunnel: w2376 -> [_ w2392]
          frame False {
            n478 = Get Variant Attribute(Variant=w2390, name=w2391, default value (empty Variant)=w2386, error in=w2388) -> (duplicate Variant=w2389:variant, value=w2385:dbl, error out=w2387:errorcluster)  [unwired: 1 out]
            n479 = To Variant(anything=w2385) -> (Variant=w2384:variant)
          }
          frame True {
            n480 = Variant To Data(type=w2399, Variant=w2392) -> (data=w2394:dbl)  [unwired: 1 in, 1 out]
            n481 = Set Variant Attribute(Variant=w2398, name=w2395, value=w2394, error in=w2396) -> (Variant out=w2397:variant, error out=w2393:errorcluster)  [unwired: 1 out]
          }
        }
      }
      frame "Fluorescence Decay_Fit Parameters:Guess Parameter Names" {
        n482 = case shown="True" w2408 {
          tunnel: w2407 -> [w2416 w2420]
          tunnel: w2406 -> [w2415 w2423]
          tunnel: [w2414 w2422] -> w2405
          tunnel: w2404 -> [w2413 w2421]
          tunnel: [w2412 w2418] -> w2403
          tunnel: "Guess Parameters Names" -> [w2411 w2424]
          tunnel: [w2409 w2417] -> w2402
          tunnel: w2401 -> [_ w2417]
          frame False {
            n483 = Get Variant Attribute(Variant=w2415, name=w2416, default value (empty Variant)=w2411, error in=w2413) -> (duplicate Variant=w2414:variant, value=w2410:T42[], error out=w2412:errorcluster)  [unwired: 1 out]
            n484 = To Variant(anything=w2410) -> (Variant=w2409:variant)
          }
          frame True {
            n485 = Variant To Data(type=w2424, Variant=w2417) -> (data=w2419:T42[])  [unwired: 1 in, 1 out]
            n486 = Set Variant Attribute(Variant=w2423, name=w2420, value=w2419, error in=w2421) -> (Variant out=w2422:variant, error out=w2418:errorcluster)  [unwired: 1 out]
          }
        }
      }
      frame "Fluorescence Decay_Fit Parameters:Guess Parameter Values" {
        n487 = case shown="True" w2433 {
          tunnel: w2432 -> [w2441 w2445]
          tunnel: w2431 -> [w2440 w2448]
          tunnel: [w2439 w2447] -> w2430
          tunnel: w2429 -> [w2438 w2446]
          tunnel: [w2437 w2443] -> w2428
          tunnel: "Guess Parameter Values" -> [w2436 w2449]
          tunnel: [w2434 w2442] -> w2427
          tunnel: w2426 -> [_ w2442]
          frame False {
            n488 = Get Variant Attribute(Variant=w2440, name=w2441, default value (empty Variant)=w2436, error in=w2438) -> (duplicate Variant=w2439:variant, value=w2435:dbl[], error out=w2437:errorcluster)  [unwired: 1 out]
            n489 = To Variant(anything=w2435) -> (Variant=w2434:variant)
          }
          frame True {
            n490 = Variant To Data(type=w2449, Variant=w2442) -> (data=w2444:dbl[])  [unwired: 1 in, 1 out]
            n491 = Set Variant Attribute(Variant=w2448, name=w2445, value=w2444, error in=w2446) -> (Variant out=w2447:variant, error out=w2443:errorcluster)  [unwired: 1 out]
          }
        }
      }
      frame "Fluorescence Decay_Fit Parameters:Guess Parameters Options" {
        n492 = case shown="True" w2458 {
          tunnel: w2457 -> [w2466 w2470]
          tunnel: w2456 -> [w2465 w2473]
          tunnel: [w2464 w2472] -> w2455
          tunnel: w2454 -> [w2463 w2471]
          tunnel: [w2462 w2468] -> w2453
          tunnel: "Guess Parameters Options" -> [w2461 w2474]
          tunnel: [w2459 w2467] -> w2452
          tunnel: w2451 -> [_ w2467]
          frame False {
            n493 = Get Variant Attribute(Variant=w2465, name=w2466, default value (empty Variant)=w2461, error in=w2463) -> (duplicate Variant=w2464:variant, value=w2460:T41, error out=w2462:errorcluster)  [unwired: 1 out]
            n494 = To Variant(anything=w2460) -> (Variant=w2459:variant)
          }
          frame True {
            n495 = Variant To Data(type=w2474, Variant=w2467) -> (data=w2469:T41)  [unwired: 1 in, 1 out]
            n496 = Set Variant Attribute(Variant=w2473, name=w2470, value=w2469, error in=w2471) -> (Variant out=w2472:variant, error out=w2468:errorcluster)  [unwired: 1 out]
          }
        }
      }
      frame "Fluorescence Decay_Fit Parameters:Optimal Offset Selection Criterion" {
        n497 = case shown="True" w2483 {
          tunnel: w2482 -> [w2491 w2495]
          tunnel: w2481 -> [w2490 w2498]
          tunnel: [w2489 w2497] -> w2480
          tunnel: w2479 -> [w2488 w2496]
          tunnel: [w2487 w2493] -> w2478
          tunnel: "Optimal Offset Selection Criterion" -> [w2486 w2499]
          tunnel: [w2484 w2492] -> w2477
          tunnel: w2476 -> [_ w2492]
          frame False {
            n498 = Get Variant Attribute(Variant=w2490, name=w2491, default value (empty Variant)=w2486, error in=w2488) -> (duplicate Variant=w2489:variant, value=w2485:T39, error out=w2487:errorcluster)  [unwired: 1 out]
            n499 = To Variant(anything=w2485) -> (Variant=w2484:variant)
          }
          frame True {
            n500 = Variant To Data(type=w2499, Variant=w2492) -> (data=w2494:T39)  [unwired: 1 in, 1 out]
            n501 = Set Variant Attribute(Variant=w2498, name=w2495, value=w2494, error in=w2496) -> (Variant out=w2497:variant, error out=w2493:errorcluster)  [unwired: 1 out]
          }
        }
      }
      frame "Fluorescence Decay_Styles:Show Last Decay Only" {
        n502 = case shown="True" w2508 {
          tunnel: w2507 -> [w2516 w2520]
          tunnel: w2506 -> [w2515 w2523]
          tunnel: [w2514 w2522] -> w2505
          tunnel: w2504 -> [w2513 w2521]
          tunnel: [w2512 w2518] -> w2503
          tunnel: "Show Last Decay only" -> [w2511 w2524]
          tunnel: [w2509 w2517] -> w2502
          tunnel: w2501 -> [_ w2517]
          frame False {
            n503 = Get Variant Attribute(Variant=w2515, name=w2516, default value (empty Variant)=w2511, error in=w2513) -> (duplicate Variant=w2514:variant, value=w2510:bool, error out=w2512:errorcluster)  [unwired: 1 out]
            n504 = To Variant(anything=w2510) -> (Variant=w2509:variant)
          }
          frame True {
            n505 = Variant To Data(type=w2524, Variant=w2517) -> (data=w2519:bool)  [unwired: 1 in, 1 out]
            n506 = Set Variant Attribute(Variant=w2523, name=w2520, value=w2519, error in=w2521) -> (Variant out=w2522:variant, error out=w2518:errorcluster)  [unwired: 1 out]
          }
        }
      }
      frame "Fluorescence Decay_Styles:Decay Graph Color Array" {
        n507 = case shown="True" w2533 {
          tunnel: w2532 -> [w2541 w2545]
          tunnel: w2531 -> [w2540 w2548]
          tunnel: [w2539 w2547] -> w2530
          tunnel: w2529 -> [w2538 w2546]
          tunnel: [w2537 w2543] -> w2528
          tunnel: "Decay Graph Color Array" -> [w2536 w2549]
          tunnel: [w2534 w2542] -> w2527
          tunnel: w2526 -> [_ w2542]
          frame False {
            n508 = Get Variant Attribute(Variant=w2540, name=w2541, default value (empty Variant)=w2536, error in=w2538) -> (duplicate Variant=w2539:variant, value=w2535:u32[], error out=w2537:errorcluster)  [unwired: 1 out]
            n509 = To Variant(anything=w2535) -> (Variant=w2534:variant)
          }
          frame True {
            n510 = Variant To Data(type=w2549, Variant=w2542) -> (data=w2544:u32[])  [unwired: 1 in, 1 out]
            n511 = Set Variant Attribute(Variant=w2548, name=w2545, value=w2544, error in=w2546) -> (Variant out=w2547:variant, error out=w2543:errorcluster)  [unwired: 1 out]
          }
        }
      }
      frame "Fluorescence Decay:Decay Graph Active" {
        w2550 = FALSE  # Not a Settings Window Control
        n512 = case shown="True" w2558 {
          tunnel: w2557 -> [w2566 w2570]
          tunnel: w2556 -> [w2565 w2573]
          tunnel: [w2564 w2572] -> w2555
          tunnel: w2554 -> [w2563 w2571]
          tunnel: [w2562 w2568] -> w2553
          tunnel: w2550 -> [w2561 w2574]
          tunnel: [w2559 w2567] -> w2552
          tunnel: w2551 -> [_ w2567]
          frame False {
            n513 = Get Variant Attribute(Variant=w2565, name=w2566, default value (empty Variant)=w2561, error in=w2563) -> (duplicate Variant=w2564:variant, value=w2560:bool, error out=w2562:errorcluster)  [unwired: 1 out]
            n514 = To Variant(anything=w2560) -> (Variant=w2559:variant)
          }
          frame True {
            n515 = Variant To Data(type=w2574, Variant=w2567) -> (data=w2569:bool)  [unwired: 1 in, 1 out]
            n516 = Set Variant Attribute(Variant=w2573, name=w2570, value=w2569, error in=w2571) -> (Variant out=w2572:variant, error out=w2568:errorcluster)  [unwired: 1 out]
          }
        }
      }
      frame "Fluorescence Decay Statistics:Min Peak Value" {
        n517 = case shown="True" w2583 {
          tunnel: w2582 -> [w2591 w2595]
          tunnel: w2581 -> [w2590 w2598]
          tunnel: [w2589 w2597] -> w2580
          tunnel: w2579 -> [w2588 w2596]
          tunnel: [w2587 w2593] -> w2578
          tunnel: "Min Peak Value" -> [w2586 w2599]
          tunnel: [w2584 w2592] -> w2577
          tunnel: w2576 -> [_ w2592]
          frame False {
            n518 = Get Variant Attribute(Variant=w2590, name=w2591, default value (empty Variant)=w2586, error in=w2588) -> (duplicate Variant=w2589:variant, value=w2585:dbl, error out=w2587:errorcluster)  [unwired: 1 out]
            n519 = To Variant(anything=w2585) -> (Variant=w2584:variant)
          }
          frame True {
            n520 = Variant To Data(type=w2599, Variant=w2592) -> (data=w2594:dbl)  [unwired: 1 in, 1 out]
            n521 = Set Variant Attribute(Variant=w2598, name=w2595, value=w2594, error in=w2596) -> (Variant out=w2597:variant, error out=w2593:errorcluster)  [unwired: 1 out]
          }
        }
      }
      frame "Fluorescence Decay Statistics:Reject Low Decay Peak Pixels" {
        n522 = case shown="True" w2608 {
          tunnel: w2607 -> [w2616 w2620]
          tunnel: w2606 -> [w2615 w2623]
          tunnel: [w2614 w2622] -> w2605
          tunnel: w2604 -> [w2613 w2621]
          tunnel: [w2612 w2618] -> w2603
          tunnel: "Reject Low Decay Peak Pixels" -> [w2611 w2624]
          tunnel: [w2609 w2617] -> w2602
          tunnel: w2601 -> [_ w2617]
          frame False {
            n523 = Get Variant Attribute(Variant=w2615, name=w2616, default value (empty Variant)=w2611, error in=w2613) -> (duplicate Variant=w2614:variant, value=w2610:bool, error out=w2612:errorcluster)  [unwired: 1 out]
            n524 = To Variant(anything=w2610) -> (Variant=w2609:variant)
          }
          frame True {
            n525 = Variant To Data(type=w2624, Variant=w2617) -> (data=w2619:bool)  [unwired: 1 in, 1 out]
            n526 = Set Variant Attribute(Variant=w2623, name=w2620, value=w2619, error in=w2621) -> (Variant out=w2622:variant, error out=w2618:errorcluster)  [unwired: 1 out]
          }
        }
      }
      frame "Fluorescence Decay Statistics:Reject High Decay Peak Pixels" {
        n527 = case shown="True" w2633 {
          tunnel: w2632 -> [w2641 w2645]
          tunnel: w2631 -> [w2640 w2648]
          tunnel: [w2639 w2647] -> w2630
          tunnel: w2629 -> [w2638 w2646]
          tunnel: [w2637 w2643] -> w2628
          tunnel: "Reject High Decay Peak Pixels" -> [w2636 w2649]
          tunnel: [w2634 w2642] -> w2627
          tunnel: w2626 -> [_ w2642]
          frame False {
            n528 = Get Variant Attribute(Variant=w2640, name=w2641, default value (empty Variant)=w2636, error in=w2638) -> (duplicate Variant=w2639:variant, value=w2635:bool, error out=w2637:errorcluster)  [unwired: 1 out]
            n529 = To Variant(anything=w2635) -> (Variant=w2634:variant)
          }
          frame True {
            n530 = Variant To Data(type=w2649, Variant=w2642) -> (data=w2644:bool)  [unwired: 1 in, 1 out]
            n531 = Set Variant Attribute(Variant=w2648, name=w2645, value=w2644, error in=w2646) -> (Variant out=w2647:variant, error out=w2643:errorcluster)  [unwired: 1 out]
          }
        }
      }
      frame "Fluorescence Decay Statistics:Max Peak Value" {
        n532 = case shown="True" w2658 {
          tunnel: w2657 -> [w2666 w2670]
          tunnel: w2656 -> [w2665 w2673]
          tunnel: [w2664 w2672] -> w2655
          tunnel: w2654 -> [w2663 w2671]
          tunnel: [w2662 w2668] -> w2653
          tunnel: "Max Peak Value" -> [w2661 w2674]
          tunnel: [w2659 w2667] -> w2652
          tunnel: w2651 -> [_ w2667]
          frame False {
            n533 = Get Variant Attribute(Variant=w2665, name=w2666, default value (empty Variant)=w2661, error in=w2663) -> (duplicate Variant=w2664:variant, value=w2660:dbl, error out=w2662:errorcluster)  [unwired: 1 out]
            n534 = To Variant(anything=w2660) -> (Variant=w2659:variant)
          }
          frame True {
            n535 = Variant To Data(type=w2674, Variant=w2667) -> (data=w2669:dbl)  [unwired: 1 in, 1 out]
            n536 = Set Variant Attribute(Variant=w2673, name=w2670, value=w2669, error in=w2671) -> (Variant out=w2672:variant, error out=w2668:errorcluster)  [unwired: 1 out]
          }
        }
      }
      frame "Time Traces:Use File Timestamp" {
        n537 = case shown="True" w2683 {
          tunnel: w2682 -> [w2691 w2695]
          tunnel: w2681 -> [w2690 w2698]
          tunnel: [w2689 w2697] -> w2680
          tunnel: w2679 -> [w2688 w2696]
          tunnel: [w2687 w2693] -> w2678
          tunnel: "Use File Timestamp" -> [w2686 w2699]
          tunnel: [w2684 w2692] -> w2677
          tunnel: w2676 -> [_ w2692]
          frame False {
            n538 = Get Variant Attribute(Variant=w2690, name=w2691, default value (empty Variant)=w2686, error in=w2688) -> (duplicate Variant=w2689:variant, value=w2685:bool, error out=w2687:errorcluster)  [unwired: 1 out]
            n539 = To Variant(anything=w2685) -> (Variant=w2684:variant)
          }
          frame True {
            n540 = Variant To Data(type=w2699, Variant=w2692) -> (data=w2694:bool)  [unwired: 1 in, 1 out]
            n541 = Set Variant Attribute(Variant=w2698, name=w2695, value=w2694, error in=w2696) -> (Variant out=w2697:variant, error out=w2693:errorcluster)  [unwired: 1 out]
          }
        }
      }
      frame "Time Traces:Time Step" {
        n542 = case shown="True" w2708 {
          tunnel: w2707 -> [w2716 w2720]
          tunnel: w2706 -> [w2715 w2723]
          tunnel: [w2714 w2722] -> w2705
          tunnel: w2704 -> [w2713 w2721]
          tunnel: [w2712 w2718] -> w2703
          tunnel: "Time Step" -> [w2711 w2724]
          tunnel: [w2709 w2717] -> w2702
          tunnel: w2701 -> [_ w2717]
          frame False {
            n543 = Get Variant Attribute(Variant=w2715, name=w2716, default value (empty Variant)=w2711, error in=w2713) -> (duplicate Variant=w2714:variant, value=w2710:dbl[unit], error out=w2712:errorcluster)  [unwired: 1 out]
            n544 = To Variant(anything=w2710) -> (Variant=w2709:variant)
          }
          frame True {
            n545 = Variant To Data(type=w2724, Variant=w2717) -> (data=w2719:dbl[unit])  [unwired: 1 in, 1 out]
            n546 = Set Variant Attribute(Variant=w2723, name=w2720, value=w2719, error in=w2721) -> (Variant out=w2722:variant, error out=w2718:errorcluster)  [unwired: 1 out]
          }
        }
      }
      frame "Time Traces:Use Intensity Correction File" {
        n547 = case shown="True" w2733 {
          tunnel: w2732 -> [w2741 w2745]
          tunnel: w2731 -> [w2740 w2748]
          tunnel: [w2739 w2747] -> w2730
          tunnel: w2729 -> [w2738 w2746]
          tunnel: [w2737 w2743] -> w2728
          tunnel: "Use Intensity Correction File" -> [w2736 w2749]
          tunnel: [w2734 w2742] -> w2727
          tunnel: w2726 -> [_ w2742]
          frame False {
            n548 = Get Variant Attribute(Variant=w2740, name=w2741, default value (empty Variant)=w2736, error in=w2738) -> (duplicate Variant=w2739:variant, value=w2735:bool, error out=w2737:errorcluster)  [unwired: 1 out]
            n549 = To Variant(anything=w2735) -> (Variant=w2734:variant)
          }
          frame True {
            n550 = Variant To Data(type=w2749, Variant=w2742) -> (data=w2744:bool)  [unwired: 1 in, 1 out]
            n551 = Set Variant Attribute(Variant=w2748, name=w2745, value=w2744, error in=w2746) -> (Variant out=w2747:variant, error out=w2743:errorcluster)  [unwired: 1 out]
          }
        }
      }
      frame "Time Traces:Intensity Correction File" {
        n552 = case shown="True" w2758 {
          tunnel: w2757 -> [w2766 w2770]
          tunnel: w2756 -> [w2765 w2773]
          tunnel: [w2764 w2772] -> w2755
          tunnel: w2754 -> [w2763 w2771]
          tunnel: [w2762 w2768] -> w2753
          tunnel: "Intensity Correction File" -> [w2761 w2774]
          tunnel: [w2759 w2767] -> w2752
          tunnel: w2751 -> [_ w2767]
          frame False {
            n553 = Get Variant Attribute(Variant=w2765, name=w2766, default value (empty Variant)=w2761, error in=w2763) -> (duplicate Variant=w2764:variant, value=w2760:path, error out=w2762:errorcluster)  [unwired: 1 out]
            n554 = To Variant(anything=w2760) -> (Variant=w2759:variant)
          }
          frame True {
            n555 = Variant To Data(type=w2774, Variant=w2767) -> (data=w2769:path)  [unwired: 1 in, 1 out]
            n556 = Set Variant Attribute(Variant=w2773, name=w2770, value=w2769, error in=w2771) -> (Variant out=w2772:variant, error out=w2768:errorcluster)  [unwired: 1 out]
          }
        }
      }
      frame "Phasor Plot:Phasor Plot Smoothing Options" {
        n557 = case shown="True" w2783 {
          tunnel: w2782 -> [w2791 w2795]
          tunnel: w2781 -> [w2790 w2798]
          tunnel: [w2789 w2797] -> w2780
          tunnel: w2779 -> [w2788 w2796]
          tunnel: [w2787 w2793] -> w2778
          tunnel: "Phasor Plot Smoothing Options" -> [w2786 w2799]
          tunnel: [w2784 w2792] -> w2777
          tunnel: w2776 -> [_ w2792]
          frame False {
            n558 = Get Variant Attribute(Variant=w2790, name=w2791, default value (empty Variant)=w2786, error in=w2788) -> (duplicate Variant=w2789:variant, value=w2785:T47, error out=w2787:errorcluster)  [unwired: 1 out]
            n559 = To Variant(anything=w2785) -> (Variant=w2784:variant)
          }
          frame True {
            n560 = Variant To Data(type=w2799, Variant=w2792) -> (data=w2794:T47)  [unwired: 1 in, 1 out]
            n561 = Set Variant Attribute(Variant=w2798, name=w2795, value=w2794, error in=w2796) -> (Variant out=w2797:variant, error out=w2793:errorcluster)  [unwired: 1 out]
          }
        }
      }
      frame "Phasor Plot:Phasor Plot Size" {
        n562 = case shown="True" w2808 {
          tunnel: w2807 -> [w2816 w2820]
          tunnel: w2806 -> [w2815 w2823]
          tunnel: [w2814 w2822] -> w2805
          tunnel: w2804 -> [w2813 w2821]
          tunnel: [w2812 w2818] -> w2803
          tunnel: "Phasor Plot Size" -> [w2811 w2824]
          tunnel: [w2809 w2817] -> w2802
          tunnel: w2801 -> [_ w2817]
          frame False {
            n563 = Get Variant Attribute(Variant=w2815, name=w2816, default value (empty Variant)=w2811, error in=w2813) -> (duplicate Variant=w2814:variant, value=w2810:T50, error out=w2812:errorcluster)  [unwired: 1 out]
            n564 = To Variant(anything=w2810) -> (Variant=w2809:variant)
          }
          frame True {
            n565 = Variant To Data(type=w2824, Variant=w2817) -> (data=w2819:T50)  [unwired: 1 in, 1 out]
            n566 = Set Variant Attribute(Variant=w2823, name=w2820, value=w2819, error in=w2821) -> (Variant out=w2822:variant, error out=w2818:errorcluster)  [unwired: 1 out]
          }
        }
      }
      frame "Phasor Plot:Phasor Plot Graphics Options" {
        n567 = case shown="True" w2833 {
          tunnel: w2832 -> [w2841 w2845]
          tunnel: w2831 -> [w2840 w2848]
          tunnel: [w2839 w2847] -> w2830
          tunnel: w2829 -> [w2838 w2846]
          tunnel: [w2837 w2843] -> w2828
          tunnel: "Phasor Plot Graphics Options" -> [w2836 w2849]
          tunnel: [w2834 w2842] -> w2827
          tunnel: w2826 -> [_ w2842]
          frame False {
            n568 = Get Variant Attribute(Variant=w2840, name=w2841, default value (empty Variant)=w2836, error in=w2838) -> (duplicate Variant=w2839:variant, value=w2835:T46, error out=w2837:errorcluster)  [unwired: 1 out]
            n569 = To Variant(anything=w2835) -> (Variant=w2834:variant)
          }
          frame True {
            n570 = Variant To Data(type=w2849, Variant=w2842) -> (data=w2844:T46)  [unwired: 1 in, 1 out]
            n571 = Set Variant Attribute(Variant=w2848, name=w2845, value=w2844, error in=w2846) -> (Variant out=w2847:variant, error out=w2843:errorcluster)  [unwired: 1 out]
          }
        }
      }
      frame "Phasor Plot:Cumulative Phasor Plot" {
        n572 = case shown="True" w2858 {
          tunnel: w2857 -> [w2866 w2870]
          tunnel: w2856 -> [w2865 w2873]
          tunnel: [w2864 w2872] -> w2855
          tunnel: w2854 -> [w2863 w2871]
          tunnel: [w2862 w2868] -> w2853
          tunnel: "Cumulative Phasor Plot" -> [w2861 w2874]
          tunnel: [w2859 w2867] -> w2852
          tunnel: w2851 -> [_ w2867]
          frame False {
            n573 = Get Variant Attribute(Variant=w2865, name=w2866, default value (empty Variant)=w2861, error in=w2863) -> (duplicate Variant=w2864:variant, value=w2860:bool, error out=w2862:errorcluster)  [unwired: 1 out]
            n574 = To Variant(anything=w2860) -> (Variant=w2859:variant)
          }
          frame True {
            n575 = Variant To Data(type=w2874, Variant=w2867) -> (data=w2869:bool)  [unwired: 1 in, 1 out]
            n576 = Set Variant Attribute(Variant=w2873, name=w2870, value=w2869, error in=w2871) -> (Variant out=w2872:variant, error out=w2868:errorcluster)  [unwired: 1 out]
          }
        }
      }
      frame "Phasor Plot:Use Phasor Brightness" {
        n577 = case shown="True" w2883 {
          tunnel: w2882 -> [w2891 w2895]
          tunnel: w2881 -> [w2890 w2898]
          tunnel: [w2889 w2897] -> w2880
          tunnel: w2879 -> [w2888 w2896]
          tunnel: [w2887 w2893] -> w2878
          tunnel: "Use Phasor Brightness" -> [w2886 w2899]
          tunnel: [w2884 w2892] -> w2877
          tunnel: w2876 -> [_ w2892]
          frame False {
            n578 = Get Variant Attribute(Variant=w2890, name=w2891, default value (empty Variant)=w2886, error in=w2888) -> (duplicate Variant=w2889:variant, value=w2885:bool, error out=w2887:errorcluster)  [unwired: 1 out]
            n579 = To Variant(anything=w2885) -> (Variant=w2884:variant)
          }
          frame True {
            n580 = Variant To Data(type=w2899, Variant=w2892) -> (data=w2894:bool)  [unwired: 1 in, 1 out]
            n581 = Set Variant Attribute(Variant=w2898, name=w2895, value=w2894, error in=w2896) -> (Variant out=w2897:variant, error out=w2893:errorcluster)  [unwired: 1 out]
          }
        }
      }
      frame "Phasor Plot:Blend Overlay with Phasor Background" {
        n582 = case shown="True" w2908 {
          tunnel: w2907 -> [w2916 w2920]
          tunnel: w2906 -> [w2915 w2923]
          tunnel: [w2914 w2922] -> w2905
          tunnel: w2904 -> [w2913 w2921]
          tunnel: [w2912 w2918] -> w2903
          tunnel: "Blend Overlay with Phasor Background" -> [w2911 w2924]
          tunnel: [w2909 w2917] -> w2902
          tunnel: w2901 -> [_ w2917]
          frame False {
            n583 = Get Variant Attribute(Variant=w2915, name=w2916, default value (empty Variant)=w2911, error in=w2913) -> (duplicate Variant=w2914:variant, value=w2910:bool, error out=w2912:errorcluster)  [unwired: 1 out]
            n584 = To Variant(anything=w2910) -> (Variant=w2909:variant)
          }
          frame True {
            n585 = Variant To Data(type=w2924, Variant=w2917) -> (data=w2919:bool)  [unwired: 1 in, 1 out]
            n586 = Set Variant Attribute(Variant=w2923, name=w2920, value=w2919, error in=w2921) -> (Variant out=w2922:variant, error out=w2918:errorcluster)  [unwired: 1 out]
          }
        }
      }
      frame "Phasor Plot:Save Phasor Plot" {
        n587 = case shown="True" w2933 {
          tunnel: w2932 -> [w2941 w2945]
          tunnel: w2931 -> [w2940 w2948]
          tunnel: [w2939 w2947] -> w2930
          tunnel: w2929 -> [w2938 w2946]
          tunnel: [w2937 w2943] -> w2928
          tunnel: "Save Phasor Plot" -> [w2936 w2949]
          tunnel: [w2934 w2942] -> w2927
          tunnel: w2926 -> [_ w2942]
          frame False {
            n588 = Get Variant Attribute(Variant=w2940, name=w2941, default value (empty Variant)=w2936, error in=w2938) -> (duplicate Variant=w2939:variant, value=w2935:bool, error out=w2937:errorcluster)  [unwired: 1 out]
            n589 = To Variant(anything=w2935) -> (Variant=w2934:variant)
          }
          frame True {
            n590 = Variant To Data(type=w2949, Variant=w2942) -> (data=w2944:bool)  [unwired: 1 in, 1 out]
            n591 = Set Variant Attribute(Variant=w2948, name=w2945, value=w2944, error in=w2946) -> (Variant out=w2947:variant, error out=w2943:errorcluster)  [unwired: 1 out]
          }
        }
      }
      frame "Phasor Plot:Show References" {
        n592 = case shown="True" w2958 {
          tunnel: w2957 -> [w2966 w2970]
          tunnel: w2956 -> [w2965 w2973]
          tunnel: [w2964 w2972] -> w2955
          tunnel: w2954 -> [w2963 w2971]
          tunnel: [w2962 w2968] -> w2953
          tunnel: "Show References" -> [w2961 w2974]
          tunnel: [w2959 w2967] -> w2952
          tunnel: w2951 -> [_ w2967]
          frame False {
            n593 = Get Variant Attribute(Variant=w2965, name=w2966, default value (empty Variant)=w2961, error in=w2963) -> (duplicate Variant=w2964:variant, value=w2960:bool, error out=w2962:errorcluster)  [unwired: 1 out]
            n594 = To Variant(anything=w2960) -> (Variant=w2959:variant)
          }
          frame True {
            n595 = Variant To Data(type=w2974, Variant=w2967) -> (data=w2969:bool)  [unwired: 1 in, 1 out]
            n596 = Set Variant Attribute(Variant=w2973, name=w2970, value=w2969, error in=w2971) -> (Variant out=w2972:variant, error out=w2968:errorcluster)  [unwired: 1 out]
          }
        }
      }
      frame "Phasor Plot:Phasor Ratio Decay Range" {
        n597 = case shown="True" w2983 {
          tunnel: w2982 -> [w2991 w2995]
          tunnel: w2981 -> [w2990 w2998]
          tunnel: [w2989 w2997] -> w2980
          tunnel: w2979 -> [w2988 w2996]
          tunnel: [w2987 w2993] -> w2978
          tunnel: "Phasor Ratio Decay Range" -> [w2986 w2999]
          tunnel: [w2984 w2992] -> w2977
          tunnel: w2976 -> [_ w2992]
          frame False {
            n598 = Get Variant Attribute(Variant=w2990, name=w2991, default value (empty Variant)=w2986, error in=w2988) -> (duplicate Variant=w2989:variant, value=w2985:dbl, error out=w2987:errorcluster)  [unwired: 1 out]
            n599 = To Variant(anything=w2985) -> (Variant=w2984:variant)
          }
          frame True {
            n600 = Variant To Data(type=w2999, Variant=w2992) -> (data=w2994:dbl)  [unwired: 1 in, 1 out]
            n601 = Set Variant Attribute(Variant=w2998, name=w2995, value=w2994, error in=w2996) -> (Variant out=w2997:variant, error out=w2993:errorcluster)  [unwired: 1 out]
          }
        }
      }
      frame "Phasor Plot:Exponential Fading" {
        n602 = case shown="True" w3008 {
          tunnel: w3007 -> [w3016 w3020]
          tunnel: w3006 -> [w3015 w3023]
          tunnel: [w3014 w3022] -> w3005
          tunnel: w3004 -> [w3013 w3021]
          tunnel: [w3012 w3018] -> w3003
          tunnel: "Exponential Fading" -> [w3011 w3024]
          tunnel: [w3009 w3017] -> w3002
          tunnel: w3001 -> [_ w3017]
          frame False {
            n603 = Get Variant Attribute(Variant=w3015, name=w3016, default value (empty Variant)=w3011, error in=w3013) -> (duplicate Variant=w3014:variant, value=w3010:bool, error out=w3012:errorcluster)  [unwired: 1 out]
            n604 = To Variant(anything=w3010) -> (Variant=w3009:variant)
          }
          frame True {
            n605 = Variant To Data(type=w3024, Variant=w3017) -> (data=w3019:bool)  [unwired: 1 in, 1 out]
            n606 = Set Variant Attribute(Variant=w3023, name=w3020, value=w3019, error in=w3021) -> (Variant out=w3022:variant, error out=w3018:errorcluster)  [unwired: 1 out]
          }
        }
      }
      frame "Phasor Plot:Phasor Ratio Reference Colors" {
        n607 = case shown="True" w3033 {
          tunnel: w3032 -> [w3041 w3045]
          tunnel: w3031 -> [w3040 w3048]
          tunnel: [w3039 w3047] -> w3030
          tunnel: w3029 -> [w3038 w3046]
          tunnel: [w3037 w3043] -> w3028
          tunnel: "Phasor Ratio Reference Colors" -> [w3036 w3049]
          tunnel: [w3034 w3042] -> w3027
          tunnel: w3026 -> [_ w3042]
          frame False {
            n608 = Get Variant Attribute(Variant=w3040, name=w3041, default value (empty Variant)=w3036, error in=w3038) -> (duplicate Variant=w3039:variant, value=w3035:T49, error out=w3037:errorcluster)  [unwired: 1 out]
            n609 = To Variant(anything=w3035) -> (Variant=w3034:variant)
          }
          frame True {
            n610 = Variant To Data(type=w3049, Variant=w3042) -> (data=w3044:T49)  [unwired: 1 in, 1 out]
            n611 = Set Variant Attribute(Variant=w3048, name=w3045, value=w3044, error in=w3046) -> (Variant out=w3047:variant, error out=w3043:errorcluster)  [unwired: 1 out]
          }
        }
      }
      frame "Phasor Plot:Reference Radius" {
        n612 = case shown="True" w3058 {
          tunnel: w3057 -> [w3066 w3070]
          tunnel: w3056 -> [w3065 w3073]
          tunnel: [w3064 w3072] -> w3055
          tunnel: w3054 -> [w3063 w3071]
          tunnel: [w3062 w3068] -> w3053
          tunnel: "Reference Radius" -> [w3061 w3074]
          tunnel: [w3059 w3067] -> w3052
          tunnel: w3051 -> [_ w3067]
          frame False {
            n613 = Get Variant Attribute(Variant=w3065, name=w3066, default value (empty Variant)=w3061, error in=w3063) -> (duplicate Variant=w3064:variant, value=w3060:i32, error out=w3062:errorcluster)  [unwired: 1 out]
            n614 = To Variant(anything=w3060) -> (Variant=w3059:variant)
          }
          frame True {
            n615 = Variant To Data(type=w3074, Variant=w3067) -> (data=w3069:i32)  [unwired: 1 in, 1 out]
            n616 = Set Variant Attribute(Variant=w3073, name=w3070, value=w3069, error in=w3071) -> (Variant out=w3072:variant, error out=w3068:errorcluster)  [unwired: 1 out]
          }
        }
      }
      frame "Phasor Plot:Show Color Map Vertices" {
        n617 = case shown="True" w3083 {
          tunnel: w3082 -> [w3091 w3095]
          tunnel: w3081 -> [w3090 w3098]
          tunnel: [w3089 w3097] -> w3080
          tunnel: w3079 -> [w3088 w3096]
          tunnel: [w3087 w3093] -> w3078
          tunnel: "Show Color Map Vertices" -> [w3086 w3099]
          tunnel: [w3084 w3092] -> w3077
          tunnel: w3076 -> [_ w3092]
          frame False {
            n618 = Get Variant Attribute(Variant=w3090, name=w3091, default value (empty Variant)=w3086, error in=w3088) -> (duplicate Variant=w3089:variant, value=w3085:bool, error out=w3087:errorcluster)  [unwired: 1 out]
            n619 = To Variant(anything=w3085) -> (Variant=w3084:variant)
          }
          frame True {
            n620 = Variant To Data(type=w3099, Variant=w3092) -> (data=w3094:bool)  [unwired: 1 in, 1 out]
            n621 = Set Variant Attribute(Variant=w3098, name=w3095, value=w3094, error in=w3096) -> (Variant out=w3097:variant, error out=w3093:errorcluster)  [unwired: 1 out]
          }
        }
      }
      frame "Phasor Plot:Phasor Plot Active" {
        w3100 = FALSE  # Not a Settings Window Control
        n622 = case shown="True" w3108 {
          tunnel: w3107 -> [w3116 w3120]
          tunnel: w3106 -> [w3115 w3123]
          tunnel: [w3114 w3122] -> w3105
          tunnel: w3104 -> [w3113 w3121]
          tunnel: [w3112 w3118] -> w3103
          tunnel: w3100 -> [w3111 w3124]
          tunnel: [w3109 w3117] -> w3102
          tunnel: w3101 -> [_ w3117]
          frame False {
            n623 = Get Variant Attribute(Variant=w3115, name=w3116, default value (empty Variant)=w3111, error in=w3113) -> (duplicate Variant=w3114:variant, value=w3110:bool, error out=w3112:errorcluster)  [unwired: 1 out]
            n624 = To Variant(anything=w3110) -> (Variant=w3109:variant)
          }
          frame True {
            n625 = Variant To Data(type=w3124, Variant=w3117) -> (data=w3119:bool)  [unwired: 1 in, 1 out]
            n626 = Set Variant Attribute(Variant=w3123, name=w3120, value=w3119, error in=w3121) -> (Variant out=w3122:variant, error out=w3118:errorcluster)  [unwired: 1 out]
          }
        }
      }
      frame "Phasor Plot:Phasor Ratio Color Map Type" {
        n627 = case shown="True" w3133 {
          tunnel: w3132 -> [w3141 w3145]
          tunnel: w3131 -> [w3140 w3148]
          tunnel: [w3139 w3147] -> w3130
          tunnel: w3129 -> [w3138 w3146]
          tunnel: [w3137 w3143] -> w3128
          tunnel: "Phasor Ratio Color Map Type" -> [w3136 w3149]
          tunnel: [w3134 w3142] -> w3127
          tunnel: w3126 -> [_ w3142]
          frame False {
            n628 = Get Variant Attribute(Variant=w3140, name=w3141, default value (empty Variant)=w3136, error in=w3138) -> (duplicate Variant=w3139:variant, value=w3135:T48, error out=w3137:errorcluster)  [unwired: 1 out]
            n629 = To Variant(anything=w3135) -> (Variant=w3134:variant)
          }
          frame True {
            n630 = Variant To Data(type=w3149, Variant=w3142) -> (data=w3144:T48)  [unwired: 1 in, 1 out]
            n631 = Set Variant Attribute(Variant=w3148, name=w3145, value=w3144, error in=w3146) -> (Variant out=w3147:variant, error out=w3143:errorcluster)  [unwired: 1 out]
          }
        }
      }
      frame "Phasor Plot:Phasor Ratio Color Map" {
        n632 = case shown="True" w3158 {
          tunnel: w3157 -> [w3166 w3170]
          tunnel: w3156 -> [w3165 w3173]
          tunnel: [w3164 w3172] -> w3155
          tunnel: w3154 -> [w3163 w3171]
          tunnel: [w3162 w3168] -> w3153
          tunnel: "Phasor Ratio Color Map" -> [w3161 w3174]
          tunnel: [w3159 w3167] -> w3152
          tunnel: w3151 -> [_ w3167]
          frame False {
            n633 = Get Variant Attribute(Variant=w3165, name=w3166, default value (empty Variant)=w3161, error in=w3163) -> (duplicate Variant=w3164:variant, value=w3160:string, error out=w3162:errorcluster)  [unwired: 1 out]
            n634 = To Variant(anything=w3160) -> (Variant=w3159:variant)
          }
          frame True {
            n635 = Variant To Data(type=w3174, Variant=w3167) -> (data=w3169:string)  [unwired: 1 in, 1 out]
            n636 = Set Variant Attribute(Variant=w3173, name=w3170, value=w3169, error in=w3171) -> (Variant out=w3172:variant, error out=w3168:errorcluster)  [unwired: 1 out]
          }
        }
      }
      frame "Phasor Plot:Phasor Ratio Display Range" {
        n637 = Variant To Data(error in=w3177, type=cluster{"Min":dbl, "Max":dbl} {"Min"=0.0, "Max"=1.0} ("Phasor Ratio Display Range"), Variant="Phasor Ratio Display Range") -> (data=w3178:cluster{"Min":dbl, "Max":dbl}, error out=w3176:errorcluster)
        n638 = case shown="True" w3186 {
          tunnel: w3185 -> [w3194 w3198]
          tunnel: w3184 -> [w3193 w3201]
          tunnel: [w3192 w3200] -> w3183
          tunnel: w3176 -> [w3191 w3199]
          tunnel: [w3190 w3196] -> w3182
          tunnel: w3178 -> [w3189 w3202]
          tunnel: [w3187 w3195] -> w3181
          tunnel: w3180 -> [_ w3195]
          frame False {
            n639 = Get Variant Attribute(Variant=w3193, name=w3194, default value (empty Variant)=w3189, error in=w3191) -> (duplicate Variant=w3192:variant, value=w3188:cluster{"Min":dbl, "Max":dbl}, error out=w3190:errorcluster)  [unwired: 1 out]
            n640 = To Variant(anything=w3188) -> (Variant=w3187:variant)
          }
          frame True {
            n641 = Variant To Data(type=w3202, Variant=w3195) -> (data=w3197:cluster{"Min":dbl, "Max":dbl})  [unwired: 1 in, 1 out]
            n642 = Set Variant Attribute(Variant=w3201, name=w3198, value=w3197, error in=w3199) -> (Variant out=w3200:variant, error out=w3196:errorcluster)  [unwired: 1 out]
          }
        }
      }
      frame "Phasor Plot:Selected Image ROI(s)" {
        n643 = case shown="True" w3211 {
          tunnel: w3210 -> [w3219 w3223]
          tunnel: w3209 -> [w3218 w3226]
          tunnel: [w3217 w3225] -> w3208
          tunnel: w3204 -> [w3216 w3224]
          tunnel: [w3215 w3221] -> w3207
          tunnel: "Selected Image ROI(s)" -> [w3214 w3227]
          tunnel: [w3212 w3220] -> w3206
          tunnel: w3205 -> [_ w3220]
          frame False {
            n644 = Get Variant Attribute(Variant=w3218, name=w3219, default value (empty Variant)=w3214, error in=w3216) -> (duplicate Variant=w3217:variant, value=w3213:bool, error out=w3215:errorcluster)  [unwired: 1 out]
            n645 = To Variant(anything=w3213) -> (Variant=w3212:variant)
          }
          frame True {
            n646 = Variant To Data(type=w3227, Variant=w3220) -> (data=w3222:bool)  [unwired: 1 in, 1 out]
            n647 = Set Variant Attribute(Variant=w3226, name=w3223, value=w3222, error in=w3224) -> (Variant out=w3225:variant, error out=w3221:errorcluster)  [unwired: 1 out]
          }
        }
      }
      frame "Phasor Plot:All Image ROIs" {
        n648 = case shown="True" w3236 {
          tunnel: w3235 -> [w3244 w3248]
          tunnel: w3234 -> [w3243 w3251]
          tunnel: [w3242 w3250] -> w3233
          tunnel: w3229 -> [w3241 w3249]
          tunnel: [w3240 w3246] -> w3232
          tunnel: "All Image ROIs" -> [w3239 w3252]
          tunnel: [w3237 w3245] -> w3231
          tunnel: w3230 -> [_ w3245]
          frame False {
            n649 = Get Variant Attribute(Variant=w3243, name=w3244, default value (empty Variant)=w3239, error in=w3241) -> (duplicate Variant=w3242:variant, value=w3238:bool, error out=w3240:errorcluster)  [unwired: 1 out]
            n650 = To Variant(anything=w3238) -> (Variant=w3237:variant)
          }
          frame True {
            n651 = Variant To Data(type=w3252, Variant=w3245) -> (data=w3247:bool)  [unwired: 1 in, 1 out]
            n652 = Set Variant Attribute(Variant=w3251, name=w3248, value=w3247, error in=w3249) -> (Variant out=w3250:variant, error out=w3246:errorcluster)  [unwired: 1 out]
          }
        }
      }
      frame "Phasor Plot:Selected Phasor Plot ROI(s)" {
        n653 = case shown="True" w3261 {
          tunnel: w3260 -> [w3269 w3273]
          tunnel: w3259 -> [w3268 w3276]
          tunnel: [w3267 w3275] -> w3258
          tunnel: w3254 -> [w3266 w3274]
          tunnel: [w3265 w3271] -> w3257
          tunnel: "Selected Phasor Plot ROI(s)" -> [w3264 w3277]
          tunnel: [w3262 w3270] -> w3256
          tunnel: w3255 -> [_ w3270]
          frame False {
            n654 = Get Variant Attribute(Variant=w3268, name=w3269, default value (empty Variant)=w3264, error in=w3266) -> (duplicate Variant=w3267:variant, value=w3263:bool, error out=w3265:errorcluster)  [unwired: 1 out]
            n655 = To Variant(anything=w3263) -> (Variant=w3262:variant)
          }
          frame True {
            n656 = Variant To Data(type=w3277, Variant=w3270) -> (data=w3272:bool)  [unwired: 1 in, 1 out]
            n657 = Set Variant Attribute(Variant=w3276, name=w3273, value=w3272, error in=w3274) -> (Variant out=w3275:variant, error out=w3271:errorcluster)  [unwired: 1 out]
          }
        }
      }
      frame "Phasor Plot:All Phasor Plot ROIs" {
        n658 = case shown="True" w3286 {
          tunnel: w3285 -> [w3294 w3298]
          tunnel: w3284 -> [w3293 w3301]
          tunnel: [w3292 w3300] -> w3283
          tunnel: w3279 -> [w3291 w3299]
          tunnel: [w3290 w3296] -> w3282
          tunnel: "All Phasor Plot ROIs" -> [w3289 w3302]
          tunnel: [w3287 w3295] -> w3281
          tunnel: w3280 -> [_ w3295]
          frame False {
            n659 = Get Variant Attribute(Variant=w3293, name=w3294, default value (empty Variant)=w3289, error in=w3291) -> (duplicate Variant=w3292:variant, value=w3288:bool, error out=w3290:errorcluster)  [unwired: 1 out]
            n660 = To Variant(anything=w3288) -> (Variant=w3287:variant)
          }
          frame True {
            n661 = Variant To Data(type=w3302, Variant=w3295) -> (data=w3297:bool)  [unwired: 1 in, 1 out]
            n662 = Set Variant Attribute(Variant=w3301, name=w3298, value=w3297, error in=w3299) -> (Variant out=w3300:variant, error out=w3296:errorcluster)  [unwired: 1 out]
          }
        }
      }
      frame "Phasor Plot:Phasor Ratio Color-Coded Quantity" {
        n663 = case shown="True" w3311 {
          tunnel: w3310 -> [w3319 w3323]
          tunnel: w3309 -> [w3318 w3326]
          tunnel: [w3317 w3325] -> w3308
          tunnel: w3304 -> [w3316 w3324]
          tunnel: [w3315 w3321] -> w3307
          tunnel: "Phasor Ratio Color-Coded Quantity" -> [w3314 w3327]
          tunnel: [w3312 w3320] -> w3306
          tunnel: w3305 -> [_ w3320]
          frame False {
            n664 = Get Variant Attribute(Variant=w3318, name=w3319, default value (empty Variant)=w3314, error in=w3316) -> (duplicate Variant=w3317:variant, value=w3313:T45, error out=w3315:errorcluster)  [unwired: 1 out]
            n665 = To Variant(anything=w3313) -> (Variant=w3312:variant)
          }
          frame True {
            n666 = Variant To Data(type=w3327, Variant=w3320) -> (data=w3322:T45)  [unwired: 1 in, 1 out]
            n667 = Set Variant Attribute(Variant=w3326, name=w3323, value=w3322, error in=w3324) -> (Variant out=w3325:variant, error out=w3321:errorcluster)  [unwired: 1 out]
          }
        }
      }
      frame "Phasor Plot:Store Phasor Harmonics" {
        n668 = case shown="True" w3336 {
          tunnel: w3335 -> [w3344 w3348]
          tunnel: w3334 -> [w3343 w3351]
          tunnel: [w3342 w3350] -> w3333
          tunnel: w3329 -> [w3341 w3349]
          tunnel: [w3340 w3346] -> w3332
          tunnel: "Store Phasor Harmonics" -> [w3339 w3352]
          tunnel: [w3337 w3345] -> w3331
          tunnel: w3330 -> [_ w3345]
          frame False {
            n669 = Get Variant Attribute(Variant=w3343, name=w3344, default value (empty Variant)=w3339, error in=w3341) -> (duplicate Variant=w3342:variant, value=w3338:bool, error out=w3340:errorcluster)  [unwired: 1 out]
            n670 = To Variant(anything=w3338) -> (Variant=w3337:variant)
          }
          frame True {
            n671 = Variant To Data(type=w3352, Variant=w3345) -> (data=w3347:bool)  [unwired: 1 in, 1 out]
            n672 = Set Variant Attribute(Variant=w3351, name=w3348, value=w3347, error in=w3349) -> (Variant out=w3350:variant, error out=w3346:errorcluster)  [unwired: 1 out]
          }
        }
      }
      frame "Phasor Plot:Draw Reference Segment" {
        n673 = case shown="True" w3361 {
          tunnel: w3360 -> [w3369 w3373]
          tunnel: w3359 -> [w3368 w3376]
          tunnel: [w3367 w3375] -> w3358
          tunnel: w3354 -> [w3366 w3374]
          tunnel: [w3365 w3371] -> w3357
          tunnel: "Draw Reference Segment" -> [w3364 w3377]
          tunnel: [w3362 w3370] -> w3356
          tunnel: w3355 -> [_ w3370]
          frame False {
            n674 = Get Variant Attribute(Variant=w3368, name=w3369, default value (empty Variant)=w3364, error in=w3366) -> (duplicate Variant=w3367:variant, value=w3363:bool, error out=w3365:errorcluster)  [unwired: 1 out]
            n675 = To Variant(anything=w3363) -> (Variant=w3362:variant)
          }
          frame True {
            n676 = Variant To Data(type=w3377, Variant=w3370) -> (data=w3372:bool)  [unwired: 1 in, 1 out]
            n677 = Set Variant Attribute(Variant=w3376, name=w3373, value=w3372, error in=w3374) -> (Variant out=w3375:variant, error out=w3371:errorcluster)  [unwired: 1 out]
          }
        }
      }
      frame "Phasor Plot:User-Defined Quantity" {
        n678 = case shown="True" w3386 {
          tunnel: w3385 -> [w3394 w3398]
          tunnel: w3384 -> [w3393 w3401]
          tunnel: [w3392 w3400] -> w3383
          tunnel: w3379 -> [w3391 w3399]
          tunnel: [w3390 w3396] -> w3382
          tunnel: "User-defined Quantity" -> [w3389 w3402]
          tunnel: [w3387 w3395] -> w3381
          tunnel: w3380 -> [_ w3395]
          frame False {
            n679 = Get Variant Attribute(Variant=w3393, name=w3394, default value (empty Variant)=w3389, error in=w3391) -> (duplicate Variant=w3392:variant, value=w3388:string, error out=w3390:errorcluster)  [unwired: 1 out]
            n680 = To Variant(anything=w3388) -> (Variant=w3387:variant)
          }
          frame True {
            n681 = Variant To Data(type=w3402, Variant=w3395) -> (data=w3397:string)  [unwired: 1 in, 1 out]
            n682 = Set Variant Attribute(Variant=w3401, name=w3398, value=w3397, error in=w3399) -> (Variant out=w3400:variant, error out=w3396:errorcluster)  [unwired: 1 out]
          }
        }
      }
      frame "Phasor Plot:Color Scale High Color" {
        n683 = case shown="True" w3411 {
          tunnel: w3410 -> [w3419 w3423]
          tunnel: w3409 -> [w3418 w3426]
          tunnel: [w3417 w3425] -> w3408
          tunnel: w3404 -> [w3416 w3424]
          tunnel: [w3415 w3421] -> w3407
          tunnel: "High Color" -> [w3414 w3427]
          tunnel: [w3412 w3420] -> w3406
          tunnel: w3405 -> [_ w3420]
          frame False {
            n684 = Get Variant Attribute(Variant=w3418, name=w3419, default value (empty Variant)=w3414, error in=w3416) -> (duplicate Variant=w3417:variant, value=w3413:u32, error out=w3415:errorcluster)  [unwired: 1 out]
            n685 = To Variant(anything=w3413) -> (Variant=w3412:variant)
          }
          frame True {
            n686 = Variant To Data(type=w3427, Variant=w3420) -> (data=w3422:u32)  [unwired: 1 in, 1 out]
            n687 = Set Variant Attribute(Variant=w3426, name=w3423, value=w3422, error in=w3424) -> (Variant out=w3425:variant, error out=w3421:errorcluster)  [unwired: 1 out]
          }
        }
      }
      frame "Phasor Plot:Color Scale Low Color" {
        n688 = case shown="True" w3436 {
          tunnel: w3435 -> [w3444 w3448]
          tunnel: w3434 -> [w3443 w3451]
          tunnel: [w3442 w3450] -> w3433
          tunnel: w3429 -> [w3441 w3449]
          tunnel: [w3440 w3446] -> w3432
          tunnel: "Low Color" -> [w3439 w3452]
          tunnel: [w3437 w3445] -> w3431
          tunnel: w3430 -> [_ w3445]
          frame False {
            n689 = Get Variant Attribute(Variant=w3443, name=w3444, default value (empty Variant)=w3439, error in=w3441) -> (duplicate Variant=w3442:variant, value=w3438:u32, error out=w3440:errorcluster)  [unwired: 1 out]
            n690 = To Variant(anything=w3438) -> (Variant=w3437:variant)
          }
          frame True {
            n691 = Variant To Data(type=w3452, Variant=w3445) -> (data=w3447:u32)  [unwired: 1 in, 1 out]
            n692 = Set Variant Attribute(Variant=w3451, name=w3448, value=w3447, error in=w3449) -> (Variant out=w3450:variant, error out=w3446:errorcluster)  [unwired: 1 out]
          }
        }
      }
      frame "Phasor Plot:Intensity-weighted Phasor Plot" {
        n693 = case shown="True" w3461 {
          tunnel: w3460 -> [w3469 w3473]
          tunnel: w3459 -> [w3468 w3476]
          tunnel: [w3467 w3475] -> w3458
          tunnel: w3454 -> [w3466 w3474]
          tunnel: [w3465 w3471] -> w3457
          tunnel: "Intensity-weighted Phasor Plot" -> [w3464 w3477]
          tunnel: [w3462 w3470] -> w3456
          tunnel: w3455 -> [_ w3470]
          frame False {
            n694 = Get Variant Attribute(Variant=w3468, name=w3469, default value (empty Variant)=w3464, error in=w3466) -> (duplicate Variant=w3467:variant, value=w3463:bool, error out=w3465:errorcluster)  [unwired: 1 out]
            n695 = To Variant(anything=w3463) -> (Variant=w3462:variant)
          }
          frame True {
            n696 = Variant To Data(type=w3477, Variant=w3470) -> (data=w3472:bool)  [unwired: 1 in, 1 out]
            n697 = Set Variant Attribute(Variant=w3476, name=w3473, value=w3472, error in=w3474) -> (Variant out=w3475:variant, error out=w3471:errorcluster)  [unwired: 1 out]
          }
        }
      }
      frame "Phasor Graph:Phasor Frequency" {
        n698 = case shown="True" w3486 {
          tunnel: w3485 -> [w3494 w3498]
          tunnel: w3484 -> [w3493 w3501]
          tunnel: [w3492 w3500] -> w3483
          tunnel: w3482 -> [w3491 w3499]
          tunnel: [w3490 w3496] -> w3481
          tunnel: "Phasor Frequency" -> [w3489 w3502]
          tunnel: [w3487 w3495] -> w3480
          tunnel: w3479 -> [_ w3495]
          frame False {
            n699 = Get Variant Attribute(Variant=w3493, name=w3494, default value (empty Variant)=w3489, error in=w3491) -> (duplicate Variant=w3492:variant, value=w3488:dbl[unit], error out=w3490:errorcluster)  [unwired: 1 out]
            n700 = To Variant(anything=w3488) -> (Variant=w3487:variant)
          }
          frame True {
            n701 = Variant To Data(type=w3502, Variant=w3495) -> (data=w3497:dbl[unit])  [unwired: 1 in, 1 out]
            n702 = Set Variant Attribute(Variant=w3501, name=w3498, value=w3497, error in=w3499) -> (Variant out=w3500:variant, error out=w3496:errorcluster)  [unwired: 1 out]
          }
        }
      }
      frame "Phasor Graph:Phasor Ratio Type" {
        # "item 0: Intensity-weighted\nitem 1: amplitude-weighted"
        n703 = case shown="True" w3511 {
          tunnel: w3510 -> [w3519 w3523]
          tunnel: w3509 -> [w3518 w3526]
          tunnel: [w3517 w3525] -> w3508
          tunnel: w3507 -> [w3516 w3524]
          tunnel: [w3515 w3521] -> w3506
          tunnel: "Phasor Ratio Type" -> [w3514 w3527]
          tunnel: [w3512 w3520] -> w3505
          tunnel: w3504 -> [_ w3520]
          frame False {
            n704 = Get Variant Attribute(Variant=w3518, name=w3519, default value (empty Variant)=w3514, error in=w3516) -> (duplicate Variant=w3517:variant, value=w3513:T53, error out=w3515:errorcluster)  [unwired: 1 out]
            n705 = To Variant(anything=w3513) -> (Variant=w3512:variant)
          }
          frame True {
            n706 = Variant To Data(type=w3527, Variant=w3520) -> (data=w3522:T53)  [unwired: 1 in, 1 out]
            n707 = Set Variant Attribute(Variant=w3526, name=w3523, value=w3522, error in=w3524) -> (Variant out=w3525:variant, error out=w3521:errorcluster)  [unwired: 1 out]
          }
        }
      }
      frame "Phasor Graph:Pixel-level Phasor Computation" {
        n708 = case shown="True" w3536 {
          tunnel: w3535 -> [w3544 w3548]
          tunnel: w3534 -> [w3543 w3551]
          tunnel: [w3542 w3550] -> w3533
          tunnel: w3532 -> [w3541 w3549]
          tunnel: [w3540 w3546] -> w3531
          tunnel: "Pixel-level Phasor Computation" -> [w3539 w3552]
          tunnel: [w3537 w3545] -> w3530
          tunnel: w3529 -> [_ w3545]
          frame False {
            n709 = Get Variant Attribute(Variant=w3543, name=w3544, default value (empty Variant)=w3539, error in=w3541) -> (duplicate Variant=w3542:variant, value=w3538:bool, error out=w3540:errorcluster)  [unwired: 1 out]
            n710 = To Variant(anything=w3538) -> (Variant=w3537:variant)
          }
          frame True {
            n711 = Variant To Data(type=w3552, Variant=w3545) -> (data=w3547:bool)  [unwired: 1 in, 1 out]
            n712 = Set Variant Attribute(Variant=w3551, name=w3548, value=w3547, error in=w3549) -> (Variant out=w3550:variant, error out=w3546:errorcluster)  [unwired: 1 out]
          }
        }
      }
      frame "Phasor Graph:Save Phasor Graph" {
        n713 = case shown="True" w3561 {
          tunnel: w3560 -> [w3569 w3573]
          tunnel: w3559 -> [w3568 w3576]
          tunnel: [w3567 w3575] -> w3558
          tunnel: w3557 -> [w3566 w3574]
          tunnel: [w3565 w3571] -> w3556
          tunnel: "Save Phasor Graph Image" -> [w3564 w3577]
          tunnel: [w3562 w3570] -> w3555
          tunnel: w3554 -> [_ w3570]
          frame False {
            n714 = Get Variant Attribute(Variant=w3568, name=w3569, default value (empty Variant)=w3564, error in=w3566) -> (duplicate Variant=w3567:variant, value=w3563:bool, error out=w3565:errorcluster)  [unwired: 1 out]
            n715 = To Variant(anything=w3563) -> (Variant=w3562:variant)
          }
          frame True {
            n716 = Variant To Data(type=w3577, Variant=w3570) -> (data=w3572:bool)  [unwired: 1 in, 1 out]
            n717 = Set Variant Attribute(Variant=w3576, name=w3573, value=w3572, error in=w3574) -> (Variant out=w3575:variant, error out=w3571:errorcluster)  [unwired: 1 out]
          }
        }
      }
      frame "Phasor Graph:Phasor Graph Active" {
        n718 = case shown="True" w3586 {
          tunnel: w3585 -> [w3594 w3598]
          tunnel: w3584 -> [w3593 w3601]
          tunnel: [w3592 w3600] -> w3583
          tunnel: w3582 -> [w3591 w3599]
          tunnel: [w3590 w3596] -> w3581
          tunnel: "Phasor Graph Active" -> [w3589 w3602]
          tunnel: [w3587 w3595] -> w3580
          tunnel: w3579 -> [_ w3595]
          frame False {
            n719 = Get Variant Attribute(Variant=w3593, name=w3594, default value (empty Variant)=w3589, error in=w3591) -> (duplicate Variant=w3592:variant, value=w3588:bool, error out=w3590:errorcluster)  [unwired: 1 out]
            n720 = To Variant(anything=w3588) -> (Variant=w3587:variant)
          }
          frame True {
            n721 = Variant To Data(type=w3602, Variant=w3595) -> (data=w3597:bool)  [unwired: 1 in, 1 out]
            n722 = Set Variant Attribute(Variant=w3601, name=w3598, value=w3597, error in=w3599) -> (Variant out=w3600:variant, error out=w3596:errorcluster)  [unwired: 1 out]
          }
        }
      }
      frame "Phasor Graph:Phasor SDV Options" {
        n723 = case shown="True" w3611 {
          tunnel: w3610 -> [w3619 w3623]
          tunnel: w3609 -> [w3618 w3626]
          tunnel: [w3617 w3625] -> w3608
          tunnel: w3607 -> [w3616 w3624]
          tunnel: [w3615 w3621] -> w3606
          tunnel: "Phasor SDV Options" -> [w3614 w3627]
          tunnel: [w3612 w3620] -> w3605
          tunnel: w3604 -> [_ w3620]
          frame False {
            n724 = Get Variant Attribute(Variant=w3618, name=w3619, default value (empty Variant)=w3614, error in=w3616) -> (duplicate Variant=w3617:variant, value=w3613:T51, error out=w3615:errorcluster)  [unwired: 1 out]
            n725 = To Variant(anything=w3613) -> (Variant=w3612:variant)
          }
          frame True {
            n726 = Variant To Data(type=w3627, Variant=w3620) -> (data=w3622:T51)  [unwired: 1 in, 1 out]
            n727 = Set Variant Attribute(Variant=w3626, name=w3623, value=w3622, error in=w3624) -> (Variant out=w3625:variant, error out=w3621:errorcluster)  [unwired: 1 out]
          }
        }
      }
      frame "Phasor Graph:Intensity-weighted Phasor Graph" {
        n728 = case shown="True" w3636 {
          tunnel: w3635 -> [w3644 w3648]
          tunnel: w3634 -> [w3643 w3651]
          tunnel: [w3642 w3650] -> w3633
          tunnel: w3632 -> [w3641 w3649]
          tunnel: [w3640 w3646] -> w3631
          tunnel: "Intensity-weighted Phasor Graph" -> [w3639 w3652]
          tunnel: [w3637 w3645] -> w3630
          tunnel: w3629 -> [_ w3645]
          frame False {
            n729 = Get Variant Attribute(Variant=w3643, name=w3644, default value (empty Variant)=w3639, error in=w3641) -> (duplicate Variant=w3642:variant, value=w3638:bool, error out=w3640:errorcluster)  [unwired: 1 out]
            n730 = To Variant(anything=w3638) -> (Variant=w3637:variant)
          }
          frame True {
            n731 = Variant To Data(type=w3652, Variant=w3645) -> (data=w3647:bool)  [unwired: 1 in, 1 out]
            n732 = Set Variant Attribute(Variant=w3651, name=w3648, value=w3647, error in=w3649) -> (Variant out=w3650:variant, error out=w3646:errorcluster)  [unwired: 1 out]
          }
        }
      }
      frame "Phasor Calibration:Use Backup Calibration if needed" {
        n733 = case shown="True" w3661 {
          tunnel: w3660 -> [w3669 w3673]
          tunnel: w3659 -> [w3668 w3676]
          tunnel: [w3667 w3675] -> w3658
          tunnel: w3657 -> [w3666 w3674]
          tunnel: [w3665 w3671] -> w3656
          tunnel: "Use Backup Calibration if needed" -> [w3664 w3677]
          tunnel: [w3662 w3670] -> w3655
          tunnel: w3654 -> [_ w3670]
          frame False {
            n734 = Get Variant Attribute(Variant=w3668, name=w3669, default value (empty Variant)=w3664, error in=w3666) -> (duplicate Variant=w3667:variant, value=w3663:bool, error out=w3665:errorcluster)  [unwired: 1 out]
            n735 = To Variant(anything=w3663) -> (Variant=w3662:variant)
          }
          frame True {
            n736 = Variant To Data(type=w3677, Variant=w3670) -> (data=w3672:bool)  [unwired: 1 in, 1 out]
            n737 = Set Variant Attribute(Variant=w3676, name=w3673, value=w3672, error in=w3674) -> (Variant out=w3675:variant, error out=w3671:errorcluster)  [unwired: 1 out]
          }
        }
      }
      frame "Phasor Graph:Define Shortest Lifetime as" {
        n738 = case shown="True" w3686 {
          tunnel: w3685 -> [w3694 w3698]
          tunnel: w3684 -> [w3693 w3701]
          tunnel: [w3692 w3700] -> w3683
          tunnel: w3682 -> [w3691 w3699]
          tunnel: [w3690 w3696] -> w3681
          tunnel: "Define Shortest Lifetime as" -> [w3689 w3702]
          tunnel: [w3687 w3695] -> w3680
          tunnel: w3679 -> [_ w3695]
          frame False {
            n739 = Get Variant Attribute(Variant=w3693, name=w3694, default value (empty Variant)=w3689, error in=w3691) -> (duplicate Variant=w3692:variant, value=w3688:T52, error out=w3690:errorcluster)  [unwired: 1 out]
            n740 = To Variant(anything=w3688) -> (Variant=w3687:variant)
          }
          frame True {
            n741 = Variant To Data(type=w3702, Variant=w3695) -> (data=w3697:T52)  [unwired: 1 in, 1 out]
            n742 = Set Variant Attribute(Variant=w3701, name=w3698, value=w3697, error in=w3699) -> (Variant out=w3700:variant, error out=w3696:errorcluster)  [unwired: 1 out]
          }
        }
      }
      frame "Phasor Calibration:Backup Calibration Type" {
        n743 = case shown="True" w3711 {
          tunnel: w3710 -> [w3719 w3723]
          tunnel: w3709 -> [w3718 w3726]
          tunnel: [w3717 w3725] -> w3708
          tunnel: w3707 -> [w3716 w3724]
          tunnel: [w3715 w3721] -> w3706
          tunnel: "Backup Calibration Type" -> [w3714 w3727]
          tunnel: [w3712 w3720] -> w3705
          tunnel: w3704 -> [_ w3720]
          frame False {
            n744 = Get Variant Attribute(Variant=w3718, name=w3719, default value (empty Variant)=w3714, error in=w3716) -> (duplicate Variant=w3717:variant, value=w3713:T66, error out=w3715:errorcluster)  [unwired: 1 out]
            n745 = To Variant(anything=w3713) -> (Variant=w3712:variant)
          }
          frame True {
            n746 = Variant To Data(type=w3727, Variant=w3720) -> (data=w3722:T66)  [unwired: 1 in, 1 out]
            n747 = Set Variant Attribute(Variant=w3726, name=w3723, value=w3722, error in=w3724) -> (Variant out=w3725:variant, error out=w3721:errorcluster)  [unwired: 1 out]
          }
        }
      }
      frame "Phasor Calibration:Calibration Type" {
        n748 = case shown="True" w3736 {
          tunnel: w3735 -> [w3744 w3748]
          tunnel: w3734 -> [w3743 w3751]
          tunnel: [w3742 w3750] -> w3733
          tunnel: w3732 -> [w3741 w3749]
          tunnel: [w3740 w3746] -> w3731
          tunnel: "Calibration Type" -> [w3739 w3752]
          tunnel: [w3737 w3745] -> w3730
          tunnel: w3729 -> [_ w3745]
          frame False {
            n749 = Get Variant Attribute(Variant=w3743, name=w3744, default value (empty Variant)=w3739, error in=w3741) -> (duplicate Variant=w3742:variant, value=w3738:T65, error out=w3740:errorcluster)  [unwired: 1 out]
            n750 = To Variant(anything=w3738) -> (Variant=w3737:variant)
          }
          frame True {
            n751 = Variant To Data(type=w3752, Variant=w3745) -> (data=w3747:T65)  [unwired: 1 in, 1 out]
            n752 = Set Variant Attribute(Variant=w3751, name=w3748, value=w3747, error in=w3749) -> (Variant out=w3750:variant, error out=w3746:errorcluster)  [unwired: 1 out]
          }
        }
      }
      frame "Phasor Calibration:Calibration Lifetime" {
        n753 = case shown="True" w3761 {
          tunnel: w3760 -> [w3769 w3773]
          tunnel: w3759 -> [w3768 w3776]
          tunnel: [w3767 w3775] -> w3758
          tunnel: w3757 -> [w3766 w3774]
          tunnel: [w3765 w3771] -> w3756
          tunnel: "Calibration Lifetime" -> [w3764 w3777]
          tunnel: [w3762 w3770] -> w3755
          tunnel: w3754 -> [_ w3770]
          frame False {
            n754 = Get Variant Attribute(Variant=w3768, name=w3769, default value (empty Variant)=w3764, error in=w3766) -> (duplicate Variant=w3767:variant, value=w3763:dbl[unit], error out=w3765:errorcluster)  [unwired: 1 out]
            n755 = To Variant(anything=w3763) -> (Variant=w3762:variant)
          }
          frame True {
            n756 = Variant To Data(type=w3777, Variant=w3770) -> (data=w3772:dbl[unit])  [unwired: 1 in, 1 out]
            n757 = Set Variant Attribute(Variant=w3776, name=w3773, value=w3772, error in=w3774) -> (Variant out=w3775:variant, error out=w3771:errorcluster)  [unwired: 1 out]
          }
        }
      }
      frame "Phasor Calibration:Calibration Map Algorithm" {
        n758 = case shown="True" w3786 {
          tunnel: w3785 -> [w3794 w3798]
          tunnel: w3784 -> [w3793 w3801]
          tunnel: [w3792 w3800] -> w3783
          tunnel: w3782 -> [w3791 w3799]
          tunnel: [w3790 w3796] -> w3781
          tunnel: "Calibration Map Algorithm" -> [w3789 w3802]
          tunnel: [w3787 w3795] -> w3780
          tunnel: w3779 -> [_ w3795]
          frame False {
            n759 = Get Variant Attribute(Variant=w3793, name=w3794, default value (empty Variant)=w3789, error in=w3791) -> (duplicate Variant=w3792:variant, value=w3788:T64, error out=w3790:errorcluster)  [unwired: 1 out]
            n760 = To Variant(anything=w3788) -> (Variant=w3787:variant)
          }
          frame True {
            n761 = Variant To Data(type=w3802, Variant=w3795) -> (data=w3797:T64)  [unwired: 1 in, 1 out]
            n762 = Set Variant Attribute(Variant=w3801, name=w3798, value=w3797, error in=w3799) -> (Variant out=w3800:variant, error out=w3796:errorcluster)  [unwired: 1 out]
          }
        }
      }
      frame "Single-Exponential Phasor Locus (SEPL):Gate Parameters" {
        n763 = case shown="True" w3811 {
          tunnel: w3810 -> [w3819 w3823]
          tunnel: w3809 -> [w3818 w3826]
          tunnel: [w3817 w3825] -> w3808
          tunnel: w3807 -> [w3816 w3824]
          tunnel: [w3815 w3821] -> w3806
          tunnel: "SEPL Gate Parameters" -> [w3814 w3827]
          tunnel: [w3812 w3820] -> w3805
          tunnel: w3804 -> [_ w3820]
          frame False {
            n764 = Get Variant Attribute(Variant=w3818, name=w3819, default value (empty Variant)=w3814, error in=w3816) -> (duplicate Variant=w3817:variant, value=w3813:T61, error out=w3815:errorcluster)  [unwired: 1 out]
            n765 = To Variant(anything=w3813) -> (Variant=w3812:variant)
          }
          frame True {
            n766 = Variant To Data(type=w3827, Variant=w3820) -> (data=w3822:T61)  [unwired: 1 in, 1 out]
            n767 = Set Variant Attribute(Variant=w3826, name=w3823, value=w3822, error in=w3824) -> (Variant out=w3825:variant, error out=w3821:errorcluster)  [unwired: 1 out]
          }
        }
      }
      frame "Single-Exponential Phasor Locus (SEPL):User-defined Gate" {
        n768 = case shown="True" w3836 {
          tunnel: w3835 -> [w3844 w3849]
          tunnel: w3834 -> [w3843 w3852]
          tunnel: [w3842 w3851] -> w3833
          tunnel: w3832 -> [w3841 w3850]
          tunnel: [w3840 w3848] -> w3831
          tunnel: T78 {"X Array"=[], "Y Array"=[]} ("Plot") -> [w3839 w3846]
          tunnel: [w3837 w3847] -> w3830
          tunnel: w3829 -> [_ w3847]
          frame False {
            n769 = Get Variant Attribute(Variant=w3843, name=w3844, default value (empty Variant)=w3839, error in=w3841) -> (duplicate Variant=w3842:variant, value=w3838:T78, error out=w3840:errorcluster)  [unwired: 1 out]
            n770 = To Variant(anything=w3838) -> (Variant=w3837:variant)
          }
          frame True {
            n771 = Variant To Data(type=w3846, Variant=w3847) -> (data=w3845:T78)  [unwired: 1 in, 1 out]
            n772 = global write "Phasor User-defined Gate & IRF.vi" "User-defined Gate"(w3845) -> ()
            n773 = Set Variant Attribute(Variant=w3852, name=w3849, value=w3845, error in=w3850) -> (Variant out=w3851:variant, error out=w3848:errorcluster)  [unwired: 1 out]
          }
        }
      }
      frame "Single-Exponential Phasor Locus (SEPL):User-defined IRF" {
        n774 = case shown="True" w3861 {
          tunnel: w3860 -> [w3869 w3874]
          tunnel: w3859 -> [w3868 w3877]
          tunnel: [w3867 w3876] -> w3858
          tunnel: w3857 -> [w3866 w3875]
          tunnel: [w3865 w3873] -> w3856
          tunnel: T78 {"X Array"=[], "Y Array"=[]} ("Plot") -> [w3864 w3871]
          tunnel: [w3862 w3872] -> w3855
          tunnel: w3854 -> [_ w3872]
          frame False {
            n775 = Get Variant Attribute(Variant=w3868, name=w3869, default value (empty Variant)=w3864, error in=w3866) -> (duplicate Variant=w3867:variant, value=w3863:T78, error out=w3865:errorcluster)  [unwired: 1 out]
            n776 = To Variant(anything=w3863) -> (Variant=w3862:variant)
          }
          frame True {
            n777 = Variant To Data(type=w3871, Variant=w3872) -> (data=w3870:T78)  [unwired: 1 in, 1 out]
            n778 = global write "Phasor User-defined Gate & IRF.vi" "User-defined IRF"(w3870) -> ()
            n779 = Set Variant Attribute(Variant=w3877, name=w3874, value=w3870, error in=w3875) -> (Variant out=w3876:variant, error out=w3873:errorcluster)  [unwired: 1 out]
          }
        }
      }
      frame "Single-Exponential Phasor Locus (SEPL):Phasor Parameters" {
        n780 = case shown="True" w3886 {
          tunnel: w3885 -> [w3894 w3898]
          tunnel: w3884 -> [w3893 w3901]
          tunnel: [w3892 w3900] -> w3883
          tunnel: w3882 -> [w3891 w3899]
          tunnel: [w3890 w3896] -> w3881
          tunnel: "SEPL Phasor Parameters" -> [w3889 w3902]
          tunnel: [w3887 w3895] -> w3880
          tunnel: w3879 -> [_ w3895]
          frame False {
            n781 = Get Variant Attribute(Variant=w3893, name=w3894, default value (empty Variant)=w3889, error in=w3891) -> (duplicate Variant=w3892:variant, value=w3888:T56, error out=w3890:errorcluster)  [unwired: 1 out]
            n782 = To Variant(anything=w3888) -> (Variant=w3887:variant)
          }
          frame True {
            n783 = Variant To Data(type=w3902, Variant=w3895) -> (data=w3897:T56)  [unwired: 1 in, 1 out]
            n784 = Set Variant Attribute(Variant=w3901, name=w3898, value=w3897, error in=w3899) -> (Variant out=w3900:variant, error out=w3896:errorcluster)  [unwired: 1 out]
          }
        }
      }
      frame "Single-Exponential Phasor Locus (SEPL):Decay & IRF Parameters" {
        n785 = case shown="True" w3911 {
          tunnel: w3910 -> [w3919 w3923]
          tunnel: w3909 -> [w3918 w3926]
          tunnel: [w3917 w3925] -> w3908
          tunnel: w3907 -> [w3916 w3924]
          tunnel: [w3915 w3921] -> w3906
          tunnel: "SEPL IRF Parameters" -> [w3914 w3927]
          tunnel: [w3912 w3920] -> w3905
          tunnel: w3904 -> [_ w3920]
          frame False {
            n786 = Get Variant Attribute(Variant=w3918, name=w3919, default value (empty Variant)=w3914, error in=w3916) -> (duplicate Variant=w3917:variant, value=w3913:T59, error out=w3915:errorcluster)  [unwired: 1 out]
            n787 = To Variant(anything=w3913) -> (Variant=w3912:variant)
          }
          frame True {
            n788 = Variant To Data(type=w3927, Variant=w3920) -> (data=w3922:T59)  [unwired: 1 in, 1 out]
            n789 = Set Variant Attribute(Variant=w3926, name=w3923, value=w3922, error in=w3924) -> (Variant out=w3925:variant, error out=w3921:errorcluster)  [unwired: 1 out]
          }
        }
      }
      frame "Single-Exponential Phasor Locus (SEPL):Display Parameters" {
        n790 = case shown="True" w3936 {
          tunnel: w3935 -> [w3944 w3948]
          tunnel: w3934 -> [w3943 w3951]
          tunnel: [w3942 w3950] -> w3933
          tunnel: w3932 -> [w3941 w3949]
          tunnel: [w3940 w3946] -> w3931
          tunnel: "SEPL Display Parameters" -> [w3939 w3952]
          tunnel: [w3937 w3945] -> w3930
          tunnel: w3929 -> [_ w3945]
          frame False {
            n791 = Get Variant Attribute(Variant=w3943, name=w3944, default value (empty Variant)=w3939, error in=w3941) -> (duplicate Variant=w3942:variant, value=w3938:T54, error out=w3940:errorcluster)  [unwired: 1 out]
            n792 = To Variant(anything=w3938) -> (Variant=w3937:variant)
          }
          frame True {
            n793 = Variant To Data(type=w3952, Variant=w3945) -> (data=w3947:T54)  [unwired: 1 in, 1 out]
            n794 = Set Variant Attribute(Variant=w3951, name=w3948, value=w3947, error in=w3949) -> (Variant out=w3950:variant, error out=w3946:errorcluster)  [unwired: 1 out]
          }
        }
      }
      frame "Lifetime Analysis:Decay Analysis Parameters" {
        n795 = case shown="True" w3961 {
          tunnel: w3960 -> [w3969 w3973]
          tunnel: w3959 -> [w3968 w3976]
          tunnel: [w3967 w3975] -> w3958
          tunnel: w3957 -> [w3966 w3974]
          tunnel: [w3965 w3971] -> w3956
          tunnel: "Decay Analysis Parameters" -> [w3964 w3977]
          tunnel: [w3962 w3970] -> w3955
          tunnel: w3954 -> [_ w3970]
          frame False {
            n796 = Get Variant Attribute(Variant=w3968, name=w3969, default value (empty Variant)=w3964, error in=w3966) -> (duplicate Variant=w3967:variant, value=w3963:T20, error out=w3965:errorcluster)  [unwired: 1 out]
            n797 = To Variant(anything=w3963) -> (Variant=w3962:variant)
          }
          frame True {
            n798 = Variant To Data(type=w3977, Variant=w3970) -> (data=w3972:T20)  [unwired: 1 in, 1 out]
            n799 = Set Variant Attribute(Variant=w3976, name=w3973, value=w3972, error in=w3974) -> (Variant out=w3975:variant, error out=w3971:errorcluster)  [unwired: 1 out]
          }
        }
      }
      frame "Lifetime Analysis:Lifetime Map Active" {
        w3978 = FALSE  # Not a Settings Window Control
        n800 = case shown="True" w3986 {
          tunnel: w3985 -> [w3994 w3998]
          tunnel: w3984 -> [w3993 w4001]
          tunnel: [w3992 w4000] -> w3983
          tunnel: w3982 -> [w3991 w3999]
          tunnel: [w3990 w3996] -> w3981
          tunnel: w3978 -> [w3989 w4002]
          tunnel: [w3987 w3995] -> w3980
          tunnel: w3979 -> [_ w3995]
          frame False {
            n801 = Get Variant Attribute(Variant=w3993, name=w3994, default value (empty Variant)=w3989, error in=w3991) -> (duplicate Variant=w3992:variant, value=w3988:bool, error out=w3990:errorcluster)  [unwired: 1 out]
            n802 = To Variant(anything=w3988) -> (Variant=w3987:variant)
          }
          frame True {
            n803 = Variant To Data(type=w4002, Variant=w3995) -> (data=w3997:bool)  [unwired: 1 in, 1 out]
            n804 = Set Variant Attribute(Variant=w4001, name=w3998, value=w3997, error in=w3999) -> (Variant out=w4000:variant, error out=w3996:errorcluster)  [unwired: 1 out]
          }
        }
      }
      frame "Plugins:Python Settings" {
        n805 = case shown="False" w4011 {
          tunnel: w4010 -> [w4019 w4023]
          tunnel: w4009 -> [w4018 w4026]
          tunnel: [w4017 w4025] -> w4008
          tunnel: w4007 -> [w4016 w4024]
          tunnel: [w4015 w4021] -> w4006
          tunnel: "Python Settings" -> [w4014 w4027]
          tunnel: [w4012 w4020] -> w4005
          tunnel: w4004 -> [_ w4020]
          frame False {
            n806 = Get Variant Attribute(Variant=w4018, name=w4019, default value (empty Variant)=w4014, error in=w4016) -> (duplicate Variant=w4017:variant, value=w4013:T67, error out=w4015:errorcluster)  [unwired: 1 out]
            n807 = To Variant(anything=w4013) -> (Variant=w4012:variant)
          }
          frame True {
            n808 = Variant To Data(type=w4027, Variant=w4020) -> (data=w4022:T67)  [unwired: 1 in, 1 out]
            n809 = Set Variant Attribute(Variant=w4026, name=w4023, value=w4022, error in=w4024) -> (Variant out=w4025:variant, error out=w4021:errorcluster)  [unwired: 1 out]
          }
        }
      }
      frame "Miscellaneous:Verbose Mode" {
        n810 = case shown="True" w4036 {
          tunnel: w4035 -> [w4044 w4049]
          tunnel: w4034 -> [w4043 w4052]
          tunnel: [w4042 w4051] -> w4033
          tunnel: w4032 -> [w4041 w4050]
          tunnel: [w4040 w4048] -> w4031
          tunnel: "Verbose Mode" -> [w4039 w4046]
          tunnel: [w4037 w4047] -> w4030
          tunnel: w4029 -> [_ w4047]
          frame False {
            n811 = Get Variant Attribute(Variant=w4043, name=w4044, default value (empty Variant)=w4039, error in=w4041) -> (duplicate Variant=w4042:variant, value=w4038:bool, error out=w4040:errorcluster)  [unwired: 1 out]
            n812 = To Variant(anything=w4038) -> (Variant=w4037:variant)
          }
          frame True {
            n813 = Variant To Data(type=w4046, Variant=w4047) -> (data=w4045:bool)  [unwired: 1 in, 1 out]
            n814 = Set Variant Attribute(Variant=w4052, name=w4049, value=w4045, error in=w4050) -> (Variant out=w4051:variant, error out=w4048:errorcluster)  [unwired: 1 out]
          }
        }
      }
      frame "Miscellaneous:Beep after Script" {
        n815 = case shown="True" w4061 {
          tunnel: w4060 -> [w4069 w4073]
          tunnel: w4059 -> [w4068 w4076]
          tunnel: [w4067 w4075] -> w4058
          tunnel: w4057 -> [w4066 w4074]
          tunnel: [w4065 w4071] -> w4056
          tunnel: "Beep after Script" -> [w4064 w4077]
          tunnel: [w4062 w4070] -> w4055
          tunnel: w4054 -> [_ w4070]
          frame False {
            n816 = Get Variant Attribute(Variant=w4068, name=w4069, default value (empty Variant)=w4064, error in=w4066) -> (duplicate Variant=w4067:variant, value=w4063:bool, error out=w4065:errorcluster)  [unwired: 1 out]
            n817 = To Variant(anything=w4063) -> (Variant=w4062:variant)
          }
          frame True {
            n818 = Variant To Data(type=w4077, Variant=w4070) -> (data=w4072:bool)  [unwired: 1 in, 1 out]
            n819 = Set Variant Attribute(Variant=w4076, name=w4073, value=w4072, error in=w4074) -> (Variant out=w4075:variant, error out=w4071:errorcluster)  [unwired: 1 out]
          }
        }
      }
      frame "Miscellaneous:Saved Image File Format" {
        n820 = case shown="False" w4086 {
          tunnel: w4085 -> [w4094 w4098]
          tunnel: w4084 -> [w4093 w4101]
          tunnel: [w4092 w4100] -> w4083
          tunnel: w4082 -> [w4091 w4099]
          tunnel: [w4090 w4096] -> w4081
          tunnel: "Saved Displayed Image File Format" -> [w4089 w4102]
          tunnel: [w4087 w4095] -> w4080
          tunnel: w4079 -> [_ w4095]
          frame False {
            n821 = Get Variant Attribute(Variant=w4093, name=w4094, default value (empty Variant)=w4089, error in=w4091) -> (duplicate Variant=w4092:variant, value=w4088:T72, error out=w4090:errorcluster)  [unwired: 1 out]
            n822 = To Variant(anything=w4088) -> (Variant=w4087:variant)
          }
          frame True {
            n823 = Variant To Data(type=w4102, Variant=w4095) -> (data=w4097:T72)  [unwired: 1 in, 1 out]
            n824 = Set Variant Attribute(Variant=w4101, name=w4098, value=w4097, error in=w4099) -> (Variant out=w4100:variant, error out=w4096:errorcluster)  [unwired: 1 out]
          }
        }
      }
      frame "Miscellaneous:Exported Gate Image Settings" {
        n825 = case shown="False" w4111 {
          tunnel: w4110 -> [w4119 w4123]
          tunnel: w4109 -> [w4118 w4126]
          tunnel: [w4117 w4125] -> w4108
          tunnel: w4107 -> [w4116 w4124]
          tunnel: [w4115 w4121] -> w4106
          tunnel: "Exported Gate Image Settings" -> [w4114 w4127]
          tunnel: [w4112 w4120] -> w4105
          tunnel: w4104 -> [_ w4120]
          frame False {
            n826 = Get Variant Attribute(Variant=w4118, name=w4119, default value (empty Variant)=w4114, error in=w4116) -> (duplicate Variant=w4117:variant, value=w4113:T71, error out=w4115:errorcluster)  [unwired: 1 out]
            n827 = To Variant(anything=w4113) -> (Variant=w4112:variant)
          }
          frame True {
            n828 = Variant To Data(type=w4127, Variant=w4120) -> (data=w4122:T71)  [unwired: 1 in, 1 out]
            n829 = Set Variant Attribute(Variant=w4126, name=w4123, value=w4122, error in=w4124) -> (Variant out=w4125:variant, error out=w4121:errorcluster)  [unwired: 1 out]
          }
        }
      }
      frame "Miscellaneous:Include Loading in Timing" {
        n830 = case shown="True" w4136 {
          tunnel: w4135 -> [w4144 w4148]
          tunnel: w4134 -> [w4143 w4151]
          tunnel: [w4142 w4150] -> w4133
          tunnel: w4132 -> [w4141 w4149]
          tunnel: [w4140 w4146] -> w4131
          tunnel: "Include Loading in Timing" -> [w4139 w4152]
          tunnel: [w4137 w4145] -> w4130
          tunnel: w4129 -> [_ w4145]
          frame False {
            n831 = Get Variant Attribute(Variant=w4143, name=w4144, default value (empty Variant)=w4139, error in=w4141) -> (duplicate Variant=w4142:variant, value=w4138:bool, error out=w4140:errorcluster)  [unwired: 1 out]
            n832 = To Variant(anything=w4138) -> (Variant=w4137:variant)
          }
          frame True {
            n833 = Variant To Data(type=w4152, Variant=w4145) -> (data=w4147:bool)  [unwired: 1 in, 1 out]
            n834 = Set Variant Attribute(Variant=w4151, name=w4148, value=w4147, error in=w4149) -> (Variant out=w4150:variant, error out=w4146:errorcluster)  [unwired: 1 out]
          }
        }
      }
      frame "Miscellaneous:Verbose Settings Mode" {
        n835 = case shown="False" w4161 {
          tunnel: w4160 -> [w4169 w4173]
          tunnel: w4159 -> [w4168 w4176]
          tunnel: [w4167 w4175] -> w4158
          tunnel: w4157 -> [w4166 w4174]
          tunnel: [w4165 w4171] -> w4156
          tunnel: "Verbose Settings Mode" -> [w4164 w4177]
          tunnel: [w4162 w4170] -> w4155
          tunnel: w4154 -> [_ w4170]
          frame False {
            n836 = Get Variant Attribute(Variant=w4168, name=w4169, default value (empty Variant)=w4164, error in=w4166) -> (duplicate Variant=w4167:variant, value=w4163:bool, error out=w4165:errorcluster)  [unwired: 1 out]
            n837 = To Variant(anything=w4163) -> (Variant=w4162:variant)
          }
          frame True {
            n838 = Variant To Data(type=w4177, Variant=w4170) -> (data=w4172:bool)  [unwired: 1 in, 1 out]
            n839 = Set Variant Attribute(Variant=w4176, name=w4173, value=w4172, error in=w4174) -> (Variant out=w4175:variant, error out=w4171:errorcluster)  [unwired: 1 out]
          }
        }
      }
      frame "Miscellaneous:Histogram Options" {
        n840 = case shown="False" w4186 {
          tunnel: w4185 -> [w4194 w4198]
          tunnel: w4184 -> [w4193 w4201]
          tunnel: [w4192 w4200] -> w4183
          tunnel: w4182 -> [w4191 w4199]
          tunnel: [w4190 w4196] -> w4181
          tunnel: "Histogram Options" -> [w4189 w4202]
          tunnel: [w4187 w4195] -> w4180
          tunnel: w4179 -> [_ w4195]
          frame False {
            n841 = Get Variant Attribute(Variant=w4193, name=w4194, default value (empty Variant)=w4189, error in=w4191) -> (duplicate Variant=w4192:variant, value=w4188:T68, error out=w4190:errorcluster)  [unwired: 1 out]
            n842 = To Variant(anything=w4188) -> (Variant=w4187:variant)
          }
          frame True {
            n843 = Variant To Data(type=w4202, Variant=w4195) -> (data=w4197:T68)  [unwired: 1 in, 1 out]
            n844 = Set Variant Attribute(Variant=w4201, name=w4198, value=w4197, error in=w4199) -> (Variant out=w4200:variant, error out=w4196:errorcluster)  [unwired: 1 out]
          }
        }
      }
      frame "Miscellaneous:Beep on Error" {
        n845 = case shown="False" w4211 {
          tunnel: w4210 -> [w4219 w4223]
          tunnel: w4209 -> [w4218 w4226]
          tunnel: [w4217 w4225] -> w4208
          tunnel: w4207 -> [w4216 w4224]
          tunnel: [w4215 w4221] -> w4206
          tunnel: "Beep on Error" -> [w4214 w4227]
          tunnel: [w4212 w4220] -> w4205
          tunnel: w4204 -> [_ w4220]
          frame False {
            n846 = Get Variant Attribute(Variant=w4218, name=w4219, default value (empty Variant)=w4214, error in=w4216) -> (duplicate Variant=w4217:variant, value=w4213:bool, error out=w4215:errorcluster)  [unwired: 1 out]
            n847 = To Variant(anything=w4213) -> (Variant=w4212:variant)
          }
          frame True {
            n848 = Variant To Data(type=w4227, Variant=w4220) -> (data=w4222:bool)  [unwired: 1 in, 1 out]
            n849 = Set Variant Attribute(Variant=w4226, name=w4223, value=w4222, error in=w4224) -> (Variant out=w4225:variant, error out=w4221:errorcluster)  [unwired: 1 out]
          }
        }
      }
      frame "Miscellaneous:# Logical Processors Used" {
        n850 = case shown="True" w4236 {
          tunnel: w4235 -> [w4244 w4249]
          tunnel: w4234 -> [w4243 w4252]
          tunnel: [w4242 w4251] -> w4233
          tunnel: w4232 -> [w4241 w4250]
          tunnel: [w4240 w4248] -> w4231
          tunnel: "# Logical Processors Used" -> [w4239 w4253]
          tunnel: [w4237 w4247] -> w4230
          tunnel: w4229 -> [_ w4247]
          frame False {
            n851 = Get Variant Attribute(Variant=w4243, name=w4244, default value (empty Variant)=w4239, error in=w4241) -> (duplicate Variant=w4242:variant, value=w4238:i32, error out=w4240:errorcluster)  [unwired: 1 out]
            n852 = To Variant(anything=w4238) -> (Variant=w4237:variant)
          }
          frame True {
            n853 = Variant To Data(type=w4253, Variant=w4247) -> (data=w4246:i32)  [unwired: 1 in, 1 out]
            n854 = call "Logical Processors Used.vi"("Set/Get (F)"=TRUE, "# Logical Processor Used"=w4246) -> ()  [unwired: 4 in, 1 out]
            n855 = Set Variant Attribute(Variant=w4252, name=w4249, value=w4246, error in=w4250) -> (Variant out=w4251:variant, error out=w4248:errorcluster)  [unwired: 1 out]
          }
        }
      }
      frame "Miscellaneous:ROI Description Max Characters" {
        n856 = case shown="False" w4262 {
          tunnel: w4261 -> [w4270 w4274]
          tunnel: w4260 -> [w4269 w4277]
          tunnel: [w4268 w4276] -> w4259
          tunnel: w4258 -> [w4267 w4275]
          tunnel: [w4266 w4272] -> w4257
          tunnel: "ROI Description Max Characters" -> [w4265 w4278]
          tunnel: [w4263 w4271] -> w4256
          tunnel: w4255 -> [_ w4271]
          frame False {
            n857 = Get Variant Attribute(Variant=w4269, name=w4270, default value (empty Variant)=w4265, error in=w4267) -> (duplicate Variant=w4268:variant, value=w4264:i32, error out=w4266:errorcluster)  [unwired: 1 out]
            n858 = To Variant(anything=w4264) -> (Variant=w4263:variant)
          }
          frame True {
            n859 = Variant To Data(type=w4278, Variant=w4271) -> (data=w4273:i32)  [unwired: 1 in, 1 out]
            n860 = Set Variant Attribute(Variant=w4277, name=w4274, value=w4273, error in=w4275) -> (Variant out=w4276:variant, error out=w4272:errorcluster)  [unwired: 1 out]
          }
        }
      }
      frame "Miscellaneous:Verbose Error Mode" {
        n861 = case shown="True" w4287 {
          tunnel: w4286 -> [w4295 w4300]
          tunnel: w4285 -> [w4294 w4303]
          tunnel: [w4293 w4302] -> w4284
          tunnel: w4283 -> [w4292 w4301]
          tunnel: [w4291 w4298] -> w4282
          tunnel: "Verbose Error Mode" -> [w4290 w4296]
          tunnel: [w4288 w4297] -> w4281
          tunnel: w4280 -> [_ w4297]
          frame False {
            n862 = Get Variant Attribute(Variant=w4294, name=w4295, default value (empty Variant)=w4290, error in=w4292) -> (duplicate Variant=w4293:variant, value=w4289:bool, error out=w4291:errorcluster)  [unwired: 1 out]
            n863 = To Variant(anything=w4289) -> (Variant=w4288:variant)
          }
          frame True {
            n864 = Variant To Data(type=w4296, Variant=w4297) -> (data=w4299:bool)  [unwired: 1 in, 1 out]
            n865 = Set Variant Attribute(Variant=w4303, name=w4300, value=w4299, error in=w4301) -> (Variant out=w4302:variant, error out=w4298:errorcluster)  [unwired: 1 out]
          }
        }
      }
      frame "Miscellaneous:Transparent Mask Color" {
        n866 = case shown="True" w4312 {
          tunnel: w4311 -> [w4320 w4325]
          tunnel: w4310 -> [w4319 w4328]
          tunnel: [w4318 w4327] -> w4309
          tunnel: w4308 -> [w4317 w4326]
          tunnel: [w4316 w4323] -> w4307
          tunnel: "Transparent Mask Color" -> [w4315 w4321]
          tunnel: [w4313 w4322] -> w4306
          tunnel: w4305 -> [_ w4322]
          frame False {
            n867 = Get Variant Attribute(Variant=w4319, name=w4320, default value (empty Variant)=w4315, error in=w4317) -> (duplicate Variant=w4318:variant, value=w4314:u32, error out=w4316:errorcluster)  [unwired: 1 out]
            n868 = To Variant(anything=w4314) -> (Variant=w4313:variant)
          }
          frame True {
            n869 = Variant To Data(type=w4321, Variant=w4322) -> (data=w4324:u32)  [unwired: 1 in, 1 out]
            n870 = Set Variant Attribute(Variant=w4328, name=w4325, value=w4324, error in=w4326) -> (Variant out=w4327:variant, error out=w4323:errorcluster)  [unwired: 1 out]
          }
        }
      }
    }
  }
  "Error Out" <- w4
  "Variant Data out" <- w3
